vi "AO_master_DM_WFS_v1.vi"() -> ()   [LabVIEW 2018]
uses:
  <userlib>/WaveKit.lib/Controls/Image information.ctl
  <userlib>/WaveKit.lib/Controls/Image general information.ctl
  <userlib>/WaveKit.lib/Controls/Image acquisition information.ctl
  <userlib>/WaveKit.lib/Controls/Point2D.ctl
  <userlib>/WaveKit.lib/Controls/Data alignment enum.ctl
  <userlib>/WaveKit.lib/Controls/StatisticsData.ctl
  <userlib>/WaveKit.lib/Controls/Wavefront Corrector states - ONE.ctl
  <userlib>/WaveKit.lib/Classes/Camera/Camera.lvclass
  <userlib>/WaveKit.lib/Classes/CameraSet/CameraSet.lvclass
  <userlib>/WaveKit.lib/Classes/Image/Image.lvclass
  <userlib>/WaveKit.lib/Classes/Phase/Phase.lvclass
  <userlib>/WaveKit.lib/Controls/HasoSlopes.lvclass
  <userlib>/WaveKit.lib/Controls/Pupil.lvclass
  <userlib>/WaveKit.lib/Classes/WavefrontCorrector/WavefrontCorrector.lvclass
  <userlib>/WaveKit.lib/Classes/WavefrontCorrectorSet/WavefrontCorrectorSet.lvclass
  <userlib>/WaveKit.lib/Classes/HasoEngine/HasoEngine.lvclass
  <userlib>/WaveKit.lib/Controls/SlopesEngineSetup.ctl
  <userlib>/WaveKit.lib/Controls/WavefrontReconstructionMode.ctl
  <vilib>/Utility/file.llb/Read From Spreadsheet File (DBL).vi
  <vilib>/Analysis/1siggen.llb/Ramp Pattern by Delta.vi
  <userlib>/WaveKit.lib/Classes/ModalCoef/ModalCoef.lvclass
  <vilib>/Analysis/NI_AALBase.lvlib
panel:
  in  "Device Status":enum32{"DM", "WFS", "Others"}(tab)=enum."Others"
  out "DM Actuator Values":sgl[](graph)
  out "Initial State":T1[](array[typedef])
  out "ActuatorsNumber":i32
  out "Initial Positions":sgl[](array[numeric])
  out "Final Positions":sgl[](array[numeric])
  in  "Coef Min":dbl=-0.5 min=1.0
  in  "Coef Max":dbl=0.5 min=1.0
  out "Zernike Measured":dbl[](graph)
  out "Phase statistics":T2
  out "Phase values":sgl[][](graph)=[[nan, nan, nan, nan, nan, nan, nan, nan, nan, nan, nan, nan, nan, nan, nan, nan, nan, nan, nan, nan, nan, nan, nan, nan, nan, nan, nan, nan, nan, nan, nan, nan, nan, nan, nan, nan, nan, nan, nan, nan], [nan, nan, nan, nan, nan, nan, nan, nan, nan, nan, nan, nan, nan, nan, nan, nan, nan, nan, nan, nan, nan, nan, nan, nan, nan, nan, nan, nan, nan, nan, nan, nan, nan, nan, nan, nan, nan, nan, nan, nan], [nan, nan, nan, nan, nan, nan, nan, nan, nan, nan, nan, nan, nan, nan, nan, nan, nan, nan, nan, nan, nan, nan, nan, nan, nan, nan, nan, nan, nan, nan, nan, nan, nan, nan, nan, nan, nan, nan, nan, nan], [nan, nan, nan, nan, nan, nan, nan, nan, nan, nan, nan, nan, nan, nan, nan, nan, nan, nan, nan, nan, nan, nan, nan, nan, nan, nan, nan, nan, nan, nan, nan, nan, nan, nan, nan, nan, nan, nan, nan, nan], [nan, nan, nan, nan, nan, nan, nan, nan, nan, nan, nan, nan, nan, nan, -0.14441992, nan, 0.1501734, 0.22490476, 0.2674259, 0.28415325, 0.2792031, 0.2552752, 0.21375881, 0.15405469, nan, nan, nan, nan, nan, nan, nan, nan, nan, nan, nan, nan, nan, nan, nan, nan], [nan, nan, nan, nan, nan, nan, nan, nan, nan, nan, nan, nan, nan, nan, 0.19143742, 0.2795512, 0.33646506, 0.37099743, 0.3877919, 0.3894302, 0.37774685, 0.35447162, 0.3212538, 0.27904776, 0.22675864, 0.15897867, nan, nan, nan, nan, nan, nan, nan, nan, nan, nan, nan, nan, nan, nan], [nan, nan, nan, nan, nan, nan, nan, nan, nan, nan, nan, nan, nan, 0.22618562, 0.290776, 0.33285964, 0.36044422, 0.3767934, 0.38285175, 0.37884915, 0.3652757, 0.3433441, 0.3149789, 0.28229773, 0.2464756, 0.20580466, 0.15268901, 0.06923797, nan, nan, nan, nan, nan, nan, nan, nan, nan, nan, nan, nan], [nan, nan, nan, nan, nan, nan, nan, nan, nan, nan, nan, nan, 0.19992779, 0.24616541, 0.27565512, 0.29675642, 0.31222007, 0.32191983, 0.32467726, 0.31943765, 0.30597392, 0.2852214, 0.25927368, 0.2309889, 0.20308714, 0.17653626, 0.14795627, 0.10568966, 0.024115691, nan, nan, nan, nan, nan, nan, nan, nan, nan, nan, nan], [nan, nan, nan, nan, nan, nan, nan, nan, nan, nan, nan, 0.14862825, 0.18219855, 0.20114602, 0.21551609, 0.22862102, 0.24014233, 0.24817906, 0.2505626, 0.24567793, 0.23295718, 0.21313797, 0.18829979, 0.16161954, 0.1367108, 0.11633411, 0.10019377, 0.081457645, 0.04156301, -0.057204023, nan, nan, nan, nan, nan, nan, nan, nan, nan, nan], [nan, nan, nan, nan, nan, nan, nan, nan, nan, nan, 0.08899155, 0.117771566, 0.12948777, 0.13732892, 0.14631097, 0.15688494, 0.16728252, 0.17497937, 0.17758016, 0.17335457, 0.16157834, 0.14275661, 0.11873307, 0.09261118, 0.06834036, 0.04974218, 0.038678437, 0.031985473, 0.016725859, -0.03676957, nan, nan, nan, nan, nan, nan, nan, nan, nan, nan], [nan, nan, nan, nan, nan, nan, nan, nan, nan, nan, 0.058377307, 0.069048055, 0.0725615, 0.07683456, 0.0840318, 0.09335055, 0.10271386, 0.1097376, 0.11226265, 0.10867052, 0.09812171, 0.08078306, 0.058033932, 0.032565817, 0.008214329, -0.010712444, -0.020921554, -0.022825297, -0.02489755, -0.05023362, -0.14592764, nan, nan, nan, nan, nan, nan, nan, nan, nan], [nan, nan, nan, nan, nan, nan, nan, nan, nan, -0.0018393314, 0.018310271, 0.023098737, 0.024714457, 0.027986258, 0.033823933, 0.041292578, 0.048749834, 0.054400377, 0.056548227, 0.05374936, 0.04499338, 0.029967438, 0.009379062, -0.014759185, -0.03905803, -0.059140373, -0.070816256, -0.0724436, -0.06894927, -0.07806298, -0.1393881, nan, nan, nan, nan, nan, nan, nan, nan, nan], [nan, nan, nan, nan, nan, nan, nan, nan, nan, -0.03322208, -0.017045017, -0.0123043535, -0.010394985, -0.007970343, -0.0042642877, 0.0003761826, 0.005164365, 0.009095938, 0.010986101, 0.009512841, 0.0033822758, -0.008344227, -0.02579559, -0.047820807, -0.071688615, -0.09321856, -0.107681155, -0.11187886, -0.10789668, -0.10908524, -0.14891545, -0.29341945, nan, nan, nan, nan, nan, nan, nan, nan], [nan, nan, nan, nan, nan, nan, nan, nan, nan, nan, -0.043187555, -0.03622458, -0.033755217, -0.03278728, -0.03198469, -0.030707732, -0.028716512, -0.026208155, -0.023933899, -0.023217455, -0.025771504, -0.03328519, -0.04682974, -0.06620631, -0.08943447, -0.1126552, -0.13079928, -0.13944486, -0.13836564, -0.13734597, -0.16491348, -0.2807172, nan, nan, nan, nan, nan, nan, nan, nan], [nan, nan, nan, nan, nan, nan, nan, nan, -0.13038255, -0.08328184, -0.060542934, -0.050779276, -0.048053104, -0.048984695, -0.05126809, -0.053124577, -0.05330209, -0.051303368, -0.04760214, -0.04368073, -0.041799206, -0.04448101, -0.05377527, -0.07043236, -0.09320336, -0.118551016, -0.14113419, -0.15550357, -0.15952203, -0.16009864, -0.18189941, -0.27977645, nan, nan, nan, nan, nan, nan, nan, nan], [nan, nan, nan, nan, nan, nan, nan, nan, -0.15416794, -0.09987456, -0.07151361, -0.05893044, -0.056102008, -0.058817875, -0.063637674, -0.067669004, -0.06878706, -0.06599128, -0.059670344, -0.051622536, -0.044753395, -0.042448726, -0.04769562, -0.062100213, -0.08502676, -0.11315687, -0.14084403, -0.16171429, -0.1720384, -0.17647736, -0.19687745, -0.284868, -0.53908885, -1.12795, nan, nan, nan, nan, nan, nan], [nan, nan, nan, nan, nan, nan, nan, nan, -0.17633308, -0.1131372, -0.07876157, -0.06330658, -0.060116876, -0.063924976, -0.07015394, -0.07493687, -0.07548633, -0.07052183, -0.060539607, -0.047784284, -0.035856243, -0.028966732, -0.030924596, -0.044017438, -0.06802279, -0.099662215, -0.13288532, -0.16044727, -0.17731819, -0.18653797, -0.20820689, -0.29237592, -0.5366785, nan, nan, nan, nan, nan, nan, nan], [nan, nan, nan, nan, nan, nan, nan, nan, -0.19826387, -0.12505035, -0.08430402, -0.06564974, -0.061443567, -0.06527472, -0.07152294, -0.07554153, -0.07411167, -0.0658889, -0.05163869, -0.034133032, -0.017655006, -0.0071354215, -0.007018423, -0.020031396, -0.046107426, -0.08178567, -0.12048963, -0.15415914, -0.17678727, -0.19048853, -0.21480094, -0.2999987, -0.54526997, nan, nan, nan, nan, nan, nan, nan], [nan, nan, nan, nan, nan, nan, nan, nan, -0.2214154, -0.13693352, -0.08914254, -0.06661926, -0.06048554, -0.06317037, -0.0681367, -0.07015528, -0.065784656, -0.053790003, -0.035310905, -0.013662348, 0.0062713036, 0.01901285, 0.01972933, 0.005542416, -0.023349542, -0.06307545, -0.10643376, -0.14466219, -0.17119798, -0.18806857, -0.21562657, -0.30642, -0.5640642, nan, nan, nan, nan, nan, nan, nan], [nan, nan, nan, nan, nan, nan, nan, nan, -0.24718054, -0.14940841, -0.093277775, -0.0658183, -0.056708053, -0.05720259, -0.059951056, -0.05929426, -0.051715773, -0.036192447, -0.014265999, 0.010266874, 0.032073133, 0.04536258, 0.04520398, 0.028878966, -0.0030008797, -0.045963787, -0.092160165, -0.13235793, -0.16002774, -0.17817038, -0.20961209, -0.31157303, -0.5953845, nan, nan, nan, nan, nan, nan, nan], [nan, nan, nan, nan, nan, nan, nan, nan, -0.27748746, -0.16290864, -0.09610232, -0.062047683, -0.048735943, -0.04617936, -0.046241976, -0.042900223, -0.03261665, -0.014586102, 0.009311387, 0.03494107, 0.05674191, 0.068891875, 0.0666744, 0.04783368, 0.0136316735, -0.030755527, -0.0769404, -0.115639456, -0.14119013, -0.15893419, -0.19620675, -0.31774768, nan, nan, nan, nan, nan, nan, nan, nan], [nan, nan, nan, nan, nan, nan, nan, nan, -0.31623095, -0.17884897, -0.09729818, -0.0539262, -0.03469713, -0.028198741, -0.025418447, -0.019910373, -0.008048305, 0.010862423, 0.034768496, 0.05942371, 0.07931873, 0.0889112, 0.08400761, 0.06307276, 0.028166434, -0.014867521, -0.057410896, -0.09080534, -0.111413695, -0.12868427, -0.17697167, -0.3319423, nan, nan, nan, nan, nan, nan, nan, nan], [nan, nan, nan, nan, nan, nan, nan, nan, nan, -0.20170604, -0.09850275, -0.0411539, -0.0131010795, -0.0011654077, 0.0047943285, 0.01185911, 0.023955166, 0.041901454, 0.06374147, 0.08542206, 0.1018104, 0.10796184, 0.10047772, 0.0787158, 0.04554086, 0.007227666, -0.027947046, -0.052963093, -0.06777905, -0.08820889, -0.15871821, nan, nan, nan, nan, nan, nan, nan, nan, nan], [nan, nan, nan, nan, nan, nan, nan, nan, nan, -0.24239759, -0.10614249, -0.026831074, 0.015322472, 0.03581071, 0.046350636, 0.05505173, 0.06651187, 0.08204405, 0.10016226, 0.11737824, 0.12928592, 0.13183476, 0.12261822, 0.10192663, 0.073240966, 0.042765103, 0.017522467, 0.0014635092, -0.0110412, -0.045025453, -0.15884721, nan, nan, nan, nan, nan, nan, nan, nan, nan], [nan, nan, nan, nan, nan, nan, nan, nan, nan, nan, -0.13597216, -0.021381527, 0.04426403, 0.07956008, 0.09847209, 0.110732496, 0.122154154, 0.13505057, 0.14887714, 0.16113368, 0.16849175, 0.16803522, 0.1584293, 0.14075197, 0.118653886, 0.09743117, 0.0815231, 0.06987105, 0.048498146, -0.020404778, nan, nan, nan, nan, nan, nan, nan, nan, nan, nan], [nan, nan, nan, nan, nan, nan, nan, nan, nan, nan, nan, -0.04876471, 0.05625415, 0.117832564, 0.15310521, 0.17423762, 0.18897903, 0.20128381, 0.21210447, 0.22038196, 0.22418612, 0.221881, 0.21311647, 0.19937092, 0.1836943, 0.16922635, 0.15598845, 0.13537171, 0.081669986, nan, nan, nan, nan, nan, nan, nan, nan, nan, nan, nan], [nan, nan, nan, nan, nan, nan, nan, nan, nan, nan, nan, nan, 0.014031529, 0.121263236, 0.18738765, 0.22803904, 0.25380248, 0.2710389, 0.28282017, 0.2899857, 0.29225817, 0.2892868, 0.28139976, 0.26978248, 0.25571787, 0.23844866, 0.21115, 0.15442081, nan, nan, nan, nan, nan, nan, nan, nan, nan, nan, nan, nan], [nan, nan, nan, nan, nan, nan, nan, nan, nan, nan, nan, nan, nan, nan, 0.15212902, 0.2306162, 0.28129596, 0.31381333, 0.33402625, 0.3450995, 0.34855807, 0.34515002, 0.33529556, 0.31882071, 0.29360068, 0.25266168, nan, nan, nan, nan, nan, nan, nan, nan, nan, nan, nan, nan, nan, nan], [nan, nan, nan, nan, nan, nan, nan, nan, nan, nan, nan, nan, nan, nan, nan, nan, 0.1979487, 0.2623494, 0.30271748, 0.32490522, 0.33223343, 0.3261181, 0.30614072, 0.26925305, nan, nan, nan, nan, nan, nan, nan, nan, nan, nan, nan, nan, nan, nan, nan, nan], [nan, nan, nan, nan, nan, nan, nan, nan, nan, nan, nan, nan, nan, nan, nan, nan, nan, nan, nan, nan, nan, nan, nan, nan, nan, nan, nan, nan, nan, nan, nan, nan, nan, nan, nan, nan, nan, nan, nan, nan], [nan, nan, nan, nan, nan, nan, nan, nan, nan, nan, nan, nan, nan, nan, nan, nan, nan, nan, nan, nan, nan, nan, nan, nan, nan, nan, nan, nan, nan, nan, nan, nan, nan, nan, nan, nan, nan, nan, nan, nan], [nan, nan, nan, nan, nan, nan, nan, nan, nan, nan, nan, nan, nan, nan, nan, nan, nan, nan, nan, nan, nan, nan, nan, nan, nan, nan, nan, nan, nan, nan, nan, nan, nan, nan, nan, nan, nan, nan, nan, nan]] caption="Wavefront"
  out "HASO intensity":u32[][](graph)
  in  "error in (no error)":errorcluster
  out "Current error":errorcluster
  out "Output path":path=path "D:/Data"
  out "nb_images (get)":u32=10
  out "exposure_duration_us (get)":u32
  in  "Current status":string="Test1"
  out "HASO ready":bool
  in  "Live Wavefront":bool
  in  "Update DM":bool
  in  "Tab Control":T3(tab)
  in  "Initial haso file":path=path "D:/SystemAlignment/system_aberration_residual_20220406.has"
  in  "interaction matrix file":path=path "D:/SystemAlignment/IM_20220407_1p5sx2_0p5um.aomi"
  in  "DM configuration file":path=path "C:/Program Files (x86)/Imagine Optic/Configuration Files/WaveFrontCorrector_mirao52-e_0326.dat"
  in  "Haso configuration file":path=path "C:/Program Files (x86)/Imagine Optic/Configuration Files/HASO3_first_7364.dat"
  in  "Record Batch Actuator":bool
  in  "Coef value":dbl=0.5 min=1.0
  in  "Idx end":u32=20 min=1
  in  "Idx start":u32=1 min=1
  in  "Subfolder":string="Test1"
  in  "Folder Name":string="Test"
  in  "Net Rp":bool
  in  "Input type":T4(ring)=enum."Zernike Coef"
  in  "Additional Command":bool=TRUE
  in  "Offset command file":path=path "D:/SystemAlignment/system_aberration_20220414.dat"
  in  "Initial offset":bool=TRUE
  in  "Additional file":path=path "D:/SystemAlignment/system_aberration_20191029.dat"
  out "Coef out":sgl[](array[numeric])
  out "Index out":i32[](array[numeric])
  in  "Zern/DM index in":i32[](array[numeric])
  in  "Zern/DM coef in":sgl[](array[numeric])
  in  "idxType":enum16{"Wyant", "ANSI"}(ring)=enum."ANSI"
  in  "Filter":u8[](array[numeric])
  in  "exposure_duration_s (set)":dbl=1.0 min=1.0
  in  "nb_images (set)":u32=1 min=1
  in  "Save File":bool
  in  "File Base Name":string="Test"
  in  "Main Path":path=path "D:/Data"
  in  "Record Response":bool
  in  "Record Batch Zern":bool
  out "Acquisition information":T5={"Image general information"={"Camera serial number"="", "Smearing removed"=FALSE, "Background image removed"=FALSE, "Time Stamp"=timestamp(0 s since 1904-01-01), "Comment"="", "Camera_MAX_Level"=0}, "Acquisition information"={"Exposure duration (us)"=0, "Exposure duration specified (us)"=0, "Gain"=0.0, "Number of summed images"=0, "Trigger type"=""}, "Number of pixels"={"X"=0, "Y"=0}, "Number of bits"=enum."16"}
  in  "Init":bool
  in  "Reset error":bool
  in  "Exit":bool
  in  "Stop HASO":bool
  in  "Start HASO":bool
  # "AO_master_DM_WFS_v1.vi: (last update: 20220405)\nControl deformable mirror and wavefront sensor, check DM response \n1, re-orgnize panel/interface: tap for settings, tab for display and indicators\n2, change camera asynchronous mode to synchronous mode:  see xxxx_v1_SynModeFailure_discarded.vi \n      tried but it does not work when exp time < 0.1s (?), switched back to asyn mode.\n3, add control to flip mirror ( and laser shutter and stage ???): to do\n4, make it more efficient and robust to errors (now: error --> shut down devices)\na) DM ocuppied due to last unnormal exit; b) wavefront measure error: no laser, wrong slopes;\n5, enable DM input by actuators, add DM  actuator index picture, check response of actuators in batch"
  # "Stop HASO: error after Record Batch"
  # "um"
  # "HASO Parameters"
  # "Need to turn OFF live wavefront"
  # "Check DM Response"
  # "Batch Range"
  # "Show in Wyant convention"
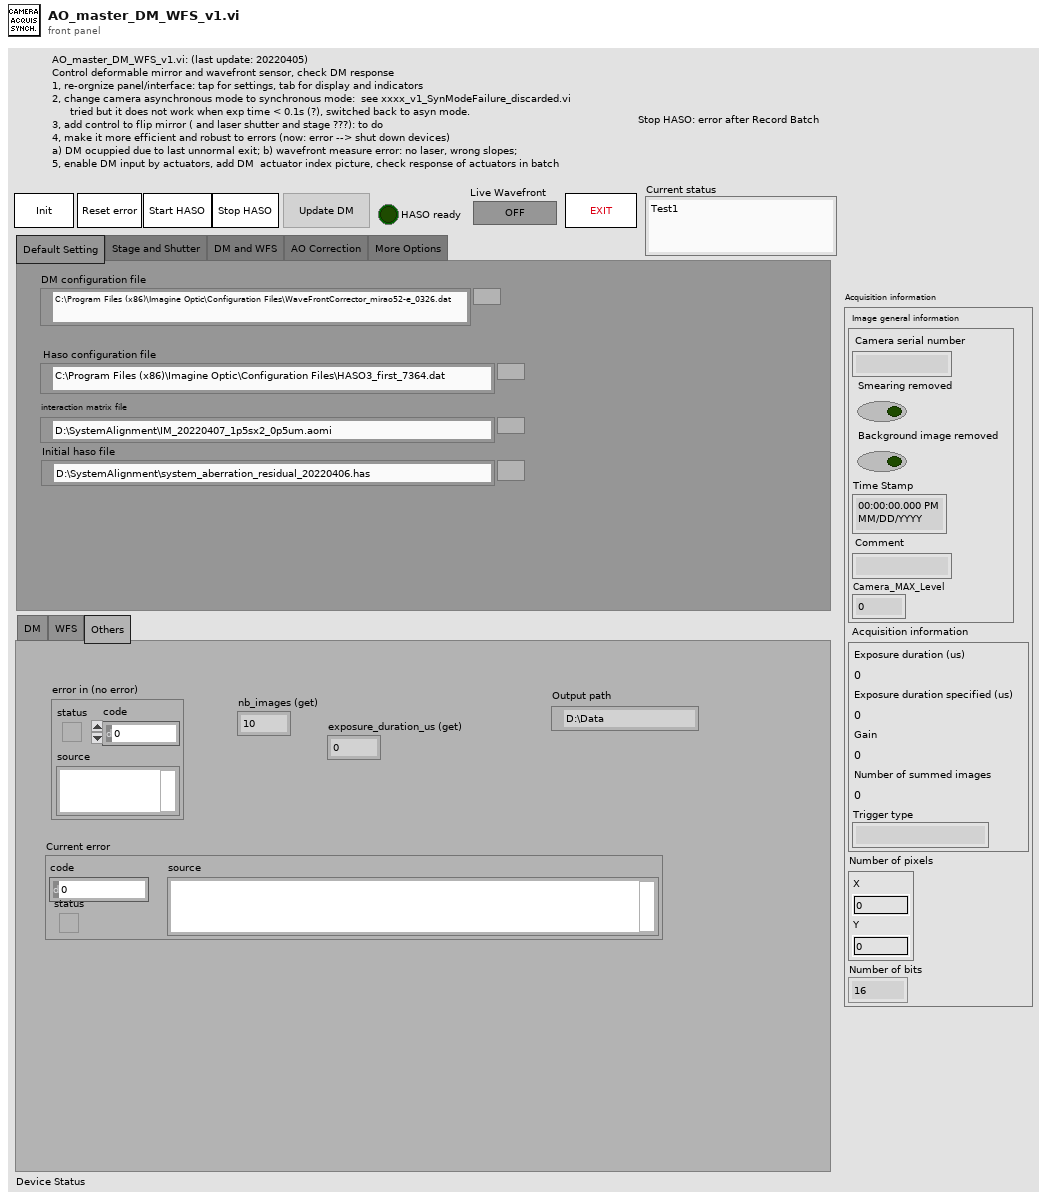
[diagram p1: front panel]
types:
  T1 = typedef "Wavefront Corrector states - ONE.ctl" = cluster{"Max":sgl, "Min":sgl, "Validity":enum16{"valid", "fixed", "invalid"}, "Fixed_Position":sgl}
  T2 = typedef "StatisticsData.ctl" = cluster{"PV":sgl, "RMS":dbl, "Max":sgl, "Min":sgl}
  T3 = enum32{"Default Setting", "Stage and Shutter", "DM and WFS", "AO Correction", "More Options"}
  T4 = enum16{"Zero Input", "Command File", "Zernike Coef", "Zernike File", "DM actuators"}
  T5 = typedef "Image information.ctl" = cluster{"Image general information":T6, "Acquisition information":T7, "Number of pixels":T8, "Number of bits":T9}
  T6 = typedef "Image general information.ctl" = cluster{"Camera serial number":string, "Smearing removed":bool, "Background image removed":bool, "Time Stamp":timestamp, "Comment":string, "Camera_MAX_Level":i32}
  T7 = typedef "Image acquisition information.ctl" = cluster{"Exposure duration (us)":i32, "Exposure duration specified (us)":i32, "Gain":sgl, "Number of summed images":i32, "Trigger type":string}
  T8 = typedef "Point2D.ctl" = cluster{"X":u32, "Y":u32}
  T9 = typedef "Data alignment enum.ctl" = enum16{"8", "16", "32"}
  T10 = typedef "SlopesEngineSetup.ctl" = cluster{"Start sub-aperture":T8, "Pupil average":dbl}
  T11 = typedef "CameraSpecifications.ctl" = cluster{"Grabber name":string, "Camera name":string, "Camera sn":string, "Pixels_um":T12, "Maximum level":u32, "Data alignment":T9, "Is signed":bool, "Acquisition start":T8, "Acquisition length":T8, "MaxFrameRate_Hz":sgl, "Chip type":enum16{"Progressive scan", "Frame transfert"}}
  T12 = typedef "General dimensions definition.ctl" = cluster{"Size":T8, "Step":T13}
  T13 = typedef "Point2Df.ctl" = cluster{"X":sgl, "Y":sgl}
  T14 = typedef "Wavefront Corrector Position.ctl" = sgl[]
  T15 = typedef "WavefrontReconstructionMode.ctl" = enum16{"None", "Modal_Legendre", "Modal_Zernike", "Zonal", "Modal_Zonal_Zernike", "Modal_Zonal_Legendre"}
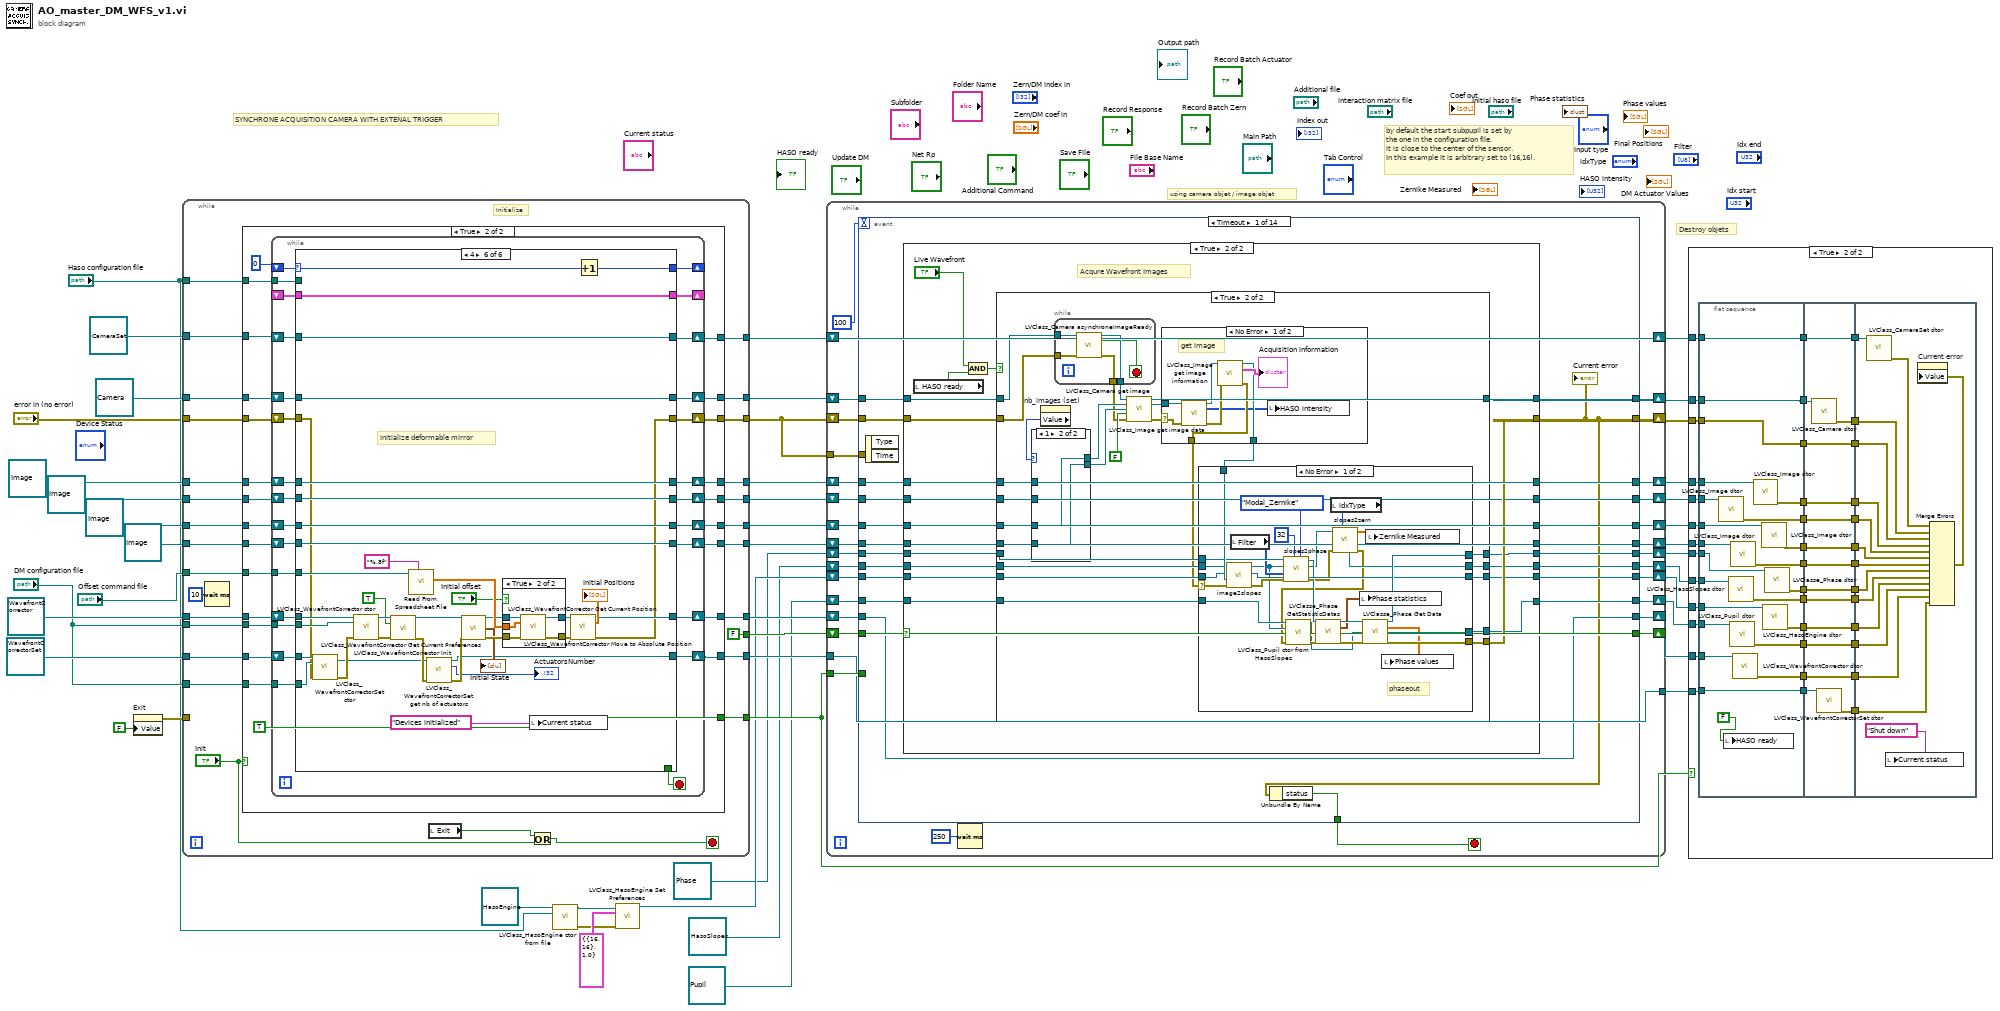
[diagram p0: block diagram]
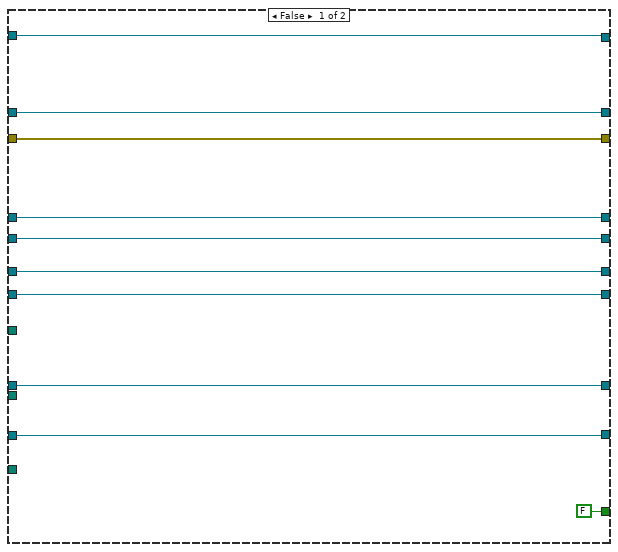
[diagram p3: hidden frame]
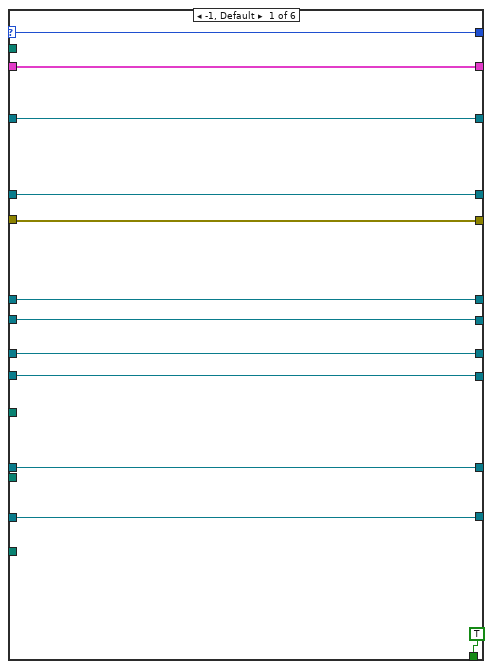
[diagram p4: hidden frame]
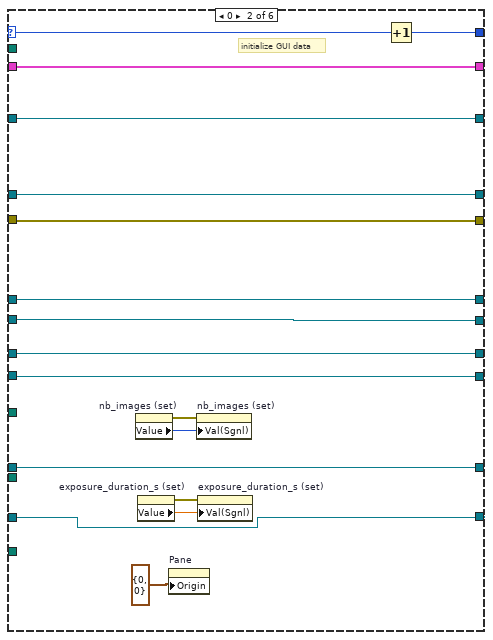
[diagram p5: hidden frame]
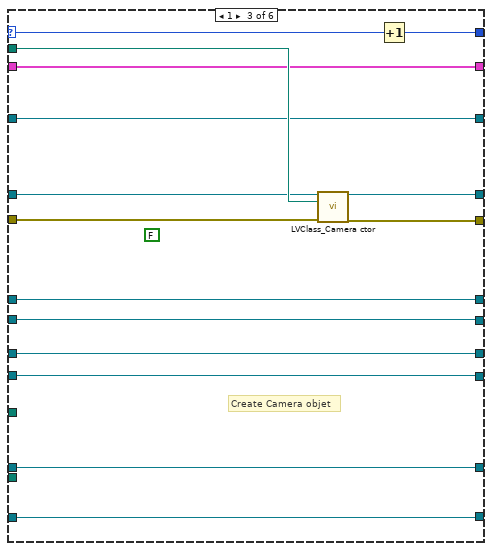
[diagram p6: hidden frame]
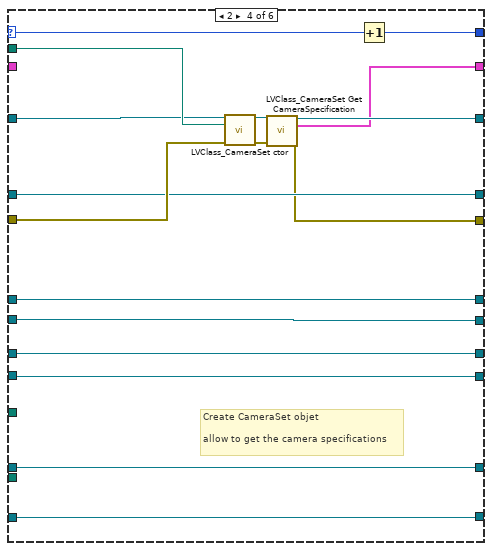
[diagram p7: hidden frame]
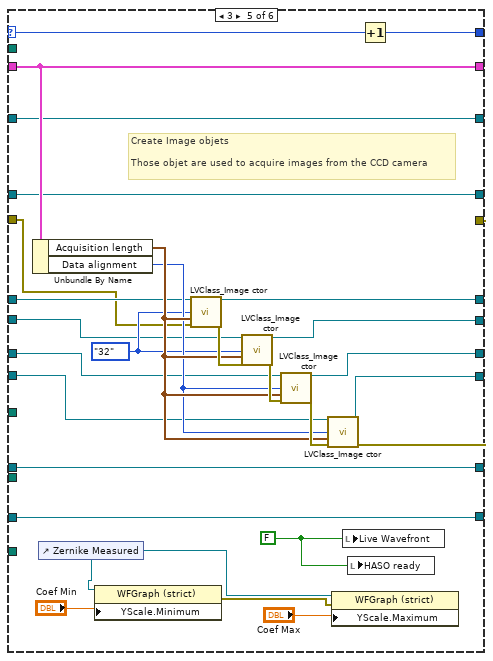
[diagram p8: hidden frame]
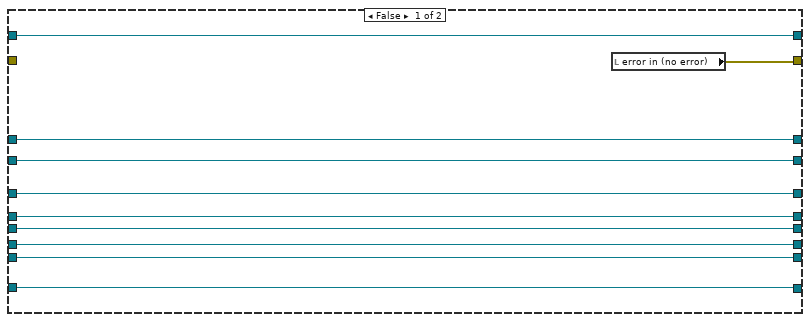
[diagram p10: hidden frame]
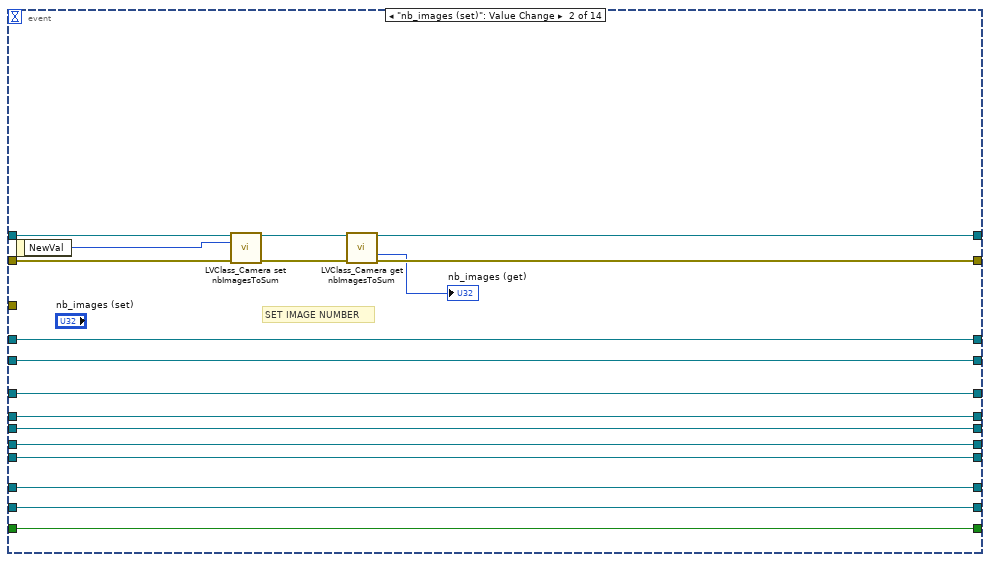
[diagram p15: hidden frame]
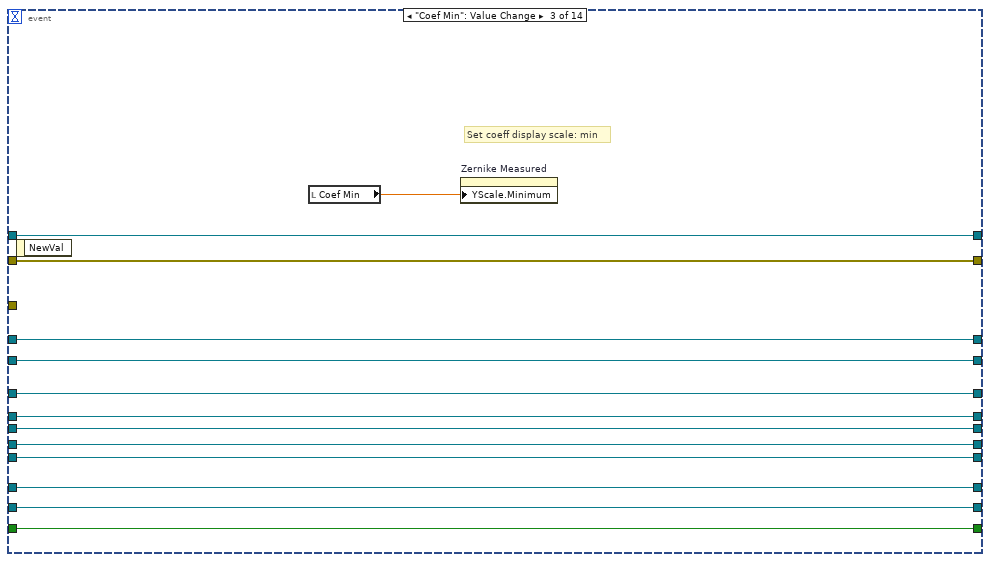
[diagram p16: hidden frame]
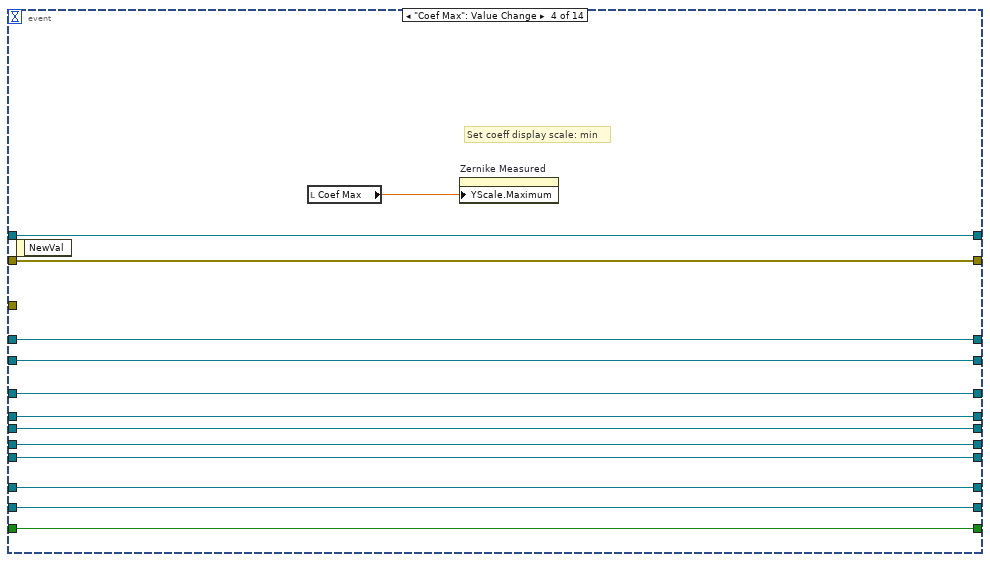
[diagram p17: hidden frame]
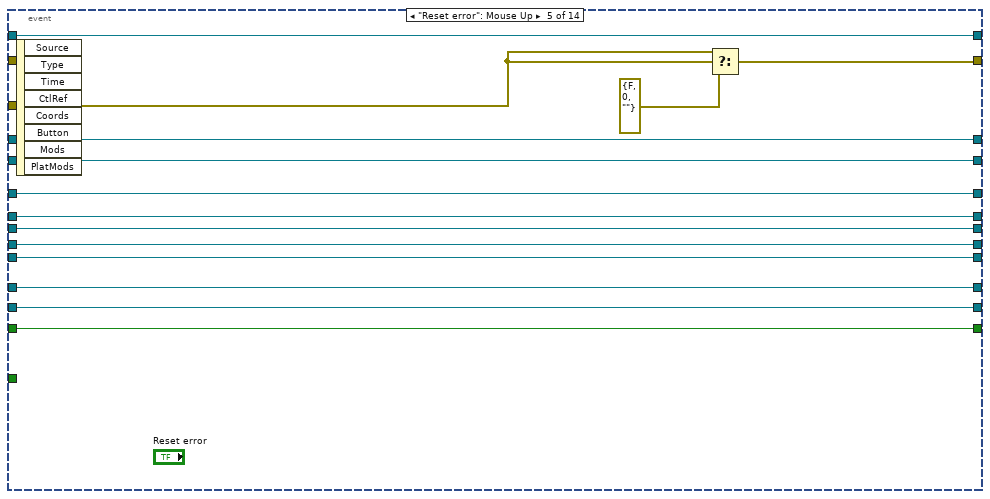
[diagram p18: hidden frame]
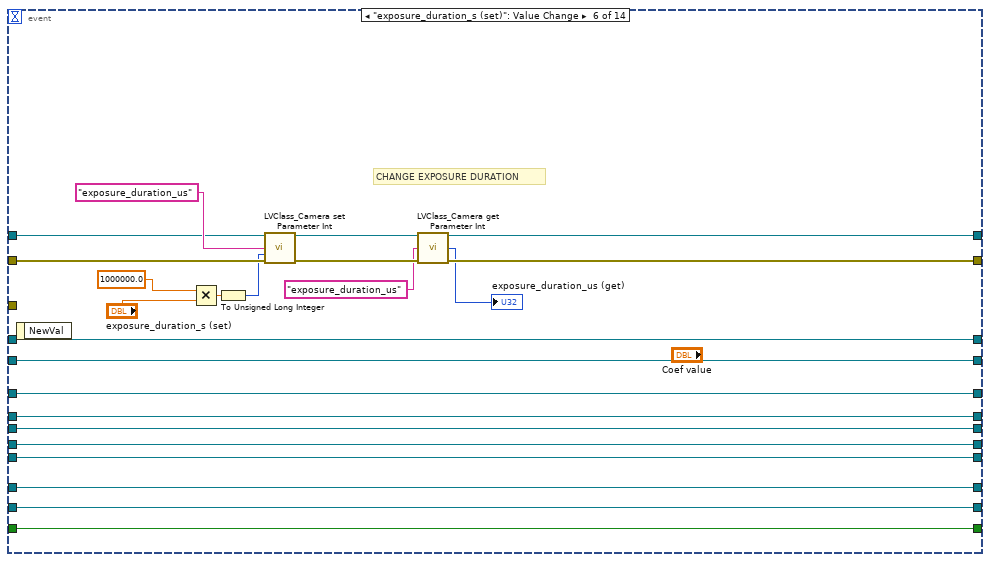
[diagram p19: hidden frame]
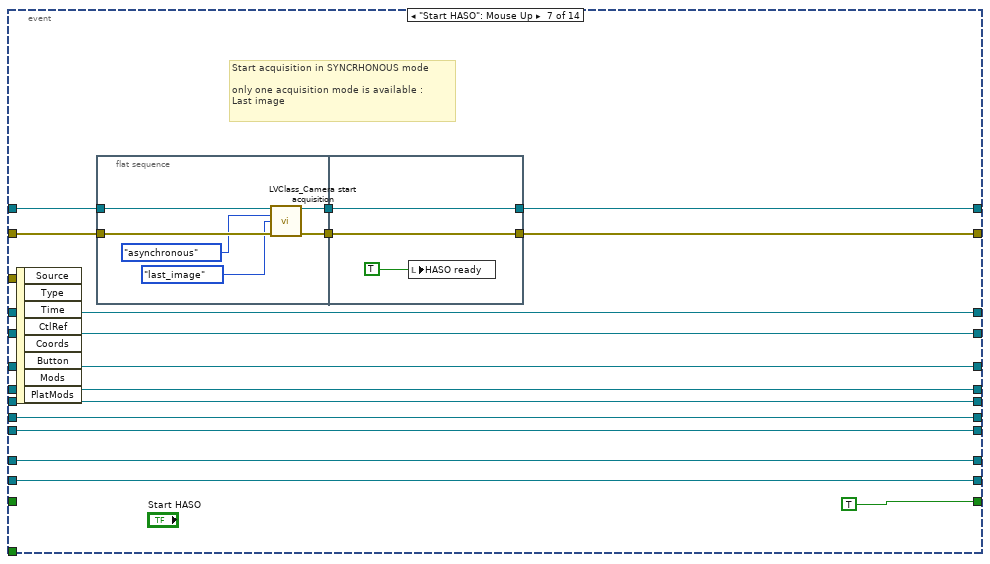
[diagram p20: hidden frame]
diagram:
  # "by default the start subpupil is set by \nthe one in the configuration file. \nit is close to the center of the sensor.\nIn this example it is arbitrary set to (16,16)."
  # "Destroy objets"
  # "using camera objet / image objet"
  # "SYNCHRONE ACQUISITION CAMERA WITH EXTENAL TRIGGER"
  n1 = property on="Exit" class="Bool (strict)"("Value"=FALSE ("Exit")) -> (error out=w23:errorcluster)  [unwired: 2 in, 1 out]
  n2 = while {
    tunnel: [FALSE] -> w39
    tunnel: [w73] -> w38
    tunnel: [w72] -> w37
    tunnel: [w71] -> w36
    tunnel: [w70] -> w35
    tunnel: [w69] -> w34
    tunnel: [w68] -> w33
    tunnel: refnum<class "Camera.lvclass"> refnum ("Camera.lvclass") -> [w67]
    tunnel: refnum<class "CameraSet.lvclass"> refnum ("CameraSet.lvclass") -> [w66]
    tunnel: refnum<class "Image.lvclass"> refnum ("Image in") -> [w65]
    tunnel: refnum<class "Image.lvclass"> refnum ("Image in") -> [w64]
    tunnel: refnum<class "Image.lvclass"> refnum ("Image in") -> [w63]
    tunnel: refnum<class "Image.lvclass"> refnum ("Image in") -> [w62]
    tunnel: "error in (no error)" -> [w61]
    tunnel: [w60] -> w26
    tunnel: [w58] -> w25
    tunnel: w23 -> [_]
    tunnel: "Haso configuration file" -> [w54]
    tunnel: "Offset command file" -> [w53]
    tunnel: refnum<class "WavefrontCorrectorSet.lvclass"> refnum ("WavefrontCorrectorSet in") -> [w52]
    tunnel: "DM configuration file" -> [w51]
    tunnel: refnum<class "WavefrontCorrector.lvclass"> refnum ("WavefrontCorrector in") -> [w50]
    tunnel: "DM configuration file" -> [w49]
    tunnel: [w48] -> w18
    tunnel: [w47] -> w17
    stop <- w55 stop-if-true
    # "Initialize"
    n3 = Wait (ms)(milliseconds to wait=u32 10) -> ()  [unwired: 1 out]
    n4 = case shown="True" "Init" {
      tunnel: [w84 w108] -> w73
      tunnel: [w83 w107] -> w72
      tunnel: [w81 w106] -> w71
      tunnel: [w80 w105] -> w70
      tunnel: [w79 w104] -> w69
      tunnel: [w78 w103] -> w68
      tunnel: w67 -> [w84 w102]
      tunnel: w66 -> [w83 w100]
      tunnel: w65 -> [w81 w99]
      tunnel: w64 -> [w80 w98]
      tunnel: w63 -> [w79 w97]
      tunnel: w62 -> [w78 w96]
      tunnel: w61 -> [w82 w95]
      tunnel: [w82 w94] -> w60
      tunnel: [FALSE TRUE] -> w58
      tunnel: w54 -> [_ w92]
      tunnel: w53 -> [_ w91]
      tunnel: w52 -> [w75 w85]
      tunnel: w51 -> [_ w90]
      tunnel: w50 -> [w76 w86]
      tunnel: w49 -> [_ w89]
      tunnel: [w76 w88] -> w48
      tunnel: [w75 w87] -> w47
      frame False {
      }
      frame True {
        n5 = while {
          tunnel: w92 -> [w133]
          shift-right: [w135] -> w108
          shift-left: w102 -> [w127]
          shift-right: [w117] -> _
          shift-left: 0 -> [w116]
          shift-right: [w134] -> w107
          shift-left: w100 -> [w126]
          shift-right: [w125] -> _
          shift-left: _ -> [w123]
          shift-right: [w132] -> w106
          shift-left: w99 -> [w124]
          shift-right: [w131] -> w105
          shift-left: w98 -> [w122]
          shift-right: [w130] -> w104
          shift-left: w97 -> [w120]
          shift-right: [w129] -> w103
          shift-left: w96 -> [w121]
          shift-right: [w128] -> w94
          shift-left: w95 -> [w118]
          tunnel: w91 -> [w115]
          tunnel: w90 -> [w114]
          tunnel: w89 -> [w113]
          shift-right: [w112] -> w88
          shift-left: w86 -> [w110]
          shift-right: [w111] -> w87
          shift-left: w85 -> [w109]
          stop <- w119 stop-if-true
          n6 = case shown="4" w116 {
            tunnel: [w147 w151 w179 w189 w211 w261] -> w135
            tunnel: w133 -> [_ _ w178 w193 _ _]
            tunnel: [w146 w155 w176 w194 w212 w260] -> w134
            tunnel: [w139 w156 w170 w184 w218 w255] -> w132
            tunnel: [w140 w157 w171 w185 w217 w256] -> w131
            tunnel: [w141 w158 w172 w186 w216 w257] -> w130
            tunnel: [w142 w159 w173 w187 w215 w258] -> w129
            tunnel: [w143 w150 w175 w188 w214 w229] -> w128
            selector: w116 -> [w138 w153 w168 w183 w206 w227]
            tunnel: w127 -> [w147 w151 w177 w189 w211 w261]
            tunnel: w126 -> [w146 w155 w176 w192 w212 w260]
            tunnel: [w144 w152 w174 w191 w213 w259] -> w125
            tunnel: w124 -> [w139 w156 w170 w184 w210 w255]
            tunnel: w123 -> [w144 w152 w174 _ w213 w259]
            tunnel: w122 -> [w140 w157 w171 w185 w209 w256]
            tunnel: w121 -> [w142 w159 w173 w187 w208 w258]
            tunnel: w120 -> [w141 w158 w172 w186 w207 w257]
            tunnel: [TRUE _ _ _ _ _] -> w119
            tunnel: w118 -> [w143 w150 w167 w190 w204 w230]
            tunnel: [w138 w154 w169 w182 w205 w226] -> w117
            tunnel: w115 -> [_ _ _ _ _ w237]
            tunnel: w109 -> [w136 w148 w165 w180 w202 w235]
            tunnel: w114 -> [_ _ _ _ _ w234]
            tunnel: w110 -> [w137 w149 w166 w181 w203 w233]
            tunnel: w113 -> [_ _ _ _ _ w232]
            tunnel: [w137 w149 w166 w181 w203 w231] -> w112
            tunnel: [w136 w148 w165 w180 w202 w228] -> w111
            frame -1, Default {
            }
            frame 0 {
              # "initialize GUI data"
              n7 = property on="nb_images (set)" class="DigNum (strict)"() -> (error out=w164:errorcluster, "Value"=w163:u32)  [unwired: 2 in, 1 out]
              n8 = property on="exposure_duration_s (set)" class="DigNum (strict)"() -> (error out=w160:errorcluster, "Value"=w162:dbl)  [unwired: 2 in, 1 out]
              n9 = property on="Pane" class="Pane"("Origin"=cluster{"Horizontal":i16, "Vertical":i16} {"Horizontal"=0, "Vertical"=0} ("Front Panel Window:Origin")) -> ()  [unwired: 2 in, 2 out]
              n10 = property on="nb_images (set)" class="DigNum (strict)"(error in=w164, "Val(Sgnl)"=w163) -> ()  [unwired: 1 in, 2 out]
              n11 = property on="exposure_duration_s (set)" class="DigNum (strict)"(error in=w160, "Val(Sgnl)"=w162) -> ()  [unwired: 1 in, 2 out]
              n12 = Increment(x=w153) -> (x+1=w154:i32)
            }
            frame 1 {
              (unwired) FALSE ("Acq required")
              # "Create Camera objet"
              n13 = call <userlib>:"LVClass_Camera ctor.vi"("Camera"=w177, "Configuration file path"=w178, "error in (no error)"=w167) -> ("Camera (new)"=w179:refnum<class "Camera.lvclass">, "error out"=w175:errorcluster)  [unwired: 11 in]
              n14 = Increment(x=w168) -> (x+1=w169:i32)
            }
            frame 2 {
              # "Create CameraSet objet\n\nallow to get the camera specifications"
              n15 = call <userlib>:"LVClass_CameraSet ctor.vi"("CameraSet.lvclass"=w192, "Configuration file path"=w193, "error in (no error)"=w190) -> ("CameraSet.lvclass"=w196:refnum<class "CameraSet.lvclass">, "error out"=w195:errorcluster)  [unwired: 11 in]
              n16 = call <userlib>:"LVClass_CameraSet Get CameraSpecification.vi"("CameraSet.lvclass"=w196, "error in (no error)"=w195) -> ("CameraSet.lvclass"=w194:refnum<class "CameraSet.lvclass">, "Camera Config"=w191:T11, "error out"=w188:errorcluster)  [unwired: 11 in]
              n17 = Increment(x=w183) -> (x+1=w182:i32)
            }
            frame 3 {
              w201 = FALSE
              w219 = Data_alignment_enum."32" ("Data alignment")
              # "Create Image objets\n\nThose objet are used to acquire images from the CCD camera"
              n18 = Unbundle By Name(w213) -> ("Acquisition length"=w221:T8, "Data alignment"=w220:T9)
              n19 = control-ref of="Zernike Measured"() -> (w198:refnum<vi>)
              n20 = property on="Property Node" class="WFGraph (strict)"(reference=w198, "YScale.Minimum"="Coef Min") -> (error out=w197:errorcluster)  [unwired: 1 in, 1 out]
              n21 = call <userlib>:"LVClass_Image ctor.vi"("Image in"=w210, "Data alignment"=w219, "Size"=w221, "error in (no error)"=w204) -> ("Image out"=w218:refnum<class "Image.lvclass">, "error out"=w222:errorcluster)  [unwired: 10 in]
              n22 = call <userlib>:"LVClass_Image ctor.vi"("Image in"=w209, "Data alignment"=w219, "Size"=w221, "error in (no error)"=w222) -> ("Image out"=w217:refnum<class "Image.lvclass">, "error out"=w223:errorcluster)  [unwired: 10 in]
              n23 = call <userlib>:"LVClass_Image ctor.vi"("Image in"=w207, "Data alignment"=w220, "Size"=w221, "error in (no error)"=w223) -> ("Image out"=w216:refnum<class "Image.lvclass">, "error out"=w224:errorcluster)  [unwired: 10 in]
              n24 = call <userlib>:"LVClass_Image ctor.vi"("Image in"=w208, "Data alignment"=w220, "Size"=w221, "error in (no error)"=w224) -> ("Image out"=w215:refnum<class "Image.lvclass">, "error out"=w214:errorcluster)  [unwired: 10 in]
              n25 = property on="Property Node" class="WFGraph (strict)"(reference=w198, error in=w197, "YScale.Maximum"="Coef Max") -> ()  [unwired: 2 out]
              n26 = local write "Live Wavefront"(w201) -> ()
              n27 = local write "HASO ready"(w201) -> ()
              n28 = Increment(x=w206) -> (x+1=w205:i32)
            }
            frame 4 {
              (unwired) "DM "
              (unwired) "DM "
              # "Initialize deformable mirror"
              n29 = call <userlib>:"LVClass_WavefrontCorrectorSet ctor.vi"("WavefrontCorrectorSet in"=w235, "PathToWavefrontCorrectorSetupFile"=w234, "error in (no error)"=w230) -> ("WavefrontCorrectorSet out"=w242:refnum<class "WavefrontCorrectorSet.lvclass">, "error out"=w251:errorcluster)  [unwired: 11 in]
              n30 = call <userlib>:"LVClass_WavefrontCorrector ctor.vi"("WavefrontCorrector in"=w233, "PathToWavefrontCorrectorSetupFile"=w232, "error in (no error)"=w251) -> ("WavefrontCorrector out"=w239:refnum<class "WavefrontCorrector.lvclass">, "error out"=w240:errorcluster)  [unwired: 11 in]
              n31 = call <userlib>:"LVClass_WavefrontCorrector Init.vi"("WavefrontCorrector in"=w239, "set_init_state_from_config_file"=TRUE, "error in (no error)"=w240) -> ("WavefrontCorrector out"=w243:refnum<class "WavefrontCorrector.lvclass">, "error out"=w252:errorcluster)  [unwired: 11 in]
              n32 = call-poly <vilib>:"Read From Spreadsheet File.vi"("format (%.3f)"="%.8f", "file path (dialog if empty)"=w237) -> ("first row"=w254:dbl[])  [unwired: 5 in, 4 out]
              n33 = call <userlib>:"LVClass_WavefrontCorrectorSet get nb of actuators.vi"("WavefrontCorrectorSet in"=w242, "error in (no error)"=w252) -> ("WavefrontCorrectorSet out"=w228:refnum<class "WavefrontCorrectorSet.lvclass">, "ActuatorsNumber"=→"ActuatorsNumber":i32, "error out"=w253:errorcluster)  [unwired: 11 in]
              n34 = call <userlib>:"LVClass_WavefrontCorrector Get Current Preferences.vi"("WavefrontCorrector in"=w243, "error in (no error)"=w253) -> ("WavefrontCorrector out"=w248:refnum<class "WavefrontCorrector.lvclass">, "Mirror preferences.Wavefront Corrector State"=→"Initial State":T1[], "error out"=w249:errorcluster)  [unwired: 10 in, 1 out]
              n35 = case shown="True" "Initial offset" {
                tunnel: w254 -> [_ w268]
                tunnel: [w263 w267] -> w246
                tunnel: [w262 w266] -> w247
                tunnel: w248 -> [w263 w265]
                tunnel: w249 -> [w262 w264]
                frame False {
                }
                frame True {
                  n36 = call <userlib>:"LVClass_WavefrontCorrector Move to Absolute Position.vi"("WavefrontCorrector in"=w265, "Absolute Positions"=w268, "error in (no error)"=w264) -> ("WavefrontCorrector out"=w267:refnum<class "WavefrontCorrector.lvclass">, "error out"=w266:errorcluster)  [unwired: 11 in]
                }
              }
              n37 = local write "Current status"("Devices initialized") -> ()
              n38 = call <userlib>:"LVClass_WavefrontCorrector Get Current Position.vi"("WavefrontCorrector in"=w246, "error in (no error)"=w247) -> ("WavefrontCorrector out"=w231:refnum<class "WavefrontCorrector.lvclass">, "Wavefront Corrector Position"=→"Initial Positions":T14, "error out"=w229:errorcluster)  [unwired: 11 in]
              n39 = Increment(x=w227) -> (x+1=w226:i32)
            }
          }
        }
      }
    }
    n40 = local read "Exit"() -> (w57:bool)
    n41 = Or(x=w57, y="Init") -> (x .or. y?=w55:bool)
  }
  n42 = call <userlib>:"LVClass_HasoEngine ctor from file.vi"("HasoEngine in"=refnum<class "HasoEngine.lvclass"> refnum, "Configuration file path"="Haso configuration file") -> ("HasoEngine out"=w14:refnum<class "HasoEngine.lvclass">, "error out"=w15:errorcluster)  [unwired: 12 in]
  n43 = call <userlib>:"LVClass_HasoEngine Set Preferences.vi"("HasoEngine in"=w14, "Slopes_HasoEngine_Setup"=T10 {"Start sub-aperture"={"X"=16, "Y"=16}, "Pupil average"=1.0}, "error in (no error)"=w15) -> ("HasoEngine out"=w11:refnum<class "HasoEngine.lvclass">)  [unwired: 11 in, 1 out]
  n44 = while {
    shift-right: [w296] -> w46
    shift-left: w26 -> [w298]
    shift-right: [w294] -> w45
    shift-left: w38 -> [w295]
    shift-right: [w288] -> w44
    shift-left: w36 -> [w293]
    shift-right: [w287] -> w43
    shift-left: w35 -> [w292]
    shift-right: [w286] -> w42
    shift-left: w34 -> [w291]
    shift-right: [w285] -> w41
    shift-left: w33 -> [w290]
    shift-right: [w284] -> _
    shift-left: w39 -> [w289]
    shift-right: [w283] -> w40
    shift-left: w37 -> [w283]
    tunnel: w26 -> [w282]
    tunnel: w25 -> [w281]
    tunnel: w17 -> [w270]
    shift-right: [w278] -> w10
    shift-left: refnum<class "HasoSlopes.lvclass"> refnum ("HasoSlopes in") -> [w277]
    shift-right: [w276] -> w5
    shift-left: w11 -> [w279]
    shift-right: [w273] -> w6
    shift-left: refnum<class "Phase.lvclass"> refnum ("Phase in") -> [w275]
    shift-right: [w272] -> w4
    shift-left: refnum<class "Pupil.lvclass"> refnum ("Pupil in") -> [w274]
    tunnel: [w270] -> w3
    shift-right: [w269] -> w2
    shift-left: w18 -> [w271]
    stop <- w297 stop-if-true
    n45 = event shown="[0] Timeout" {
      selector: _ -> [_ _ _ _ _ _ _ _ _ _ _ _ _ _]
      dyn-events: _ -> [_ _ _ _ _ _ _ _ _ _ _ _ _ _]
      timeout: 100 -> [_ _ _ _ _ _ _ _ _ _ _ _ _ _]
      tunnel: w298 -> [w314 w452 w455 w468 _ w515 w531 w549 w577 w711 w1282 w1825 _ w2593]
      tunnel: [w300 _ _ _ _ _ _ _ w578 w712 w1283 w1826 "Exit" TRUE ("Exit")] -> w297
      tunnel: [w301 w450 w455 w468 w486 w510 w529 w555 w576 w710 w1281 w1824 w2577 w2598] -> w296
      tunnel: w295 -> [w319 w451 w456 w469 w488 w514 w532 w556 w572 w699 w1270 w1813 w2578 w2600]
      tunnel: [w318 w449 w456 w469 w488 w511 w530 w557 w572 w699 w1270 w1813 w2576 w2599] -> w294
      tunnel: w293 -> [w322 w442 w463 w476 w490 w504 w527 w551 w588 w706 w1277 w1820 w2572 w2594]
      tunnel: w292 -> [w321 w443 w464 w477 w491 w505 w526 w552 w587 w705 w1276 w1819 w2573 w2595]
      tunnel: w291 -> [w320 w444 w465 w478 w492 w506 w525 w553 w586 w704 w1275 w1818 w2574 w2596]
      tunnel: w290 -> [w315 w445 w466 w479 w493 w507 w524 w554 w585 w703 w1274 w1817 w2575 w2597]
      tunnel: w289 -> [w311 w441 w462 w475 w489 w503 _ _ w573 w708 w1279 w1822 _ _]
      tunnel: [w317 w442 w463 w476 w490 w504 w527 w551 w588 w706 w1277 w1820 w2572 w2594] -> w288
      tunnel: [w316 w443 w464 w477 w491 w505 w526 w552 w587 w705 w1276 w1819 w2573 w2595] -> w287
      tunnel: [w313 w444 w465 w478 w492 w506 w525 w553 w586 w704 w1275 w1818 w2574 w2596] -> w286
      tunnel: [w312 w445 w466 w479 w493 w507 w524 w554 w585 w703 w1274 w1817 w2575 w2597] -> w285
      tunnel: [w311 w441 w462 w475 w489 w503 TRUE FALSE w573 w708 w1279 w1822 FALSE FALSE] -> w284
      tunnel: w282 -> [_ _ _ _ w485 _ _ _ _ _ _ _ _ _]
      tunnel: w281 -> [_ _ _ _ _ _ _ _ _ _ _ _ w2570 _]
      tunnel: w277 -> [w310 w439 w460 w473 w483 w497 w522 w547 w569 w701 w1272 w1815 w2568 w2590]
      tunnel: w279 -> [w309 w438 w459 w472 w482 w496 w521 w546 w568 w700 w1271 w1814 w2567 w2589]
      tunnel: [w308 w439 w460 w473 w483 w497 w522 w547 w569 w698 w1269 w1812 w2568 w2590] -> w278
      tunnel: [w307 w438 w459 w472 w482 w496 w521 w546 w568 w700 w1271 w1814 w2567 w2589] -> w276
      tunnel: w275 -> [w306 w440 w461 w474 w484 w498 w523 w548 w570 w702 w1273 w1816 w2569 w2591]
      tunnel: w274 -> [w305 w437 w458 w471 w481 w495 w520 w545 w567 w696 w1267 w1810 w2566 w2588]
      tunnel: [w304 w440 w461 w474 w484 w498 w523 w548 w570 w697 w1268 w1811 w2569 w2591] -> w273
      tunnel: [w303 w437 w458 w471 w481 w495 w520 w545 w567 w695 w1266 w1809 w2566 w2588] -> w272
      tunnel: w271 -> [w302 w436 w457 w470 w480 w494 w519 w544 w575 w709 w1280 w1823 w2565 w2587]
      tunnel: [w302 w436 w457 w470 w480 w494 w519 w544 w571 w707 w1278 w1821 w2565 w2587] -> w269
      event Timeout {
        n46 = event-data() -> ()  [unwired: 1 in, 2 out]
        n47 = case shown="True" w311 {
          tunnel: [w323 w348] -> w301
          tunnel: w322 -> [w332 w351]
          tunnel: [w332 w351] -> w317
          tunnel: [w328 w347] -> w316
          tunnel: w320 -> [w331 w350]
          tunnel: w315 -> [w330 w349]
          tunnel: [w331 w350] -> w313
          tunnel: [w330 w349] -> w312
          tunnel: w321 -> [w328 w347]
          tunnel: w319 -> [w329 w345]
          tunnel: [w329 w346] -> w318
          tunnel: w314 -> [_ w344]
          tunnel: w310 -> [w326 w343]
          tunnel: w309 -> [w325 w342]
          tunnel: [w326 w341] -> w308
          tunnel: [w325 w340] -> w307
          tunnel: w306 -> [w327 w339]
          tunnel: w305 -> [w324 w338]
          tunnel: [w327 w337] -> w304
          tunnel: [w324 w336] -> w303
          frame False {
            n48 = local read "error in (no error)"() -> (w323:errorcluster)
          }
          frame True {
            # "Acqure Wavefront Images"
            n49 = local read "HASO ready"() -> (w333:bool)
            n50 = And(x="Live Wavefront", y=w333) -> (x .and. y?=w335:bool)
            n51 = case shown="True" w335 {
              tunnel: w351 -> [_ w381]
              tunnel: w350 -> [_ w380]
              tunnel: w349 -> [_ w379]
              tunnel: [w352 w376] -> w348
              tunnel: w347 -> [_ w373]
              tunnel: [w357 w372] -> w346
              tunnel: w345 -> [w357 w358]
              tunnel: w344 -> [w352 w359]
              tunnel: w343 -> [w355 w371]
              tunnel: w342 -> [w354 w370]
              tunnel: [w355 w369] -> w341
              tunnel: [w354 w368] -> w340
              tunnel: w339 -> [w356 w367]
              tunnel: w338 -> [w353 w366]
              tunnel: [w356 w365] -> w337
              tunnel: [w353 w364] -> w336
              frame False {
              }
              frame True {
                n52 = property on="nb_images (set)" class="DigNum (strict)"() -> ("Value"=w382:u32)  [unwired: 2 in, 2 out]
                n53 = case shown="1" w382 {
                  tunnel: [w433 w435] -> w383
                  tunnel: w373 -> [w432 _]
                  tunnel: w381 -> [w433 _]
                  tunnel: [w432 w434] -> w378
                  tunnel: w380 -> [_ w435]
                  tunnel: w379 -> [_ w434]
                  frame 2, Default {
                  }
                  frame 1 {
                  }
                }
                n54 = while {
                  tunnel: w358 -> [w388]
                  tunnel: [w387] -> w360
                  tunnel: w359 -> [w385]
                  tunnel: [w384] -> w361
                  stop <- w386 stop-if-true
                  n55 = call <userlib>:"LVClass_Camera asynchroneImageReady.vi"("Camera in"=w388, "error in (no error)"=w385) -> ("Camera out"=w387:refnum<class "Camera.lvclass">, "ready"=w386:bool, "error out"=w384:errorcluster)  [unwired: 11 in]
                }
                n56 = call <userlib>:"LVClass_Camera get image.vi"("Camera in"=w360, "Image"=w383, "Image RAW"=w378, "remove_background"=FALSE, "error in (no error)"=w361) -> ("Camera out"=w372:refnum<class "Camera.lvclass">, "Image (dup)"=w377:refnum<class "Image.lvclass">, "error out"=w374:errorcluster)  [unwired: 7 in, 1 out]
                n57 = case shown="No Error" w374 {
                  selector: w374 -> [w429 w430]
                  tunnel: w377 -> [w426 w431]
                  tunnel: [w424 w431] -> w363
                  tunnel: [w423 w430] -> w362
                  frame No Error {
                    # "get image"
                    n58 = call <userlib>:"LVClass_Image get image data.vi"("Image in"=w426, "error in (no error)"=w429) -> ("Image out"=w428:refnum<class "Image.lvclass">, "Image data out"=w422:u32[][], "error out"=w427:errorcluster)  [unwired: 11 in]
                    n59 = call <userlib>:"LVClass_Image get image information.vi"("Image in"=w428, "error in (no error)"=w427) -> ("Image out"=w424:refnum<class "Image.lvclass">, "Acquisition information"=→"Acquisition information":T5, "error out"=w423:errorcluster)  [unwired: 11 in]
                    n60 = local write "HASO intensity"(w422) -> ()
                  }
                  frame Error {
                  }
                }
                n61 = case shown="No Error" w362 {
                  selector: w362 -> [w409 w421]
                  tunnel: [w415 w421] -> w376
                  tunnel: w363 -> [w408 _]
                  tunnel: [w413 w417] -> w364
                  tunnel: [w412 w420] -> w365
                  tunnel: w371 -> [w405 w419]
                  tunnel: w370 -> [w404 w418]
                  tunnel: [w393 w419] -> w369
                  tunnel: [w403 w418] -> w368
                  tunnel: w367 -> [w401 w420]
                  tunnel: w366 -> [w399 w417]
                  frame No Error {
                    # "phaseout"
                    n62 = call "image2slopes.vi"("error in (no error)"=w409, "Image in"=w408, "HasoEngine in"=w404, "HasoSlopes in"=w405) -> ("error out"=w402:errorcluster, "HasoEngine out"=w403:refnum<class "HasoEngine.lvclass">, "HasoSlopes out"=w395:refnum<class "HasoSlopes.lvclass">)  [unwired: 4 in, 1 out]
                    n63 = local read "Filter"() -> (w398:u8[])
                    n64 = call "slopes2phase.vi"("TypePhase"=WavefrontReconstructionMode."Modal_Zernike", "Number of coefficients"=u8 32, "error in (no error)"=w402, "Filter"=w398, "HasoSlopes in"=w395, "Phase in"=w401) -> ("error out"=w392:errorcluster, "HasoSlopes out"=w394:refnum<class "HasoSlopes.lvclass">, "Phase out"=w400:refnum<class "Phase.lvclass">)  [unwired: 3 in]
                    n65 = local read "idxType"() -> (w389:enum16{"Wyant", "ANSI"})
                    n66 = call "slopes2zern.vi"("HasoSlopes in"=w394, "error in (no error)"=w392, "idxType"=w389) -> ("HasoSlopes out"=w393:refnum<class "HasoSlopes.lvclass">, "Zernike Coefficients"=w390:dbl[], "error out"=w391:errorcluster)  [unwired: 3 in, 2 out]
                    n67 = call <userlib>:"LVClass_Pupil ctor from HasoSlopes.vi"("Pupil in"=w399, "HasoSlopes.lvclass"=w395, "error in (no error)"=w391) -> ("Pupil out"=w410:refnum<class "Pupil.lvclass">, "error out"=w411:errorcluster)  [unwired: 11 in]
                    n68 = call <userlib>:"LVClasse_Phase GetStatisticDatas.vi"("Phase in"=w400, "error in (no error)"=w411) -> ("Phase out"=w416:refnum<class "Phase.lvclass">, "StatisticsData"=w396:T2, "error out"=w414:errorcluster)  [unwired: 11 in]
                    n69 = local write "Phase statistics"(w396) -> ()
                    n70 = call <userlib>:"LVClasse_Phase Get Data.vi"("Phase in"=w416, "Pupil"=w410, "error in (no error)"=w414) -> ("Phase out"=w412:refnum<class "Phase.lvclass">, "data"=w397:sgl[][], "Pupil (dup)"=w413:refnum<class "Pupil.lvclass">, "error out"=w415:errorcluster)  [unwired: 9 in]
                    n71 = local write "Zernike Measured"(w390) -> ()
                    n72 = local write "Phase values"(w397) -> ()
                  }
                  frame Error {
                  }
                }
              }
            }
          }
        }
        "Current error" <- w301
        n73 = Unbundle By Name(w301) -> ("status"=w300:bool)
      }
      event "nb_images (set)": Value Change {
        # "SET IMAGE NUMBER"
        n74 = event-data() -> ("NewVal"=w453:u32)  [unwired: 1 in]
        n75 = call <userlib>:"LVClass_Camera set nbImagesToSum.vi"("Camera in"=w451, "nb_image"=w453, "error in (no error)"=w452) -> ("Camera out"=w448:refnum<class "Camera.lvclass">, "error out"=w447:errorcluster)  [unwired: 11 in]
        n76 = call <userlib>:"LVClass_Camera get nbImagesToSum.vi"("Camera in"=w448, "error in (no error)"=w447) -> ("Camera out"=w449:refnum<class "Camera.lvclass">, "nb_image"=→"nb_images (get)":u32, "error out"=w450:errorcluster)  [unwired: 11 in]
      }
      event "Coef Min": Value Change {
        # "Set coeff display scale: min"
        n77 = event-data() -> ()  [unwired: 1 in, 1 out]
        n78 = local read "Coef Min"() -> (w454:dbl)
        n79 = property on="Zernike Measured" class="WFGraph (strict)"("YScale.Minimum"=w454) -> ()  [unwired: 2 in, 2 out]
      }
      event "Coef Max": Value Change {
        # "Set coeff display scale: min"
        n80 = event-data() -> ()  [unwired: 1 in, 1 out]
        n81 = local read "Coef Max"() -> (w467:dbl)
        n82 = property on="Zernike Measured" class="WFGraph (strict)"("YScale.Maximum"=w467) -> ()  [unwired: 2 in, 2 out]
      }
      event "Reset error": Mouse Up {
        n83 = event-data() -> ()  [unwired: 1 in, 8 out]
        n84 = Select(t=w485, s=w485, f=errorcluster {"status"=FALSE, "code"=0, "source"=""} ("error out")) -> (s? t:f=w486:errorcluster)
      }
      event "exposure_duration_s (set)": Value Change {
        # "CHANGE EXPOSURE DURATION"
        n85 = event-data() -> ()  [unwired: 1 in, 1 out]
        n86 = Multiply(x=1000000.0, y="exposure_duration_s (set)") -> (x*y=w501:dbl)
        n87 = To Unsigned Long Integer(number=w501) -> (unsigned 32bit integer=w500:u32)
        n88 = call <userlib>:"LVClass_Camera set Parameter Int.vi"("Camera in"=w514, "parameter_name"="exposure_duration_us", "value"=w500, "error in (no error)"=w515) -> ("Camera out"=w513:refnum<class "Camera.lvclass">, "error out"=w512:errorcluster)  [unwired: 10 in]
        n89 = call <userlib>:"LVClass_Camera get Parameter Int.vi"("Camera in"=w513, "parameter_name"="exposure_duration_us", "error in (no error)"=w512) -> ("Camera out"=w511:refnum<class "Camera.lvclass">, "value"=→"exposure_duration_us (get)":i32, "error out"=w510:errorcluster)  [unwired: 10 in]
      }
      event "Start HASO": Mouse Up {
        # "Start acquisition in SYNCRHONOUS mode\n\nonly one acquisition mode is available :\nLast image"
        n90 = event-data() -> ()  [unwired: 1 in, 8 out]
        n91 = flat-sequence {
          tunnel: w532 -> [w538]
          tunnel: w531 -> [w537]
          tunnel: [w536] -> w518
          tunnel: [w535] -> w517
          tunnel: [w540] -> w529
          tunnel: [w541] -> w530
          tunnel: w518 -> [w541]
          tunnel: w517 -> [w540]
          frame #0 {
            n92 = call <userlib>:"LVClass_Camera start acquisition.vi"("Camera in"=w538, "synchronisation_mode"=enum16{"synchronous", "asynchronous"}."asynchronous", "acquisition_mode"=enum16{"last_image", "new_image"}."last_image", "error in (no error)"=w537) -> ("Camera out"=w536:refnum<class "Camera.lvclass">, "error out"=w535:errorcluster)  [unwired: 10 in]
          }
          frame #1 {
            n93 = local write "HASO ready"(TRUE) -> ()
          }
        }
      }
      event "Stop HASO": Mouse Up {
        n94 = event-data() -> ()  [unwired: 1 in, 8 out]
        n95 = flat-sequence {
          tunnel: w556 -> [w560]
          tunnel: w549 -> [w558]
          tunnel: [w561] -> w543
          tunnel: [w559] -> w542
          tunnel: [w563] -> w555
          tunnel: [w564] -> w557
          tunnel: w543 -> [w564]
          tunnel: w542 -> [w563]
          frame #0 {
            n96 = call <userlib>:"LVClass_Camera stop acquisition.vi"("Camera in"=w560, "error in (no error)"=w558) -> ("Camera out"=w561:refnum<class "Camera.lvclass">, "error out"=w559:errorcluster)  [unwired: 12 in]
          }
          frame #1 {
            n97 = local write "HASO ready"(FALSE) -> ()
          }
        }
      }
      event "Update DM": Mouse Up {
        n98 = event-data() -> ()  [unwired: 1 in, 8 out]
        n99 = local read "Initial offset"() -> (w574:bool)
        n100 = case shown="True" w574 {
          tunnel: [w589 w594] -> w579
          frame False {
            n101 = Initialize Array(0.0, 52) -> (w589:dbl[])
          }
          frame True {
            n102 = local read "Offset command file"() -> (w593:path)
            n103 = call-poly <vilib>:"Read From Spreadsheet File.vi"("format (%.3f)"="%.8f", "file path (dialog if empty)"=w593) -> ("first row"=w594:dbl[])  [unwired: 5 in, 4 out]
          }
        }
        n104 = local read "Additional Command"() -> (w584:bool)
        n105 = case shown="True" w584 {
          tunnel: [w596 w602] -> w580
          tunnel: [w595 w601] -> w581
          tunnel: w577 -> [w595 w600]
          frame False {
            n106 = Initialize Array(0.0, 52) -> (w596:dbl[])
          }
          frame True {
            n107 = local read "Input type"() -> (w599:T4)
            n108 = case shown="\"DM actuators\"" w599 {
              tunnel: w600 -> [w603 w608 w651 w665 w674]
              tunnel: [w604 w610 w652 w663 w676] -> w602
              tunnel: [w603 w607 w651 w662 w673] -> w601
              frame "Zero Input" {
                n109 = Initialize Array(0.0, 52) -> (w604:dbl[])
              }
              frame "DM actuators" {
                w614 = 1
                w615 = 52
                n110 = local read "Zern/DM index in"() -> (w611:i32[])
                n111 = local read "Zern/DM coef in"() -> (w609:sgl[])
                n112 = Array Size(array=w611) -> (size(s)=w619:i32)
                n113 = Initialize Array(0.0, w615) -> (w617:dbl[])
                n114 = call-poly <vilib>:"Ramp Pattern.vi"("start"=w614, "end"=w615, "delta"=w614) -> ("Ramp Pattern"=w616:dbl[])  [unwired: 6 in, 2 out]
                n115 = Less Or Equal?(x=w619, y=w615) -> (x <= y?=w618:bool)
                n116 = case shown="True" w618 {
                  tunnel: w619 -> [_ w630]
                  tunnel: w617 -> [w623 w629]
                  tunnel: [w623 w628] -> w610
                  tunnel: w611 -> [_ w627]
                  tunnel: w609 -> [_ w626]
                  tunnel: [w620 w624] -> w607
                  tunnel: w615 -> [_ w625]
                  tunnel: w608 -> [w622 w624]
                  frame False {
                    n117 = Merge Errors(w622, errorcluster {"status"=FALSE, "code"=0, "source"="Wrong Zern index size"} ("error out")) -> (w620:errorcluster)
                  }
                  frame True {
                    n118 = for {
                      N: w630 -> [_]
                      shift-right: [w643] -> w628
                      shift-left: w629 -> [w644]
                      tunnel: w627 -> [w640] mode=indexing
                      tunnel: w626 -> [w634] mode=indexing
                      tunnel: w625 -> [w641]
                      n119 = Greater Than 0?(x=w640) -> (x > 0?=w639:bool)
                      n120 = Less Or Equal?(x=w640, y=w641) -> (x <= y?=w631:bool)
                      n121 = And(x=w639, y=w631) -> (x .and. y?=w638:bool)
                      n122 = In Range and Coerce(upper limit=0.8, x=w634, lower limit=-0.8) -> (coerced(x)=w635:dbl, In Range?=w637:bool)
                      n123 = And(x=w638, y=w637) -> (x .and. y?=w636:bool)
                      n124 = Decrement(x=w640) -> (x-1=w642:i32)
                      n125 = case shown="True" w636 {
                        tunnel: w642 -> [_ w649]
                        tunnel: w644 -> [w645 w648]
                        tunnel: [w645 w647] -> w643
                        tunnel: w635 -> [_ w646]
                        frame False {
                        }
                        frame True {
                          n126 = Replace Array Subset(array=w648, new element=w646, index=w649) -> (w647:dbl[])
                        }
                      }
                    }
                  }
                }
                n127 = local write "Coef out"(w610) -> ()
                n128 = To Long Integer(number=w616) -> (32bit integer=w612:i32[])
                n129 = local write "Index out"(w612) -> ()
              }
              frame "Command File" {
                n130 = local read "Additional file"() -> (w650:path)
                n131 = call-poly <vilib>:"Read From Spreadsheet File.vi"("format (%.3f)"="%.8f", "file path (dialog if empty)"=w650) -> ("first row"=w652:dbl[])  [unwired: 5 in, 4 out]
              }
              frame "Zernike Coef", Default {
                n132 = local read "Zern/DM index in"() -> (w654:i32[])
                n133 = local read "Zern/DM coef in"() -> (w655:sgl[])
                n134 = local read "idxType"() -> (w661:enum16{"Wyant", "ANSI"})
                n135 = local read "Initial haso file"() -> (w659:path)
                n136 = local read "Haso configuration file"() -> (w660:path)
                n137 = local read "interaction matrix file"() -> (w658:path)
                n138 = call "zern2command.vi"("Haso configuration file"=w660, "idxType"=w661, "interaction matrix file"=w658, "error in (no error)"=w665, "Zern coef in"=w655, "Zern index in"=w654, "Initial haso file"=w659) -> ("error out"=w664:errorcluster, "Offset Positions"=w663:sgl[], "Zern pupil out"=w666:refnum<class "Pupil.lvclass">, "ModalCoef out"=w667:refnum<class "ModalCoef.lvclass">)  [unwired: 1 in]
                n139 = call <userlib>:"LVClass_ModalCoef GetData.vi"("ModalCoef in"=w667, "Pupil.lvclass"=w666, "error in (no error)"=w664) -> ("ModalCoef out"=w671:refnum<class "ModalCoef.lvclass">, "coef"=w657:sgl[], "index"=w656:u32[], "Pupil.lvclass (dup)"=w670:refnum<class "Pupil.lvclass">, "error out"=w669:errorcluster)  [unwired: 8 in]
                n140 = local write "Index out"(w656) -> ()
                n141 = call <userlib>:"LVClass_Pupil dtor.vi"("Pupil in"=w670, "error in (no error)"=w669) -> ("error out"=w668:errorcluster)  [unwired: 12 in, 1 out]
                n142 = local write "Coef out"(w657) -> ()
                n143 = call <userlib>:"LVClass_ModalCoef dtor.vi"("ModalCoef in"=w671, "error in (no error)"=w668) -> ("error out"=w662:errorcluster)  [unwired: 12 in, 1 out]
              }
              frame "Zernike File" {
                w679 = 1
                n144 = local read "interaction matrix file"() -> (w683:path)
                n145 = local read "Initial haso file"() -> (w681:path)
                n146 = local read "Haso configuration file"() -> (w682:path)
                n147 = local read "Additional file"() -> (w692:path)
                n148 = call-poly <vilib>:"Ramp Pattern.vi"("start"=w679, "end"=32, "delta"=w679) -> ("Ramp Pattern"=w680:dbl[])  [unwired: 6 in, 2 out]
                n149 = To Long Integer(number=w680) -> (32bit integer=w677:i32[])
                n150 = local read "idxType"() -> (w672:enum16{"Wyant", "ANSI"})
                n151 = call-poly <vilib>:"Read From Spreadsheet File.vi"("format (%.3f)"="%.8f", "file path (dialog if empty)"=w692) -> ("first row"=w684:dbl[])  [unwired: 5 in, 4 out]
                n152 = call "zern2command.vi"("Haso configuration file"=w682, "idxType"=w672, "interaction matrix file"=w683, "Zern coef in"=w684, "Zern index in"=w677, "Initial haso file"=w681) -> ("error out"=w685:errorcluster, "Offset Positions"=w676:sgl[], "Zern pupil out"=w686:refnum<class "Pupil.lvclass">, "ModalCoef out"=w687:refnum<class "ModalCoef.lvclass">)  [unwired: 2 in]
                n153 = call <userlib>:"LVClass_ModalCoef GetData.vi"("ModalCoef in"=w687, "Pupil.lvclass"=w686, "error in (no error)"=w685) -> ("ModalCoef out"=w691:refnum<class "ModalCoef.lvclass">, "Pupil.lvclass (dup)"=w690:refnum<class "Pupil.lvclass">, "error out"=w689:errorcluster)  [unwired: 8 in, 2 out]
                n154 = call <userlib>:"LVClass_Pupil dtor.vi"("Pupil in"=w690, "error in (no error)"=w689) -> ("error out"=w688:errorcluster)  [unwired: 12 in, 1 out]
                n155 = call <userlib>:"LVClass_ModalCoef dtor.vi"("ModalCoef in"=w691, "error in (no error)"=w688) -> ("error out"=w675:errorcluster)  [unwired: 12 in, 1 out]
                n156 = Merge Errors(w675, w674) -> (w673:errorcluster)
              }
            }
          }
        }
        n157 = local write "Initial Positions"(w579) -> ()
        n158 = Add(x=w580, y=w579) -> (x+y=w565:dbl[])
        n159 = call <userlib>:"LVClass_WavefrontCorrector Move to Absolute Position.vi"("WavefrontCorrector in"=w575, "Absolute Positions"=w565, "error in (no error)"=w581) -> ("WavefrontCorrector out"=w582:refnum<class "WavefrontCorrector.lvclass">, "error out"=w583:errorcluster)  [unwired: 11 in]
        n160 = call <userlib>:"LVClass_WavefrontCorrector Get Current Position.vi"("WavefrontCorrector in"=w582, "error in (no error)"=w583) -> ("WavefrontCorrector out"=w571:refnum<class "WavefrontCorrector.lvclass">, "Wavefront Corrector Position"=w566:T14, "error out"=w576:errorcluster)  [unwired: 11 in]
        n161 = local write "Final Positions"(w565) -> ()
        n162 = local write "DM Actuator Values"(w566) -> ()
        n163 = Unbundle By Name(w576) -> ("status"=w578:bool)
      }
      event "Record Response": Mouse Up {
        n164 = event-data() -> ()  [unwired: 1 in, 8 out]
        n165 = local read "Net Rp"() -> (w694:bool)
        n166 = stacked-sequence {
          seq-local: [_ _ _ w1080 _] -> [_ _ _ _ w1105]
          seq-local: [_ _ w947 _ _] -> [_ _ _ w1079 _]
          seq-local: [_ w742 _ _ _] -> [_ _ w948 _ _]
          seq-local: [_ _ w946 _ _] -> [_ _ _ _ w1101]
          tunnel: [_ _ _ _ w1104] -> w712
          tunnel: w711 -> [_ w755 _ _ _]
          tunnel: [_ _ _ _ w1103] -> w710
          tunnel: w709 -> [_ w754 _ w1081 _]
          tunnel: [_ w752 _ _ _] -> w707
          tunnel: w706 -> [_ _ w960 _ w1113]
          tunnel: w705 -> [_ _ w959 _ w1112]
          tunnel: w704 -> [_ _ w958 _ w1111]
          tunnel: w703 -> [_ _ w957 _ w1110]
          tunnel: w702 -> [_ _ w956 _ w1109]
          tunnel: w701 -> [_ _ w955 _ _]
          tunnel: w700 -> [_ _ w954 _ w1108]
          tunnel: w696 -> [_ _ w953 _ w1107]
          tunnel: w699 -> [_ _ w952 _ w1106]
          tunnel: [_ _ _ _ w1100] -> w698
          tunnel: [_ _ w950 _ _] -> w697
          tunnel: [_ _ w949 _ _] -> w695
          tunnel: w694 -> [_ _ _ w1078 w1102]
          frame #0 {
            # "Create output folder path"
            n167 = Get Date/Time In Seconds() -> (seconds since 1Jan1904=w726:timestamp)
            n168 = local read "Folder Name"() -> (w718:string)
            n169 = Format Date/Time String(time format string (%c)="%Y%m%d", seconds (now)=w726) -> (date/time string=w725:string)  [unwired: 1 in]
            n170 = local read "Main Path"() -> (w719:path)
            n171 = local read "Subfolder"() -> (w717:string)
            n172 = Concatenate Strings(w725, "_", w718) -> (w724:string)
            n173 = Build Path(base path=w719, name or relative path=w724) -> (appended path=w722:path)
            n174 = call <vilib>:"Check if File or Folder Exists.vi"("path"=w722) -> ("error out"=w714:errorcluster, "file or folder exists?"=w728:bool)  [unwired: 8 in, 1 out]
            n175 = local write "Current status"("Check single response") -> ()
            n176 = Build Path(base path=w722, name or relative path=w717) -> (appended path=w716:path)
            n177 = case shown="False" w728 {
              tunnel: w722 -> [w740 _]
              tunnel: w714 -> [w739 w741]
              tunnel: [w738 w741] -> w713
              frame False {
                n178 = Create Folder(path (use dialog)=w740, error in=w739) -> (error out=w738:errorcluster)  [unwired: 1 in, 2 out]
              }
              frame True {
              }
            }
            n179 = call <vilib>:"Check if File or Folder Exists.vi"("error in (no error)"=w713, "path"=w716) -> ("error out"=w723:errorcluster, "file or folder exists?"=w727:bool)  [unwired: 7 in, 1 out]
            n180 = case shown="True" w727 {
              tunnel: w716 -> [w731 w736]
              tunnel: w723 -> [w730 w737]
              tunnel: [w729 w732] -> _
              frame False {
                n181 = Create Folder(path (use dialog)=w731, error in=w730) -> (error out=w729:errorcluster)  [unwired: 1 in, 2 out]
              }
              frame True {
                n182 = Delete(path (use dialog)=w736, entire hierarchy (F)=TRUE, error in=w737) -> (deleted path=w734:path, error out=w733:errorcluster)  [unwired: 2 in, 1 out]
                n183 = Create Folder(path (use dialog)=w734, error in=w733) -> (error out=w732:errorcluster)  [unwired: 1 in, 2 out]
              }
            }
            n184 = local write "Output path"(w716) -> ()
          }
          frame #1 {
            # "Delay for DM response"
            # "Apply command to DM"
            n185 = local read "Initial offset"() -> (w753:bool)
            n186 = case shown="True" w753 {
              tunnel: [w841 w846] -> w744
              frame False {
                n187 = Initialize Array(0.0, 52) -> (w841:dbl[])
              }
              frame True {
                n188 = local read "Offset command file"() -> (w845:path)
                n189 = call-poly <vilib>:"Read From Spreadsheet File.vi"("format (%.3f)"="%.8f", "file path (dialog if empty)"=w845) -> ("first row"=w846:dbl[])  [unwired: 5 in, 4 out]
              }
            }
            n190 = local read "Additional Command"() -> (w759:bool)
            n191 = case shown="True" w759 {
              tunnel: [w848 w854] -> w745
              tunnel: [w847 w853] -> w756
              tunnel: w755 -> [w847 w852]
              frame False {
                n192 = Initialize Array(0.0, 52) -> (w848:dbl[])
              }
              frame True {
                n193 = local read "Input type"() -> (w851:T4)
                n194 = case shown="\"DM actuators\"" w851 {
                  tunnel: w852 -> [w855 w861 w903 w917 w926]
                  tunnel: [w856 w859 w904 w915 w928] -> w854
                  tunnel: [w855 w860 w903 w914 w925] -> w853
                  frame "Zero Input" {
                    n195 = Initialize Array(0.0, 52) -> (w856:dbl[])
                  }
                  frame "DM actuators" {
                    w863 = 1
                    w864 = 52
                    n196 = local read "Zern/DM index in"() -> (w870:i32[])
                    n197 = local read "Zern/DM coef in"() -> (w871:sgl[])
                    n198 = Array Size(array=w870) -> (size(s)=w865:i32)
                    n199 = Initialize Array(0.0, w864) -> (w867:dbl[])
                    n200 = call-poly <vilib>:"Ramp Pattern.vi"("start"=w863, "end"=w864, "delta"=w863) -> ("Ramp Pattern"=w868:dbl[])  [unwired: 6 in, 2 out]
                    n201 = Less Or Equal?(x=w865, y=w864) -> (x <= y?=w866:bool)
                    n202 = case shown="True" w866 {
                      tunnel: w865 -> [_ w882]
                      tunnel: w867 -> [w875 w881]
                      tunnel: [w875 w880] -> w859
                      tunnel: w870 -> [_ w879]
                      tunnel: w871 -> [_ w878]
                      tunnel: [w872 w876] -> w860
                      tunnel: w864 -> [_ w877]
                      tunnel: w861 -> [w874 w876]
                      frame False {
                        n203 = Merge Errors(w874, errorcluster {"status"=FALSE, "code"=0, "source"="Wrong Zern index size"} ("error out")) -> (w872:errorcluster)
                      }
                      frame True {
                        n204 = for {
                          N: w882 -> [_]
                          shift-right: [w895] -> w880
                          shift-left: w881 -> [w896]
                          tunnel: w879 -> [w892] mode=indexing
                          tunnel: w878 -> [w886] mode=indexing
                          tunnel: w877 -> [w893]
                          n205 = Greater Than 0?(x=w892) -> (x > 0?=w891:bool)
                          n206 = Less Or Equal?(x=w892, y=w893) -> (x <= y?=w883:bool)
                          n207 = And(x=w891, y=w883) -> (x .and. y?=w890:bool)
                          n208 = In Range and Coerce(upper limit=0.8, x=w886, lower limit=-0.8) -> (coerced(x)=w887:dbl, In Range?=w889:bool)
                          n209 = And(x=w890, y=w889) -> (x .and. y?=w888:bool)
                          n210 = Decrement(x=w892) -> (x-1=w894:i32)
                          n211 = case shown="True" w888 {
                            tunnel: w894 -> [_ w901]
                            tunnel: w896 -> [w897 w900]
                            tunnel: [w897 w899] -> w895
                            tunnel: w887 -> [_ w898]
                            frame False {
                            }
                            frame True {
                              n212 = Replace Array Subset(array=w900, new element=w898, index=w901) -> (w899:dbl[])
                            }
                          }
                        }
                      }
                    }
                    n213 = local write "Coef out"(w859) -> ()
                    n214 = To Long Integer(number=w868) -> (32bit integer=w869:i32[])
                    n215 = local write "Index out"(w869) -> ()
                  }
                  frame "Command File" {
                    n216 = local read "Additional file"() -> (w902:path)
                    n217 = call-poly <vilib>:"Read From Spreadsheet File.vi"("format (%.3f)"="%.8f", "file path (dialog if empty)"=w902) -> ("first row"=w904:dbl[])  [unwired: 5 in, 4 out]
                  }
                  frame "Zernike Coef", Default {
                    n218 = local read "Zern/DM index in"() -> (w906:i32[])
                    n219 = local read "Zern/DM coef in"() -> (w907:sgl[])
                    n220 = local read "idxType"() -> (w913:enum16{"Wyant", "ANSI"})
                    n221 = local read "Initial haso file"() -> (w911:path)
                    n222 = local read "Haso configuration file"() -> (w912:path)
                    n223 = local read "interaction matrix file"() -> (w910:path)
                    n224 = call "zern2command.vi"("Haso configuration file"=w912, "idxType"=w913, "interaction matrix file"=w910, "error in (no error)"=w917, "Zern coef in"=w907, "Zern index in"=w906, "Initial haso file"=w911) -> ("error out"=w916:errorcluster, "Offset Positions"=w915:sgl[], "Zern pupil out"=w918:refnum<class "Pupil.lvclass">, "ModalCoef out"=w919:refnum<class "ModalCoef.lvclass">)  [unwired: 1 in]
                    n225 = call <userlib>:"LVClass_ModalCoef GetData.vi"("ModalCoef in"=w919, "Pupil.lvclass"=w918, "error in (no error)"=w916) -> ("ModalCoef out"=w923:refnum<class "ModalCoef.lvclass">, "coef"=w909:sgl[], "index"=w908:u32[], "Pupil.lvclass (dup)"=w922:refnum<class "Pupil.lvclass">, "error out"=w921:errorcluster)  [unwired: 8 in]
                    n226 = local write "Index out"(w908) -> ()
                    n227 = call <userlib>:"LVClass_Pupil dtor.vi"("Pupil in"=w922, "error in (no error)"=w921) -> ("error out"=w920:errorcluster)  [unwired: 12 in, 1 out]
                    n228 = local write "Coef out"(w909) -> ()
                    n229 = call <userlib>:"LVClass_ModalCoef dtor.vi"("ModalCoef in"=w923, "error in (no error)"=w920) -> ("error out"=w914:errorcluster)  [unwired: 12 in, 1 out]
                  }
                  frame "Zernike File" {
                    w931 = 1
                    n230 = local read "interaction matrix file"() -> (w935:path)
                    n231 = local read "Initial haso file"() -> (w933:path)
                    n232 = local read "Haso configuration file"() -> (w934:path)
                    n233 = local read "Additional file"() -> (w944:path)
                    n234 = call-poly <vilib>:"Ramp Pattern.vi"("start"=w931, "end"=32, "delta"=w931) -> ("Ramp Pattern"=w932:dbl[])  [unwired: 6 in, 2 out]
                    n235 = To Long Integer(number=w932) -> (32bit integer=w929:i32[])
                    n236 = local read "idxType"() -> (w924:enum16{"Wyant", "ANSI"})
                    n237 = call-poly <vilib>:"Read From Spreadsheet File.vi"("format (%.3f)"="%.8f", "file path (dialog if empty)"=w944) -> ("first row"=w936:dbl[])  [unwired: 5 in, 4 out]
                    n238 = call "zern2command.vi"("Haso configuration file"=w934, "idxType"=w924, "interaction matrix file"=w935, "Zern coef in"=w936, "Zern index in"=w929, "Initial haso file"=w933) -> ("error out"=w937:errorcluster, "Offset Positions"=w928:sgl[], "Zern pupil out"=w938:refnum<class "Pupil.lvclass">, "ModalCoef out"=w939:refnum<class "ModalCoef.lvclass">)  [unwired: 2 in]
                    n239 = call <userlib>:"LVClass_ModalCoef GetData.vi"("ModalCoef in"=w939, "Pupil.lvclass"=w938, "error in (no error)"=w937) -> ("ModalCoef out"=w943:refnum<class "ModalCoef.lvclass">, "Pupil.lvclass (dup)"=w942:refnum<class "Pupil.lvclass">, "error out"=w941:errorcluster)  [unwired: 8 in, 2 out]
                    n240 = call <userlib>:"LVClass_Pupil dtor.vi"("Pupil in"=w942, "error in (no error)"=w941) -> ("error out"=w940:errorcluster)  [unwired: 12 in, 1 out]
                    n241 = call <userlib>:"LVClass_ModalCoef dtor.vi"("ModalCoef in"=w943, "error in (no error)"=w940) -> ("error out"=w927:errorcluster)  [unwired: 12 in, 1 out]
                    n242 = Merge Errors(w927, w926) -> (w925:errorcluster)
                  }
                }
              }
            }
            n243 = local read "File Base Name"() -> (w746:string)
            n244 = local read "Output path"() -> (w750:path)
            n245 = local read "Input type"() -> (w747:T4)
            n246 = local read "Save File"() -> (w751:bool)
            n247 = local write "Initial Positions"(w744) -> ()
            n248 = Add(x=w745, y=w744) -> (x+y=w748:dbl[])
            n249 = call <userlib>:"LVClass_WavefrontCorrector Move to Absolute Position.vi"("WavefrontCorrector in"=w754, "Absolute Positions"=w748, "error in (no error)"=w756) -> ("WavefrontCorrector out"=w757:refnum<class "WavefrontCorrector.lvclass">, "error out"=w758:errorcluster)  [unwired: 11 in]
            n250 = call <userlib>:"LVClass_WavefrontCorrector Get Current Position.vi"("WavefrontCorrector in"=w757, "error in (no error)"=w758) -> ("WavefrontCorrector out"=w752:refnum<class "WavefrontCorrector.lvclass">, "Wavefront Corrector Position"=w749:T14, "error out"=w743:errorcluster)  [unwired: 11 in]
            n251 = case shown="True" w751 {
              tunnel: w750 -> [_ w768]
              tunnel: w746 -> [_ w767]
              tunnel: w744 -> [_ w766]
              tunnel: w745 -> [_ w765]
              tunnel: w748 -> [_ w764]
              tunnel: w747 -> [_ w763]
              tunnel: w749 -> [_ w762]
              frame False {
              }
              frame True {
                n252 = stacked-sequence {
                  tunnel: w768 -> [w773 w782 w791 w800 w807 w819 w831]
                  tunnel: w767 -> [w771 w780 w789 w798 w806 w818 w830]
                  tunnel: w766 -> [w769 _ _ _ _ _ _]
                  tunnel: w765 -> [_ w778 _ _ _ _ _]
                  tunnel: w764 -> [_ _ w787 _ _ _ _]
                  tunnel: w763 -> [_ _ _ _ w805 w817 w829]
                  tunnel: w762 -> [_ _ _ w796 _ _ _]
                  frame #0 {
                    n253 = Concatenate Strings(w771, "_cmdOffset", ".dat") -> (w774:string)
                    n254 = Build Path(base path=w773, name or relative path=w774) -> (appended path=w775:path)
                    n255 = Array To Spreadsheet String(array=w769, 3:"%f") -> (spreadsheet string=w776:string)  [unwired: 1 in]
                    n256 = Write to Text File(file (use dialog)=w775, text=w776) -> ()  [unwired: 2 in, 3 out]
                  }
                  frame #1 {
                    n257 = Concatenate Strings(w780, "_cmdAdd", ".dat") -> (w783:string)
                    n258 = Build Path(base path=w782, name or relative path=w783) -> (appended path=w784:path)
                    n259 = Array To Spreadsheet String(array=w778, 3:"%f") -> (spreadsheet string=w785:string)  [unwired: 1 in]
                    n260 = Write to Text File(file (use dialog)=w784, text=w785) -> ()  [unwired: 2 in, 3 out]
                  }
                  frame #2 {
                    n261 = Concatenate Strings(w789, "_cmdFinal", ".dat") -> (w792:string)
                    n262 = Build Path(base path=w791, name or relative path=w792) -> (appended path=w793:path)
                    n263 = Array To Spreadsheet String(array=w787, 3:"%f") -> (spreadsheet string=w794:string)  [unwired: 1 in]
                    n264 = Write to Text File(file (use dialog)=w793, text=w794) -> ()  [unwired: 2 in, 3 out]
                  }
                  frame #3 {
                    n265 = Concatenate Strings(w798, "_cmdFinalMirror", ".dat") -> (w801:string)
                    n266 = Build Path(base path=w800, name or relative path=w801) -> (appended path=w802:path)
                    n267 = Array To Spreadsheet String(array=w796, 3:"%f") -> (spreadsheet string=w803:string)  [unwired: 1 in]
                    n268 = Write to Text File(file (use dialog)=w802, text=w803) -> ()  [unwired: 2 in, 3 out]
                  }
                  frame #4 {
                    n269 = case shown="\"Zero Input\"" w805 {
                      tunnel: w807 -> [_ w812]
                      tunnel: w806 -> [_ w810]
                      frame "Zero Input" {
                      }
                      frame "Zernike Coef", Default {
                        n270 = local read "Zern/DM coef in"() -> (w808:sgl[])
                        n271 = Concatenate Strings(w810, "_zernCoef", ".txt") -> (w813:string)
                        n272 = Build Path(base path=w812, name or relative path=w813) -> (appended path=w814:path)
                        n273 = Array To Spreadsheet String(array=w808, 3:"%f") -> (spreadsheet string=w815:string)  [unwired: 1 in]
                        n274 = Write to Text File(file (use dialog)=w814, text=w815) -> ()  [unwired: 2 in, 3 out]
                      }
                    }
                  }
                  frame #5 {
                    n275 = case shown="\"Zernike Coef\", Default" w817 {
                      tunnel: w819 -> [_ w824]
                      tunnel: w818 -> [_ w822]
                      frame "Zero Input" {
                      }
                      frame "Zernike Coef", Default {
                        n276 = local read "Zern/DM index in"() -> (w820:i32[])
                        n277 = Concatenate Strings(w822, "_zernIdx", ".txt") -> (w825:string)
                        n278 = Build Path(base path=w824, name or relative path=w825) -> (appended path=w826:path)
                        n279 = Array To Spreadsheet String(array=w820, 3:"%d") -> (spreadsheet string=w827:string)  [unwired: 1 in]
                        n280 = Write to Text File(file (use dialog)=w826, text=w827) -> ()  [unwired: 2 in, 3 out]
                      }
                    }
                  }
                  frame #6 {
                    n281 = case shown="\"Zernike Coef\", Default" w829 {
                      tunnel: w831 -> [_ w836]
                      tunnel: w830 -> [_ w834]
                      frame "Zero Input" {
                      }
                      frame "Zernike Coef", Default {
                        n282 = Concatenate Strings(w834, "_zernCoefWyant", ".txt") -> (w837:string)
                        n283 = local read "Coef out"() -> (w832:sgl[])
                        n284 = Build Path(base path=w836, name or relative path=w837) -> (appended path=w838:path)
                        n285 = Array To Spreadsheet String(array=w832, 3:"%f") -> (spreadsheet string=w839:string)  [unwired: 1 in]
                        n286 = Write to Text File(file (use dialog)=w838, text=w839) -> ()  [unwired: 2 in, 3 out]
                      }
                    }
                  }
                }
              }
            }
            n287 = local write "Final Positions"(w748) -> ()
            n288 = local write "DM Actuator Values"(w749) -> ()
            n289 = flat-sequence {
              tunnel: [w760] -> w742
              tunnel: w743 -> [w760]
              frame #0 {
                n290 = Wait (ms)(milliseconds to wait=u32 50) -> ()  [unwired: 1 out]
              }
            }
          }
          frame #2 {
            n291 = local read "HASO ready"() -> (w951:bool)
            n292 = case shown="True" w951 {
              tunnel: w960 -> [_ w986]
              tunnel: w958 -> [_ w985]
              tunnel: w957 -> [_ w984]
              tunnel: [w961 w983] -> w947
              tunnel: w959 -> [_ w982]
              tunnel: w952 -> [_ w968]
              tunnel: w948 -> [w961 w969]
              tunnel: w955 -> [w964 w981]
              tunnel: w954 -> [w963 w980]
              tunnel: [w964 w979] -> w946
              tunnel: [w963 w978] -> _
              tunnel: w956 -> [w965 w977]
              tunnel: w953 -> [w962 w976]
              tunnel: [w965 w975] -> w950
              tunnel: [w962 w974] -> w949
              frame False {
              }
              frame True {
                n293 = property on="nb_images (set)" class="DigNum (strict)"() -> ("Value"=w987:u32)  [unwired: 2 in, 2 out]
                n294 = case shown="2, Default" w987 {
                  tunnel: [w1075 w1077] -> w970
                  tunnel: w982 -> [w1074 _]
                  tunnel: w986 -> [w1075 _]
                  tunnel: [w1074 w1076] -> w971
                  tunnel: w985 -> [_ w1077]
                  tunnel: w984 -> [_ w1076]
                  frame 2, Default {
                  }
                  frame 1 {
                  }
                }
                n295 = stacked-sequence {
                  tunnel: w970 -> [_ w1005]
                  tunnel: w971 -> [_ w1004]
                  tunnel: [_ w1003] -> w967
                  tunnel: [_ w1001] -> w966
                  tunnel: [_ w1000] -> _
                  tunnel: w968 -> [_ w997]
                  tunnel: w969 -> [_ w996]
                  frame #0 {
                    # "Delay until MD gets stable"
                    n296 = local read "exposure_duration_s (set)"() -> (w988:dbl)
                    n297 = local read "nb_images (set)"() -> (w989:u32)
                    n298 = Multiply(x=w988, y=w989) -> (x*y=w990:dbl)
                    n299 = Add(x=w990, y=1.0) -> (x+y=w991:dbl)
                    n300 = Multiply(x=w991, y=1000.0) -> (x*y=w995:dbl)
                    n301 = To Unsigned Long Integer(number=w995) -> (unsigned 32bit integer=w994:u32)
                    n302 = Wait (ms)(milliseconds to wait=w994) -> ()  [unwired: 1 out]
                  }
                  frame #1 {
                    n303 = while {
                      tunnel: w997 -> [w1010]
                      tunnel: [w1009] -> w999
                      tunnel: w996 -> [w1007]
                      tunnel: [w1006] -> w998
                      stop <- w1008 stop-if-true
                      n304 = call <userlib>:"LVClass_Camera asynchroneImageReady.vi"("Camera in"=w1010, "error in (no error)"=w1007) -> ("Camera out"=w1009:refnum<class "Camera.lvclass">, "ready"=w1008:bool, "error out"=w1006:errorcluster)  [unwired: 11 in]
                    }
                    n305 = call <userlib>:"LVClass_Camera get image.vi"("Camera in"=w999, "Image"=w1005, "Image RAW"=w1004, "remove_background"=FALSE, "error in (no error)"=w998) -> ("Camera out"=w1000:refnum<class "Camera.lvclass">, "Image (dup)"=w1003:refnum<class "Image.lvclass">, "error out"=w1001:errorcluster)  [unwired: 7 in, 1 out]
                  }
                }
                n306 = case shown="No Error" w966 {
                  selector: w966 -> [w1071 w1072]
                  tunnel: w967 -> [w1070 w1073]
                  tunnel: [w1067 w1073] -> w973
                  tunnel: [w1068 w1072] -> w972
                  frame No Error {
                    # "get image"
                    n307 = call <userlib>:"LVClass_Image get image data.vi"("Image in"=w1070, "error in (no error)"=w1071) -> ("Image out"=w1067:refnum<class "Image.lvclass">, "Image data out"=w1069:u32[][], "error out"=w1068:errorcluster)  [unwired: 11 in]
                    n308 = local write "HASO intensity"(w1069) -> ()
                  }
                  frame Error {
                  }
                }
                n309 = case shown="No Error" w972 {
                  selector: w972 -> [w1034 w1066]
                  tunnel: [w1040 w1066] -> w983
                  tunnel: w973 -> [w1033 _]
                  tunnel: [w1038 w1062] -> w974
                  tunnel: [w1037 w1065] -> w975
                  tunnel: w981 -> [w1030 w1064]
                  tunnel: w980 -> [w1029 w1063]
                  tunnel: [w1017 w1064] -> w979
                  tunnel: [w1028 w1063] -> w978
                  tunnel: w977 -> [w1026 w1065]
                  tunnel: w976 -> [w1024 w1062]
                  frame No Error {
                    # "phaseout"
                    n310 = local read "File Base Name"() -> (w1015:string)
                    n311 = local read "Save File"() -> (w1016:bool)
                    n312 = local read "Output path"() -> (w1014:path)
                    n313 = call "image2slopes.vi"("error in (no error)"=w1034, "Image in"=w1033, "HasoEngine in"=w1029, "HasoSlopes in"=w1030) -> ("error out"=w1027:errorcluster, "HasoEngine out"=w1028:refnum<class "HasoEngine.lvclass">, "HasoSlopes out"=w1011:refnum<class "HasoSlopes.lvclass">)  [unwired: 4 in, 1 out]
                    n314 = local read "Filter"() -> (w1023:u8[])
                    n315 = call "slopes2phase.vi"("TypePhase"=WavefrontReconstructionMode."Modal_Zernike", "Number of coefficients"=u8 32, "error in (no error)"=w1027, "Filter"=w1023, "HasoSlopes in"=w1011, "Phase in"=w1026) -> ("error out"=w1019:errorcluster, "HasoSlopes out"=w1020:refnum<class "HasoSlopes.lvclass">, "Phase out"=w1025:refnum<class "Phase.lvclass">)  [unwired: 3 in]
                    n316 = local read "idxType"() -> (w1013:enum16{"Wyant", "ANSI"})
                    n317 = call "slopes2zern.vi"("HasoSlopes in"=w1020, "error in (no error)"=w1019, "idxType"=w1013) -> ("HasoSlopes out"=w1017:refnum<class "HasoSlopes.lvclass">, "Zernike Coefficients"=w1012:dbl[], "error out"=w1018:errorcluster)  [unwired: 3 in, 2 out]
                    n318 = call <userlib>:"LVClass_Pupil ctor from HasoSlopes.vi"("Pupil in"=w1024, "HasoSlopes.lvclass"=w1011, "error in (no error)"=w1018) -> ("Pupil out"=w1035:refnum<class "Pupil.lvclass">, "error out"=w1036:errorcluster)  [unwired: 11 in]
                    n319 = case shown="True" w1016 {
                      tunnel: w1015 -> [_ w1045]
                      tunnel: w1014 -> [_ w1044]
                      tunnel: w1012 -> [_ w1043]
                      tunnel: w1011 -> [_ w1042]
                      frame False {
                      }
                      frame True {
                        n320 = stacked-sequence {
                          tunnel: w1045 -> [w1049 w1055]
                          tunnel: w1044 -> [w1048 w1054]
                          tunnel: w1043 -> [_ w1053]
                          tunnel: w1042 -> [w1046 _]
                          frame #0 {
                            n321 = Concatenate Strings(w1049, "_slopesMeas", ".has") -> (w1052:string)
                            n322 = Build Path(base path=w1048, name or relative path=w1052) -> (appended path=w1047:path)
                            n323 = call <userlib>:"LVClass_HasoSlopes Save.vi"("HasoSlopes in"=w1046, "path"=w1047) -> ()  [unwired: 12 in, 2 out]
                          }
                          frame #1 {
                            n324 = Concatenate Strings(w1055, "_zernCoefMeas", ".txt") -> (w1058:string)
                            n325 = Build Path(base path=w1054, name or relative path=w1058) -> (appended path=w1059:path)
                            n326 = Array To Spreadsheet String(array=w1053, 3:"%f") -> (spreadsheet string=w1060:string)  [unwired: 1 in]
                            n327 = Write to Text File(file (use dialog)=w1059, text=w1060) -> ()  [unwired: 2 in, 3 out]
                          }
                        }
                      }
                    }
                    n328 = call <userlib>:"LVClasse_Phase GetStatisticDatas.vi"("Phase in"=w1025, "error in (no error)"=w1036) -> ("Phase out"=w1041:refnum<class "Phase.lvclass">, "StatisticsData"=w1021:T2, "error out"=w1039:errorcluster)  [unwired: 11 in]
                    n329 = local write "Phase statistics"(w1021) -> ()
                    n330 = call <userlib>:"LVClasse_Phase Get Data.vi"("Phase in"=w1041, "Pupil"=w1035, "error in (no error)"=w1039) -> ("Phase out"=w1037:refnum<class "Phase.lvclass">, "data"=w1022:sgl[][], "Pupil (dup)"=w1038:refnum<class "Pupil.lvclass">, "error out"=w1040:errorcluster)  [unwired: 9 in]
                    n331 = local write "Zernike Measured"(w1012) -> ()
                    n332 = local write "Phase values"(w1022) -> ()
                  }
                  frame Error {
                  }
                }
              }
            }
          }
          frame #3 {
            # "Apply offset to DM"
            n333 = case shown="True" w1078 {
              tunnel: w1081 -> [_ w1089]
              tunnel: [w1082 w1083] -> w1080
              tunnel: w1079 -> [w1082 w1085]
              frame False {
              }
              frame True {
                # "Delay for DM response"
                n334 = local read "Initial offset"() -> (w1088:bool)
                n335 = case shown="True" w1088 {
                  tunnel: [w1094 w1099] -> w1086
                  frame False {
                    n336 = Initialize Array(0.0, 52) -> (w1094:dbl[])
                  }
                  frame True {
                    n337 = local read "Offset command file"() -> (w1098:path)
                    n338 = call-poly <vilib>:"Read From Spreadsheet File.vi"("format (%.3f)"="%.8f", "file path (dialog if empty)"=w1098) -> ("first row"=w1099:dbl[])  [unwired: 5 in, 4 out]
                  }
                }
                n339 = local write "Initial Positions"(w1086) -> ()
                n340 = call <userlib>:"LVClass_WavefrontCorrector Move to Absolute Position.vi"("WavefrontCorrector in"=w1089, "Absolute Positions"=w1086, "error in (no error)"=w1085) -> ("WavefrontCorrector out"=w1090:refnum<class "WavefrontCorrector.lvclass">, "error out"=w1091:errorcluster)  [unwired: 11 in]
                n341 = call <userlib>:"LVClass_WavefrontCorrector Get Current Position.vi"("WavefrontCorrector in"=w1090, "error in (no error)"=w1091) -> ("Wavefront Corrector Position"=w1087:T14, "error out"=w1084:errorcluster)  [unwired: 11 in, 1 out]
                n342 = local write "Initial Positions"(w1087) -> ()
                n343 = flat-sequence {
                  tunnel: [w1092] -> w1083
                  tunnel: w1084 -> [w1092]
                  frame #0 {
                    n344 = Wait (ms)(milliseconds to wait=u32 50) -> ()  [unwired: 1 out]
                  }
                }
              }
            }
          }
          frame #4 {
            n345 = case shown="True" w1102 {
              tunnel: w1113 -> [_ w1128]
              tunnel: w1112 -> [_ w1127]
              tunnel: w1111 -> [_ w1126]
              tunnel: w1110 -> [_ w1125]
              tunnel: w1109 -> [_ w1124]
              tunnel: w1101 -> [w1114 w1123]
              tunnel: w1108 -> [_ w1122]
              tunnel: w1107 -> [_ w1121]
              tunnel: w1106 -> [_ w1120]
              tunnel: w1105 -> [w1115 w1118]
              tunnel: [w1115 w1117] -> w1103
              tunnel: [w1114 w1116] -> w1100
              frame False {
              }
              frame True {
                n346 = local read "HASO ready"() -> (w1119:bool)
                n347 = case shown="True" w1119 {
                  tunnel: w1128 -> [_ w1156]
                  tunnel: w1126 -> [_ w1155]
                  tunnel: w1125 -> [_ w1154]
                  tunnel: [w1129 w1153] -> w1117
                  tunnel: w1127 -> [_ w1152]
                  tunnel: w1120 -> [_ w1136]
                  tunnel: w1118 -> [w1129 w1135]
                  tunnel: w1123 -> [w1132 w1140]
                  tunnel: w1122 -> [w1131 w1151]
                  tunnel: [w1132 w1142] -> w1116
                  tunnel: [w1131 w1150] -> _
                  tunnel: w1124 -> [w1133 w1149]
                  tunnel: w1121 -> [w1130 w1148]
                  tunnel: [w1133 w1147] -> _
                  tunnel: [w1130 w1146] -> _
                  frame False {
                  }
                  frame True {
                    n348 = property on="nb_images (set)" class="DigNum (strict)"() -> ("Value"=w1157:u32)  [unwired: 2 in, 2 out]
                    n349 = case shown="2, Default" w1157 {
                      tunnel: [w1259 w1261] -> w1138
                      tunnel: w1152 -> [w1258 _]
                      tunnel: w1156 -> [w1259 _]
                      tunnel: [w1258 w1260] -> w1137
                      tunnel: w1155 -> [_ w1261]
                      tunnel: w1154 -> [_ w1260]
                      frame 2, Default {
                      }
                      frame 1 {
                      }
                    }
                    n350 = stacked-sequence {
                      tunnel: w1138 -> [_ w1175]
                      tunnel: w1137 -> [_ w1174]
                      tunnel: [_ w1173] -> w1139
                      tunnel: [_ w1171] -> w1134
                      tunnel: [_ w1170] -> _
                      tunnel: w1136 -> [_ w1167]
                      tunnel: w1135 -> [_ w1166]
                      frame #0 {
                        # "Delay until MD gets stable"
                        n351 = local read "exposure_duration_s (set)"() -> (w1158:dbl)
                        n352 = local read "nb_images (set)"() -> (w1159:u32)
                        n353 = Multiply(x=w1158, y=w1159) -> (x*y=w1160:dbl)
                        n354 = Add(x=w1160, y=1.0) -> (x+y=w1161:dbl)
                        n355 = Multiply(x=w1161, y=1000.0) -> (x*y=w1165:dbl)
                        n356 = To Unsigned Long Integer(number=w1165) -> (unsigned 32bit integer=w1164:u32)
                        n357 = Wait (ms)(milliseconds to wait=w1164) -> ()  [unwired: 1 out]
                      }
                      frame #1 {
                        n358 = while {
                          tunnel: w1167 -> [w1180]
                          tunnel: [w1179] -> w1169
                          tunnel: w1166 -> [w1177]
                          tunnel: [w1176] -> w1168
                          stop <- w1178 stop-if-true
                          n359 = call <userlib>:"LVClass_Camera asynchroneImageReady.vi"("Camera in"=w1180, "error in (no error)"=w1177) -> ("Camera out"=w1179:refnum<class "Camera.lvclass">, "ready"=w1178:bool, "error out"=w1176:errorcluster)  [unwired: 11 in]
                        }
                        n360 = call <userlib>:"LVClass_Camera get image.vi"("Camera in"=w1169, "Image"=w1175, "Image RAW"=w1174, "remove_background"=FALSE, "error in (no error)"=w1168) -> ("Camera out"=w1170:refnum<class "Camera.lvclass">, "Image (dup)"=w1173:refnum<class "Image.lvclass">, "error out"=w1171:errorcluster)  [unwired: 7 in, 1 out]
                      }
                    }
                    n361 = case shown="No Error" w1134 {
                      selector: w1134 -> [w1255 w1256]
                      tunnel: w1139 -> [w1252 w1257]
                      tunnel: [w1251 w1257] -> w1145
                      tunnel: [w1250 w1256] -> w1144
                      frame No Error {
                        # "get image"
                        n362 = call <userlib>:"LVClass_Image get image data.vi"("Image in"=w1252, "error in (no error)"=w1255) -> ("Image out"=w1254:refnum<class "Image.lvclass">, "Image data out"=w1249:u32[][], "error out"=w1253:errorcluster)  [unwired: 11 in]
                        n363 = call <userlib>:"LVClass_Image get image information.vi"("Image in"=w1254, "error in (no error)"=w1253) -> ("Image out"=w1251:refnum<class "Image.lvclass">, "error out"=w1250:errorcluster)  [unwired: 11 in, 1 out]
                        n364 = local write "HASO intensity"(w1249) -> ()
                      }
                      frame Error {
                      }
                    }
                    n365 = case shown="No Error" w1144 {
                      selector: w1144 -> [w1207 w1248]
                      tunnel: [w1213 w1248] -> w1153
                      tunnel: w1145 -> [w1206 _]
                      tunnel: [w1211 w1245] -> w1146
                      tunnel: [w1210 w1247] -> w1147
                      tunnel: refnum<class "HasoSlopes.lvclass"> refnum ("HasoSlopes in") -> [w1203 w1244]
                      tunnel: w1151 -> [w1202 w1246]
                      tunnel: [w1201 w1246] -> w1150
                      tunnel: w1149 -> [w1200 w1247]
                      tunnel: w1148 -> [w1198 w1245]
                      tunnel: [w1183 w1243] -> w1142
                      tunnel: [w1181 w1244] -> w1141
                      tunnel: w1140 -> [w1182 w1243]
                      frame No Error {
                        # "phaseout"
                        n366 = local read "File Base Name"() -> (w1190:string)
                        n367 = local read "Save File"() -> (w1191:bool)
                        n368 = local read "Output path"() -> (w1189:path)
                        n369 = call "image2slopes.vi"("error in (no error)"=w1207, "Image in"=w1206, "HasoEngine in"=w1202, "HasoSlopes in"=w1203) -> ("error out"=w1185:errorcluster, "HasoEngine out"=w1201:refnum<class "HasoEngine.lvclass">, "HasoSlopes out"=w1181:refnum<class "HasoSlopes.lvclass">)  [unwired: 4 in, 1 out]
                        n370 = local read "Filter"() -> (w1197:u8[])
                        n371 = call <userlib>:"LVClass_HasoSlopes Apply Substractor.vi"("HasoSlopes in"=w1182, "HasoSlopes to substract"=w1181, "error in (no error)"=w1185) -> ("HasoSlopes out"=w1186:refnum<class "HasoSlopes.lvclass">, "error out"=w1184:errorcluster)  [unwired: 11 in]
                        n372 = call "slopes2phase.vi"("TypePhase"=WavefrontReconstructionMode."Modal_Zernike", "Number of coefficients"=u8 32, "error in (no error)"=w1184, "Filter"=w1197, "HasoSlopes in"=w1186, "Phase in"=w1200) -> ("error out"=w1193:errorcluster, "HasoSlopes out"=w1194:refnum<class "HasoSlopes.lvclass">, "Phase out"=w1199:refnum<class "Phase.lvclass">)  [unwired: 3 in]
                        n373 = local read "idxType"() -> (w1188:enum16{"Wyant", "ANSI"})
                        n374 = call "slopes2zern.vi"("HasoSlopes in"=w1194, "error in (no error)"=w1193, "idxType"=w1188) -> ("HasoSlopes out"=w1183:refnum<class "HasoSlopes.lvclass">, "Zernike Coefficients"=w1187:dbl[], "error out"=w1192:errorcluster)  [unwired: 3 in, 2 out]
                        n375 = call <userlib>:"LVClass_Pupil ctor from HasoSlopes.vi"("Pupil in"=w1198, "HasoSlopes.lvclass"=w1186, "error in (no error)"=w1192) -> ("Pupil out"=w1208:refnum<class "Pupil.lvclass">, "error out"=w1209:errorcluster)  [unwired: 11 in]
                        n376 = case shown="True" w1191 {
                          tunnel: w1190 -> [_ w1219]
                          tunnel: w1189 -> [_ w1218]
                          tunnel: w1187 -> [_ w1217]
                          tunnel: w1186 -> [_ w1215]
                          tunnel: w1181 -> [_ w1216]
                          frame False {
                          }
                          frame True {
                            n377 = stacked-sequence {
                              tunnel: w1219 -> [w1223 w1230 w1236]
                              tunnel: w1218 -> [w1222 w1229 w1235]
                              tunnel: w1217 -> [_ _ w1234]
                              tunnel: w1216 -> [w1220 _ _]
                              tunnel: w1215 -> [_ w1227 _]
                              frame #0 {
                                n378 = Concatenate Strings(w1223, "_slopesOffset", ".has") -> (w1226:string)
                                n379 = Build Path(base path=w1222, name or relative path=w1226) -> (appended path=w1221:path)
                                n380 = call <userlib>:"LVClass_HasoSlopes Save.vi"("HasoSlopes in"=w1220, "path"=w1221) -> ()  [unwired: 12 in, 2 out]
                              }
                              frame #1 {
                                n381 = Concatenate Strings(w1230, "_slopesNet", ".has") -> (w1233:string)
                                n382 = Build Path(base path=w1229, name or relative path=w1233) -> (appended path=w1228:path)
                                n383 = call <userlib>:"LVClass_HasoSlopes Save.vi"("HasoSlopes in"=w1227, "path"=w1228) -> ()  [unwired: 12 in, 2 out]
                              }
                              frame #2 {
                                n384 = Concatenate Strings(w1236, "_zernCoefNet", ".txt") -> (w1239:string)
                                n385 = Build Path(base path=w1235, name or relative path=w1239) -> (appended path=w1240:path)
                                n386 = Array To Spreadsheet String(array=w1234, 3:"%f") -> (spreadsheet string=w1241:string)  [unwired: 1 in]
                                n387 = Write to Text File(file (use dialog)=w1240, text=w1241) -> ()  [unwired: 2 in, 3 out]
                              }
                            }
                          }
                        }
                        n388 = call <userlib>:"LVClasse_Phase GetStatisticDatas.vi"("Phase in"=w1199, "error in (no error)"=w1209) -> ("Phase out"=w1214:refnum<class "Phase.lvclass">, "StatisticsData"=w1195:T2, "error out"=w1212:errorcluster)  [unwired: 11 in]
                        n389 = local write "Phase statistics"(w1195) -> ()
                        n390 = call <userlib>:"LVClasse_Phase Get Data.vi"("Phase in"=w1214, "Pupil"=w1208, "error in (no error)"=w1212) -> ("Phase out"=w1210:refnum<class "Phase.lvclass">, "data"=w1196:sgl[][], "Pupil (dup)"=w1211:refnum<class "Pupil.lvclass">, "error out"=w1213:errorcluster)  [unwired: 9 in]
                        n391 = local write "Zernike Measured"(w1187) -> ()
                        n392 = local write "Phase values"(w1196) -> ()
                      }
                      frame Error {
                      }
                    }
                    n393 = call <userlib>:"LVClass_HasoSlopes dtor.vi"("HasoSlopes in"=w1141) -> ()  [unwired: 13 in, 2 out]
                  }
                }
              }
            }
            n394 = Unbundle By Name(w1103) -> ("status"=w1104:bool)
          }
        }
      }
      event "Record Batch Zern": Mouse Up {
        n395 = event-data() -> ()  [unwired: 1 in, 8 out]
        n396 = local read "Idx start"() -> (w1262:u32)
        n397 = local read "Idx end"() -> (w1263:u32)
        n398 = Subtract(x=w1263, y=w1262) -> (x-y=w1264:u32)
        n399 = Increment(x=w1264) -> (x+1=w1265:u32)
        n400 = for {
          N: w1265 -> [_]
          tunnel: [w1304] -> w1283
          tunnel: w1277 -> [w1299]
          tunnel: w1276 -> [w1298]
          tunnel: w1275 -> [w1297]
          tunnel: w1274 -> [w1296]
          tunnel: w1271 -> [w1293]
          tunnel: w1270 -> [w1292]
          shift-right: [w1302] -> w1281
          shift-left: w1282 -> [w1303]
          shift-right: [w1300] -> w1278
          shift-left: w1280 -> [w1301]
          shift-right: [w1290] -> w1268
          shift-left: w1273 -> [w1295]
          shift-right: [w1291] -> w1269
          shift-left: w1272 -> [w1294]
          shift-right: [w1288] -> w1266
          shift-left: w1267 -> [w1289]
          tunnel: w1262 -> [w1285]
          i -> [w1286]
          n401 = Add(x=w1285, y=w1286) -> (x+y=w1284:u32)
          n402 = local read "Net Rp"() -> (w1287:bool)
          n403 = stacked-sequence {
            seq-local: [_ _ _ w1614 _] -> [_ _ _ _ w1639]
            seq-local: [_ _ w1479 _ _] -> [_ _ _ w1613 _]
            seq-local: [_ w1348 _ _ _] -> [_ _ w1480 _ _]
            seq-local: [_ _ w1478 _ _] -> [_ _ _ _ w1635]
            tunnel: [_ _ _ _ w1638] -> w1304
            tunnel: w1303 -> [_ w1361 _ _ _]
            tunnel: [_ _ _ _ w1637] -> w1302
            tunnel: w1301 -> [_ w1360 _ w1615 _]
            tunnel: [_ w1358 _ _ _] -> w1300
            tunnel: w1299 -> [_ _ w1492 _ w1647]
            tunnel: w1298 -> [_ _ w1491 _ w1646]
            tunnel: w1297 -> [_ _ w1490 _ w1645]
            tunnel: w1296 -> [_ _ w1489 _ w1644]
            tunnel: w1295 -> [_ _ w1488 _ w1643]
            tunnel: w1294 -> [_ _ w1487 _ _]
            tunnel: w1293 -> [_ _ w1486 _ w1642]
            tunnel: w1289 -> [_ _ w1485 _ w1641]
            tunnel: w1292 -> [_ _ w1484 _ w1640]
            tunnel: [_ _ _ _ w1634] -> w1291
            tunnel: [_ _ w1482 _ _] -> w1290
            tunnel: [_ _ w1481 _ _] -> w1288
            tunnel: w1287 -> [_ _ _ w1612 w1636]
            tunnel: w1284 -> [w1306 w1349 _ _ _]
            frame #0 {
              # "Create output folder path"
              n404 = Get Date/Time In Seconds() -> (seconds since 1Jan1904=w1327:timestamp)
              n405 = local read "Folder Name"() -> (w1319:string)
              n406 = local read "idxType"() -> (w1310:enum16{"Wyant", "ANSI"})
              n407 = Number To Decimal String(number=w1306) -> (decimal integer string=w1307:string)  [unwired: 1 in]
              n408 = Format Date/Time String(time format string (%c)="%Y%m%d", seconds (now)=w1327) -> (date/time string=w1326:string)  [unwired: 1 in]
              n409 = local read "Main Path"() -> (w1320:path)
              n410 = case shown="\"ANSI\"" w1310 {
                tunnel: ["Wyant" "ANSI"] -> w1309
                frame "Wyant", Default {
                }
                frame "ANSI" {
                }
              }
              n411 = local read "Subfolder"() -> (w1318:string)
              n412 = Concatenate Strings(w1326, "_", w1319) -> (w1325:string)
              n413 = Build Path(base path=w1320, name or relative path=w1325) -> (appended path=w1323:path)
              n414 = call <vilib>:"Check if File or Folder Exists.vi"("path"=w1323) -> ("error out"=w1316:errorcluster, "file or folder exists?"=w1329:bool)  [unwired: 8 in, 1 out]
              n415 = Concatenate Strings(w1309, "_idx_", w1307) -> (w1305:string)
              n416 = Build Path(base path=w1323, name or relative path=w1318) -> (appended path=w1314:path)
              n417 = Build Path(base path=w1314, name or relative path=w1305) -> (appended path=w1311:path)
              n418 = local write "Current status"(w1305) -> ()
              n419 = case shown="False" w1329 {
                tunnel: w1323 -> [w1345 _]
                tunnel: w1316 -> [w1344 w1346]
                tunnel: [w1343 w1346] -> w1315
                frame False {
                  n420 = Create Folder(path (use dialog)=w1345, error in=w1344) -> (error out=w1343:errorcluster)  [unwired: 1 in, 2 out]
                }
                frame True {
                }
              }
              n421 = call <vilib>:"Check if File or Folder Exists.vi"("error in (no error)"=w1315, "path"=w1314) -> ("error out"=w1313:errorcluster, "file or folder exists?"=w1317:bool)  [unwired: 7 in, 1 out]
              n422 = case shown="True" w1317 {
                tunnel: w1314 -> [w1334 _]
                tunnel: w1313 -> [w1333 w1335]
                tunnel: [w1332 w1335] -> w1312
                frame False {
                  n423 = Create Folder(path (use dialog)=w1334, error in=w1333) -> (error out=w1332:errorcluster)  [unwired: 1 in, 2 out]
                }
                frame True {
                }
              }
              n424 = call <vilib>:"Check if File or Folder Exists.vi"("error in (no error)"=w1312, "path"=w1311) -> ("error out"=w1324:errorcluster, "file or folder exists?"=w1328:bool)  [unwired: 7 in, 1 out]
              n425 = case shown="False" w1328 {
                tunnel: w1311 -> [w1337 w1341]
                tunnel: w1324 -> [w1336 w1342]
                frame False {
                  n426 = Create Folder(path (use dialog)=w1337, error in=w1336) -> ()  [unwired: 1 in, 3 out]
                }
                frame True {
                  n427 = Delete(path (use dialog)=w1341, entire hierarchy (F)=TRUE, error in=w1342) -> (deleted path=w1339:path, error out=w1338:errorcluster)  [unwired: 2 in, 1 out]
                  n428 = Create Folder(path (use dialog)=w1339, error in=w1338) -> ()  [unwired: 1 in, 3 out]
                }
              }
              n429 = local write "Output path"(w1311) -> ()
            }
            frame #1 {
              # "Delay for DM response"
              # "Apply command to DM"
              n430 = local read "Initial offset"() -> (w1359:bool)
              n431 = case shown="True" w1359 {
                tunnel: [w1447 w1452] -> w1350
                frame False {
                  n432 = Initialize Array(0.0, 52) -> (w1447:dbl[])
                }
                frame True {
                  n433 = local read "Offset command file"() -> (w1451:path)
                  n434 = call-poly <vilib>:"Read From Spreadsheet File.vi"("format (%.3f)"="%.8f", "file path (dialog if empty)"=w1451) -> ("first row"=w1452:dbl[])  [unwired: 5 in, 4 out]
                }
              }
              n435 = local read "Additional Command"() -> (w1365:bool)
              n436 = case shown="True" w1365 {
                tunnel: [w1454 w1477] -> w1351
                tunnel: [w1453 w1476] -> w1362
                tunnel: w1361 -> [w1453 w1475]
                tunnel: w1349 -> [_ w1458]
                frame False {
                  n437 = Initialize Array(0.0, 52) -> (w1454:dbl[])
                }
                frame True {
                  w1459 = 1
                  n438 = local read "Coef value"() -> (w1461:dbl)
                  n439 = local read "Initial haso file"() -> (w1465:path)
                  n440 = Initialize Array(w1458, w1459) -> (w1457:u32[])
                  n441 = Initialize Array(w1461, w1459) -> (w1460:dbl[])
                  n442 = local read "Haso configuration file"() -> (w1466:path)
                  n443 = local read "interaction matrix file"() -> (w1464:path)
                  n444 = local read "idxType"() -> (w1467:enum16{"Wyant", "ANSI"})
                  n445 = call "zern2command.vi"("Haso configuration file"=w1466, "idxType"=w1467, "interaction matrix file"=w1464, "error in (no error)"=w1475, "Zern coef in"=w1460, "Zern index in"=w1457, "Initial haso file"=w1465) -> ("error out"=w1468:errorcluster, "Offset Positions"=w1477:sgl[], "Zern pupil out"=w1469:refnum<class "Pupil.lvclass">, "ModalCoef out"=w1470:refnum<class "ModalCoef.lvclass">)  [unwired: 1 in]
                  n446 = call <userlib>:"LVClass_ModalCoef GetData.vi"("ModalCoef in"=w1470, "Pupil.lvclass"=w1469, "error in (no error)"=w1468) -> ("ModalCoef out"=w1474:refnum<class "ModalCoef.lvclass">, "coef"=w1463:sgl[], "index"=w1462:u32[], "Pupil.lvclass (dup)"=w1473:refnum<class "Pupil.lvclass">, "error out"=w1472:errorcluster)  [unwired: 8 in]
                  n447 = local write "Index out"(w1462) -> ()
                  n448 = call <userlib>:"LVClass_Pupil dtor.vi"("Pupil in"=w1473, "error in (no error)"=w1472) -> ("error out"=w1471:errorcluster)  [unwired: 12 in, 1 out]
                  n449 = local write "Coef out"(w1463) -> ()
                  n450 = call <userlib>:"LVClass_ModalCoef dtor.vi"("ModalCoef in"=w1474, "error in (no error)"=w1471) -> ("error out"=w1476:errorcluster)  [unwired: 12 in, 1 out]
                }
              }
              n451 = local read "File Base Name"() -> (w1352:string)
              n452 = local read "Output path"() -> (w1356:path)
              n453 = local read "Input type"() -> (w1353:T4)
              n454 = local read "Save File"() -> (w1357:bool)
              n455 = local write "Initial Positions"(w1350) -> ()
              n456 = Add(x=w1351, y=w1350) -> (x+y=w1354:dbl[])
              n457 = call <userlib>:"LVClass_WavefrontCorrector Move to Absolute Position.vi"("WavefrontCorrector in"=w1360, "Absolute Positions"=w1354, "error in (no error)"=w1362) -> ("WavefrontCorrector out"=w1363:refnum<class "WavefrontCorrector.lvclass">, "error out"=w1364:errorcluster)  [unwired: 11 in]
              n458 = call <userlib>:"LVClass_WavefrontCorrector Get Current Position.vi"("WavefrontCorrector in"=w1363, "error in (no error)"=w1364) -> ("WavefrontCorrector out"=w1358:refnum<class "WavefrontCorrector.lvclass">, "Wavefront Corrector Position"=w1355:T14, "error out"=w1347:errorcluster)  [unwired: 11 in]
              n459 = case shown="True" w1357 {
                tunnel: w1356 -> [_ w1374]
                tunnel: w1352 -> [_ w1373]
                tunnel: w1350 -> [_ w1372]
                tunnel: w1351 -> [_ w1371]
                tunnel: w1354 -> [_ w1370]
                tunnel: w1353 -> [_ w1369]
                tunnel: w1355 -> [_ w1368]
                frame False {
                }
                frame True {
                  n460 = stacked-sequence {
                    tunnel: w1374 -> [w1379 w1388 w1397 w1406 w1413 w1425 w1437]
                    tunnel: w1373 -> [w1377 w1386 w1395 w1404 w1412 w1424 w1436]
                    tunnel: w1372 -> [w1375 _ _ _ _ _ _]
                    tunnel: w1371 -> [_ w1384 _ _ _ _ _]
                    tunnel: w1370 -> [_ _ w1393 _ _ _ _]
                    tunnel: w1369 -> [_ _ _ _ w1411 w1423 w1435]
                    tunnel: w1368 -> [_ _ _ w1402 _ _ _]
                    frame #0 {
                      n461 = Concatenate Strings(w1377, "_cmdOffset", ".dat") -> (w1380:string)
                      n462 = Build Path(base path=w1379, name or relative path=w1380) -> (appended path=w1381:path)
                      n463 = Array To Spreadsheet String(array=w1375, 3:"%f") -> (spreadsheet string=w1382:string)  [unwired: 1 in]
                      n464 = Write to Text File(file (use dialog)=w1381, text=w1382) -> ()  [unwired: 2 in, 3 out]
                    }
                    frame #1 {
                      n465 = Concatenate Strings(w1386, "_cmdAdd", ".dat") -> (w1389:string)
                      n466 = Build Path(base path=w1388, name or relative path=w1389) -> (appended path=w1390:path)
                      n467 = Array To Spreadsheet String(array=w1384, 3:"%f") -> (spreadsheet string=w1391:string)  [unwired: 1 in]
                      n468 = Write to Text File(file (use dialog)=w1390, text=w1391) -> ()  [unwired: 2 in, 3 out]
                    }
                    frame #2 {
                      n469 = Concatenate Strings(w1395, "_cmdFinal", ".dat") -> (w1398:string)
                      n470 = Build Path(base path=w1397, name or relative path=w1398) -> (appended path=w1399:path)
                      n471 = Array To Spreadsheet String(array=w1393, 3:"%f") -> (spreadsheet string=w1400:string)  [unwired: 1 in]
                      n472 = Write to Text File(file (use dialog)=w1399, text=w1400) -> ()  [unwired: 2 in, 3 out]
                    }
                    frame #3 {
                      n473 = Concatenate Strings(w1404, "_cmdFinalMirror", ".dat") -> (w1407:string)
                      n474 = Build Path(base path=w1406, name or relative path=w1407) -> (appended path=w1408:path)
                      n475 = Array To Spreadsheet String(array=w1402, 3:"%f") -> (spreadsheet string=w1409:string)  [unwired: 1 in]
                      n476 = Write to Text File(file (use dialog)=w1408, text=w1409) -> ()  [unwired: 2 in, 3 out]
                    }
                    frame #4 {
                      n477 = case shown="\"Zernike Coef\", Default" w1411 {
                        tunnel: w1413 -> [_ w1418]
                        tunnel: w1412 -> [_ w1416]
                        frame "Zero Input" {
                        }
                        frame "Zernike Coef", Default {
                          n478 = local read "Zern/DM coef in"() -> (w1414:sgl[])
                          n479 = Concatenate Strings(w1416, "_zernCoef", ".txt") -> (w1419:string)
                          n480 = Build Path(base path=w1418, name or relative path=w1419) -> (appended path=w1420:path)
                          n481 = Array To Spreadsheet String(array=w1414, 3:"%f") -> (spreadsheet string=w1421:string)  [unwired: 1 in]
                          n482 = Write to Text File(file (use dialog)=w1420, text=w1421) -> ()  [unwired: 2 in, 3 out]
                        }
                      }
                    }
                    frame #5 {
                      n483 = case shown="\"Zernike Coef\", Default" w1423 {
                        tunnel: w1425 -> [_ w1430]
                        tunnel: w1424 -> [_ w1428]
                        frame "Zero Input" {
                        }
                        frame "Zernike Coef", Default {
                          n484 = local read "Zern/DM index in"() -> (w1426:i32[])
                          n485 = Concatenate Strings(w1428, "_zernIdx", ".txt") -> (w1431:string)
                          n486 = Build Path(base path=w1430, name or relative path=w1431) -> (appended path=w1432:path)
                          n487 = Array To Spreadsheet String(array=w1426, 3:"%d") -> (spreadsheet string=w1433:string)  [unwired: 1 in]
                          n488 = Write to Text File(file (use dialog)=w1432, text=w1433) -> ()  [unwired: 2 in, 3 out]
                        }
                      }
                    }
                    frame #6 {
                      n489 = case shown="\"Zernike Coef\", Default" w1435 {
                        tunnel: w1437 -> [_ w1442]
                        tunnel: w1436 -> [_ w1440]
                        frame "Zero Input" {
                        }
                        frame "Zernike Coef", Default {
                          n490 = Concatenate Strings(w1440, "_zernCoefWyant", ".txt") -> (w1443:string)
                          n491 = local read "Coef out"() -> (w1438:sgl[])
                          n492 = Build Path(base path=w1442, name or relative path=w1443) -> (appended path=w1444:path)
                          n493 = Array To Spreadsheet String(array=w1438, 3:"%f") -> (spreadsheet string=w1445:string)  [unwired: 1 in]
                          n494 = Write to Text File(file (use dialog)=w1444, text=w1445) -> ()  [unwired: 2 in, 3 out]
                        }
                      }
                    }
                  }
                }
              }
              n495 = local write "Final Positions"(w1354) -> ()
              n496 = local write "DM Actuator Values"(w1355) -> ()
              n497 = flat-sequence {
                tunnel: [w1366] -> w1348
                tunnel: w1347 -> [w1366]
                frame #0 {
                  n498 = Wait (ms)(milliseconds to wait=u32 50) -> ()  [unwired: 1 out]
                }
              }
            }
            frame #2 {
              n499 = local read "HASO ready"() -> (w1483:bool)
              n500 = case shown="True" w1483 {
                tunnel: w1492 -> [_ w1518]
                tunnel: w1490 -> [_ w1517]
                tunnel: w1489 -> [_ w1516]
                tunnel: [w1493 w1515] -> w1479
                tunnel: w1491 -> [_ w1514]
                tunnel: w1484 -> [_ w1501]
                tunnel: w1480 -> [w1493 w1500]
                tunnel: w1487 -> [w1496 w1513]
                tunnel: w1486 -> [w1495 w1512]
                tunnel: [w1496 w1511] -> w1478
                tunnel: [w1495 w1510] -> _
                tunnel: w1488 -> [w1497 w1509]
                tunnel: w1485 -> [w1494 w1508]
                tunnel: [w1497 w1507] -> w1482
                tunnel: [w1494 w1506] -> w1481
                frame False {
                }
                frame True {
                  n501 = property on="nb_images (set)" class="DigNum (strict)"() -> ("Value"=w1519:u32)  [unwired: 2 in, 2 out]
                  n502 = case shown="2, Default" w1519 {
                    tunnel: [w1609 w1611] -> w1499
                    tunnel: w1514 -> [w1608 _]
                    tunnel: w1518 -> [w1609 _]
                    tunnel: [w1608 w1610] -> w1498
                    tunnel: w1517 -> [_ w1611]
                    tunnel: w1516 -> [_ w1610]
                    frame 2, Default {
                    }
                    frame 1 {
                    }
                  }
                  n503 = stacked-sequence {
                    tunnel: w1499 -> [_ w1537]
                    tunnel: w1498 -> [_ w1536]
                    tunnel: [_ w1535] -> w1502
                    tunnel: [_ w1533] -> w1503
                    tunnel: [_ w1532] -> _
                    tunnel: w1501 -> [_ w1529]
                    tunnel: w1500 -> [_ w1528]
                    frame #0 {
                      # "Delay until MD gets stable"
                      n504 = local read "exposure_duration_s (set)"() -> (w1520:dbl)
                      n505 = local read "nb_images (set)"() -> (w1521:u32)
                      n506 = Multiply(x=w1520, y=w1521) -> (x*y=w1522:dbl)
                      n507 = Add(x=w1522, y=3.0) -> (x+y=w1523:dbl)
                      n508 = Multiply(x=w1523, y=1000.0) -> (x*y=w1527:dbl)
                      n509 = To Unsigned Long Integer(number=w1527) -> (unsigned 32bit integer=w1526:u32)
                      n510 = Wait (ms)(milliseconds to wait=w1526) -> ()  [unwired: 1 out]
                    }
                    frame #1 {
                      n511 = while {
                        tunnel: w1529 -> [w1542]
                        tunnel: [w1541] -> w1531
                        tunnel: w1528 -> [w1539]
                        tunnel: [w1538] -> w1530
                        stop <- w1540 stop-if-true
                        n512 = call <userlib>:"LVClass_Camera asynchroneImageReady.vi"("Camera in"=w1542, "error in (no error)"=w1539) -> ("Camera out"=w1541:refnum<class "Camera.lvclass">, "ready"=w1540:bool, "error out"=w1538:errorcluster)  [unwired: 11 in]
                      }
                      n513 = call <userlib>:"LVClass_Camera get image.vi"("Camera in"=w1531, "Image"=w1537, "Image RAW"=w1536, "remove_background"=FALSE, "error in (no error)"=w1530) -> ("Camera out"=w1532:refnum<class "Camera.lvclass">, "Image (dup)"=w1535:refnum<class "Image.lvclass">, "error out"=w1533:errorcluster)  [unwired: 7 in, 1 out]
                    }
                  }
                  n514 = case shown="No Error" w1503 {
                    selector: w1503 -> [w1605 w1606]
                    tunnel: w1502 -> [w1599 w1607]
                    tunnel: [w1602 w1607] -> w1505
                    tunnel: [w1601 w1606] -> w1504
                    frame No Error {
                      # "get image"
                      n515 = call <userlib>:"LVClass_Image get image data.vi"("Image in"=w1599, "error in (no error)"=w1605) -> ("Image out"=w1604:refnum<class "Image.lvclass">, "Image data out"=w1600:u32[][], "error out"=w1603:errorcluster)  [unwired: 11 in]
                      n516 = call <userlib>:"LVClass_Image get image information.vi"("Image in"=w1604, "error in (no error)"=w1603) -> ("Image out"=w1602:refnum<class "Image.lvclass">, "error out"=w1601:errorcluster)  [unwired: 11 in, 1 out]
                      n517 = local write "HASO intensity"(w1600) -> ()
                    }
                    frame Error {
                    }
                  }
                  n518 = case shown="No Error" w1504 {
                    selector: w1504 -> [w1566 w1598]
                    tunnel: [w1572 w1598] -> w1515
                    tunnel: w1505 -> [w1565 _]
                    tunnel: [w1570 w1594] -> w1506
                    tunnel: [w1569 w1597] -> w1507
                    tunnel: w1513 -> [w1562 w1596]
                    tunnel: w1512 -> [w1561 w1595]
                    tunnel: [w1549 w1596] -> w1511
                    tunnel: [w1560 w1595] -> w1510
                    tunnel: w1509 -> [w1558 w1597]
                    tunnel: w1508 -> [w1556 w1594]
                    frame No Error {
                      # "phaseout"
                      n519 = local read "File Base Name"() -> (w1547:string)
                      n520 = local read "Save File"() -> (w1548:bool)
                      n521 = local read "Output path"() -> (w1546:path)
                      n522 = call "image2slopes.vi"("error in (no error)"=w1566, "Image in"=w1565, "HasoEngine in"=w1561, "HasoSlopes in"=w1562) -> ("error out"=w1559:errorcluster, "HasoEngine out"=w1560:refnum<class "HasoEngine.lvclass">, "HasoSlopes out"=w1543:refnum<class "HasoSlopes.lvclass">)  [unwired: 4 in, 1 out]
                      n523 = local read "Filter"() -> (w1555:u8[])
                      n524 = call "slopes2phase.vi"("TypePhase"=WavefrontReconstructionMode."Modal_Zernike", "Number of coefficients"=u8 32, "error in (no error)"=w1559, "Filter"=w1555, "HasoSlopes in"=w1543, "Phase in"=w1558) -> ("error out"=w1551:errorcluster, "HasoSlopes out"=w1552:refnum<class "HasoSlopes.lvclass">, "Phase out"=w1557:refnum<class "Phase.lvclass">)  [unwired: 3 in]
                      n525 = local read "idxType"() -> (w1545:enum16{"Wyant", "ANSI"})
                      n526 = call "slopes2zern.vi"("HasoSlopes in"=w1552, "error in (no error)"=w1551, "idxType"=w1545) -> ("HasoSlopes out"=w1549:refnum<class "HasoSlopes.lvclass">, "Zernike Coefficients"=w1544:dbl[], "error out"=w1550:errorcluster)  [unwired: 3 in, 2 out]
                      n527 = call <userlib>:"LVClass_Pupil ctor from HasoSlopes.vi"("Pupil in"=w1556, "HasoSlopes.lvclass"=w1543, "error in (no error)"=w1550) -> ("Pupil out"=w1567:refnum<class "Pupil.lvclass">, "error out"=w1568:errorcluster)  [unwired: 11 in]
                      n528 = case shown="True" w1548 {
                        tunnel: w1547 -> [_ w1577]
                        tunnel: w1546 -> [_ w1576]
                        tunnel: w1544 -> [_ w1575]
                        tunnel: w1543 -> [_ w1574]
                        frame False {
                        }
                        frame True {
                          n529 = stacked-sequence {
                            tunnel: w1577 -> [w1581 w1587]
                            tunnel: w1576 -> [w1580 w1586]
                            tunnel: w1575 -> [_ w1585]
                            tunnel: w1574 -> [w1578 _]
                            frame #0 {
                              n530 = Concatenate Strings(w1581, "_slopesMeas", ".has") -> (w1584:string)
                              n531 = Build Path(base path=w1580, name or relative path=w1584) -> (appended path=w1579:path)
                              n532 = call <userlib>:"LVClass_HasoSlopes Save.vi"("HasoSlopes in"=w1578, "path"=w1579) -> ()  [unwired: 12 in, 2 out]
                            }
                            frame #1 {
                              n533 = Concatenate Strings(w1587, "_zernCoefMeas", ".txt") -> (w1590:string)
                              n534 = Build Path(base path=w1586, name or relative path=w1590) -> (appended path=w1591:path)
                              n535 = Array To Spreadsheet String(array=w1585, 3:"%f") -> (spreadsheet string=w1592:string)  [unwired: 1 in]
                              n536 = Write to Text File(file (use dialog)=w1591, text=w1592) -> ()  [unwired: 2 in, 3 out]
                            }
                          }
                        }
                      }
                      n537 = call <userlib>:"LVClasse_Phase GetStatisticDatas.vi"("Phase in"=w1557, "error in (no error)"=w1568) -> ("Phase out"=w1573:refnum<class "Phase.lvclass">, "StatisticsData"=w1553:T2, "error out"=w1571:errorcluster)  [unwired: 11 in]
                      n538 = local write "Phase statistics"(w1553) -> ()
                      n539 = call <userlib>:"LVClasse_Phase Get Data.vi"("Phase in"=w1573, "Pupil"=w1567, "error in (no error)"=w1571) -> ("Phase out"=w1569:refnum<class "Phase.lvclass">, "data"=w1554:sgl[][], "Pupil (dup)"=w1570:refnum<class "Pupil.lvclass">, "error out"=w1572:errorcluster)  [unwired: 9 in]
                      n540 = local write "Zernike Measured"(w1544) -> ()
                      n541 = local write "Phase values"(w1554) -> ()
                    }
                    frame Error {
                    }
                  }
                }
              }
            }
            frame #3 {
              # "Apply offset to DM"
              n542 = case shown="True" w1612 {
                tunnel: w1615 -> [_ w1623]
                tunnel: [w1616 w1618] -> w1614
                tunnel: w1613 -> [w1616 w1619]
                frame False {
                }
                frame True {
                  # "Delay for DM response"
                  n543 = local read "Initial offset"() -> (w1622:bool)
                  n544 = case shown="True" w1622 {
                    tunnel: [w1628 w1633] -> w1620
                    frame False {
                      n545 = Initialize Array(0.0, 52) -> (w1628:dbl[])
                    }
                    frame True {
                      n546 = local read "Offset command file"() -> (w1632:path)
                      n547 = call-poly <vilib>:"Read From Spreadsheet File.vi"("format (%.3f)"="%.8f", "file path (dialog if empty)"=w1632) -> ("first row"=w1633:dbl[])  [unwired: 5 in, 4 out]
                    }
                  }
                  n548 = local write "Initial Positions"(w1620) -> ()
                  n549 = call <userlib>:"LVClass_WavefrontCorrector Move to Absolute Position.vi"("WavefrontCorrector in"=w1623, "Absolute Positions"=w1620, "error in (no error)"=w1619) -> ("WavefrontCorrector out"=w1624:refnum<class "WavefrontCorrector.lvclass">, "error out"=w1625:errorcluster)  [unwired: 11 in]
                  n550 = call <userlib>:"LVClass_WavefrontCorrector Get Current Position.vi"("WavefrontCorrector in"=w1624, "error in (no error)"=w1625) -> ("Wavefront Corrector Position"=w1621:T14, "error out"=w1617:errorcluster)  [unwired: 11 in, 1 out]
                  n551 = local write "Initial Positions"(w1621) -> ()
                  n552 = flat-sequence {
                    tunnel: [w1626] -> w1618
                    tunnel: w1617 -> [w1626]
                    frame #0 {
                      n553 = Wait (ms)(milliseconds to wait=u32 50) -> ()  [unwired: 1 out]
                    }
                  }
                }
              }
            }
            frame #4 {
              n554 = case shown="True" w1636 {
                tunnel: w1647 -> [_ w1662]
                tunnel: w1646 -> [_ w1661]
                tunnel: w1645 -> [_ w1660]
                tunnel: w1644 -> [_ w1659]
                tunnel: w1643 -> [_ w1658]
                tunnel: w1635 -> [w1648 w1657]
                tunnel: w1642 -> [_ w1656]
                tunnel: w1641 -> [_ w1655]
                tunnel: w1640 -> [_ w1654]
                tunnel: w1639 -> [w1649 w1652]
                tunnel: [w1649 w1651] -> w1637
                tunnel: [w1648 w1650] -> w1634
                frame False {
                }
                frame True {
                  n555 = local read "HASO ready"() -> (w1653:bool)
                  n556 = case shown="True" w1653 {
                    tunnel: w1662 -> [_ w1690]
                    tunnel: w1660 -> [_ w1689]
                    tunnel: w1659 -> [_ w1688]
                    tunnel: [w1663 w1687] -> w1651
                    tunnel: w1661 -> [_ w1686]
                    tunnel: w1654 -> [_ w1671]
                    tunnel: w1652 -> [w1663 w1670]
                    tunnel: w1657 -> [w1666 w1674]
                    tunnel: w1656 -> [w1665 w1685]
                    tunnel: [w1666 w1676] -> w1650
                    tunnel: [w1665 w1684] -> _
                    tunnel: w1658 -> [w1667 w1683]
                    tunnel: w1655 -> [w1664 w1682]
                    tunnel: [w1667 w1681] -> _
                    tunnel: [w1664 w1680] -> _
                    frame False {
                    }
                    frame True {
                      n557 = property on="nb_images (set)" class="DigNum (strict)"() -> ("Value"=w1691:u32)  [unwired: 2 in, 2 out]
                      n558 = case shown="2, Default" w1691 {
                        tunnel: [w1793 w1795] -> w1673
                        tunnel: w1686 -> [w1792 _]
                        tunnel: w1690 -> [w1793 _]
                        tunnel: [w1792 w1794] -> w1672
                        tunnel: w1689 -> [_ w1795]
                        tunnel: w1688 -> [_ w1794]
                        frame 2, Default {
                        }
                        frame 1 {
                        }
                      }
                      n559 = stacked-sequence {
                        tunnel: w1673 -> [_ w1709]
                        tunnel: w1672 -> [_ w1708]
                        tunnel: [_ w1707] -> w1669
                        tunnel: [_ w1705] -> w1668
                        tunnel: [_ w1704] -> _
                        tunnel: w1671 -> [_ w1701]
                        tunnel: w1670 -> [_ w1700]
                        frame #0 {
                          # "Delay until MD gets stable"
                          n560 = local read "exposure_duration_s (set)"() -> (w1692:dbl)
                          n561 = local read "nb_images (set)"() -> (w1693:u32)
                          n562 = Multiply(x=w1692, y=w1693) -> (x*y=w1694:dbl)
                          n563 = Add(x=w1694, y=3.0) -> (x+y=w1695:dbl)
                          n564 = Multiply(x=w1695, y=1000.0) -> (x*y=w1699:dbl)
                          n565 = To Unsigned Long Integer(number=w1699) -> (unsigned 32bit integer=w1698:u32)
                          n566 = Wait (ms)(milliseconds to wait=w1698) -> ()  [unwired: 1 out]
                        }
                        frame #1 {
                          n567 = while {
                            tunnel: w1701 -> [w1714]
                            tunnel: [w1713] -> w1703
                            tunnel: w1700 -> [w1711]
                            tunnel: [w1710] -> w1702
                            stop <- w1712 stop-if-true
                            n568 = call <userlib>:"LVClass_Camera asynchroneImageReady.vi"("Camera in"=w1714, "error in (no error)"=w1711) -> ("Camera out"=w1713:refnum<class "Camera.lvclass">, "ready"=w1712:bool, "error out"=w1710:errorcluster)  [unwired: 11 in]
                          }
                          n569 = call <userlib>:"LVClass_Camera get image.vi"("Camera in"=w1703, "Image"=w1709, "Image RAW"=w1708, "remove_background"=FALSE, "error in (no error)"=w1702) -> ("Camera out"=w1704:refnum<class "Camera.lvclass">, "Image (dup)"=w1707:refnum<class "Image.lvclass">, "error out"=w1705:errorcluster)  [unwired: 7 in, 1 out]
                        }
                      }
                      n570 = case shown="No Error" w1668 {
                        selector: w1668 -> [w1789 w1790]
                        tunnel: w1669 -> [w1786 w1791]
                        tunnel: [w1785 w1791] -> w1679
                        tunnel: [w1784 w1790] -> w1678
                        frame No Error {
                          # "get image"
                          n571 = call <userlib>:"LVClass_Image get image data.vi"("Image in"=w1786, "error in (no error)"=w1789) -> ("Image out"=w1788:refnum<class "Image.lvclass">, "Image data out"=w1783:u32[][], "error out"=w1787:errorcluster)  [unwired: 11 in]
                          n572 = call <userlib>:"LVClass_Image get image information.vi"("Image in"=w1788, "error in (no error)"=w1787) -> ("Image out"=w1785:refnum<class "Image.lvclass">, "error out"=w1784:errorcluster)  [unwired: 11 in, 1 out]
                          n573 = local write "HASO intensity"(w1783) -> ()
                        }
                        frame Error {
                        }
                      }
                      n574 = case shown="No Error" w1678 {
                        selector: w1678 -> [w1741 w1782]
                        tunnel: [w1747 w1782] -> w1687
                        tunnel: w1679 -> [w1740 _]
                        tunnel: [w1745 w1779] -> w1680
                        tunnel: [w1744 w1781] -> w1681
                        tunnel: refnum<class "HasoSlopes.lvclass"> refnum ("HasoSlopes in") -> [w1737 w1778]
                        tunnel: w1685 -> [w1736 w1780]
                        tunnel: [w1735 w1780] -> w1684
                        tunnel: w1683 -> [w1734 w1781]
                        tunnel: w1682 -> [w1732 w1779]
                        tunnel: [w1717 w1777] -> w1676
                        tunnel: [w1715 w1778] -> w1675
                        tunnel: w1674 -> [w1716 w1777]
                        frame No Error {
                          # "phaseout"
                          n575 = local read "File Base Name"() -> (w1724:string)
                          n576 = local read "Save File"() -> (w1725:bool)
                          n577 = local read "Output path"() -> (w1723:path)
                          n578 = call "image2slopes.vi"("error in (no error)"=w1741, "Image in"=w1740, "HasoEngine in"=w1736, "HasoSlopes in"=w1737) -> ("error out"=w1719:errorcluster, "HasoEngine out"=w1735:refnum<class "HasoEngine.lvclass">, "HasoSlopes out"=w1715:refnum<class "HasoSlopes.lvclass">)  [unwired: 4 in, 1 out]
                          n579 = local read "Filter"() -> (w1731:u8[])
                          n580 = call <userlib>:"LVClass_HasoSlopes Apply Substractor.vi"("HasoSlopes in"=w1716, "HasoSlopes to substract"=w1715, "error in (no error)"=w1719) -> ("HasoSlopes out"=w1720:refnum<class "HasoSlopes.lvclass">, "error out"=w1718:errorcluster)  [unwired: 11 in]
                          n581 = call "slopes2phase.vi"("TypePhase"=WavefrontReconstructionMode."Modal_Zernike", "Number of coefficients"=u8 32, "error in (no error)"=w1718, "Filter"=w1731, "HasoSlopes in"=w1720, "Phase in"=w1734) -> ("error out"=w1727:errorcluster, "HasoSlopes out"=w1728:refnum<class "HasoSlopes.lvclass">, "Phase out"=w1733:refnum<class "Phase.lvclass">)  [unwired: 3 in]
                          n582 = local read "idxType"() -> (w1722:enum16{"Wyant", "ANSI"})
                          n583 = call "slopes2zern.vi"("HasoSlopes in"=w1728, "error in (no error)"=w1727, "idxType"=w1722) -> ("HasoSlopes out"=w1717:refnum<class "HasoSlopes.lvclass">, "Zernike Coefficients"=w1721:dbl[], "error out"=w1726:errorcluster)  [unwired: 3 in, 2 out]
                          n584 = call <userlib>:"LVClass_Pupil ctor from HasoSlopes.vi"("Pupil in"=w1732, "HasoSlopes.lvclass"=w1720, "error in (no error)"=w1726) -> ("Pupil out"=w1742:refnum<class "Pupil.lvclass">, "error out"=w1743:errorcluster)  [unwired: 11 in]
                          n585 = case shown="True" w1725 {
                            tunnel: w1724 -> [_ w1753]
                            tunnel: w1723 -> [_ w1752]
                            tunnel: w1721 -> [_ w1751]
                            tunnel: w1720 -> [_ w1749]
                            tunnel: w1715 -> [_ w1750]
                            frame False {
                            }
                            frame True {
                              n586 = stacked-sequence {
                                tunnel: w1753 -> [w1757 w1764 w1770]
                                tunnel: w1752 -> [w1756 w1763 w1769]
                                tunnel: w1751 -> [_ _ w1768]
                                tunnel: w1750 -> [w1754 _ _]
                                tunnel: w1749 -> [_ w1761 _]
                                frame #0 {
                                n587 = Concatenate Strings(w1757, "_slopesOffset", ".has") -> (w1760:string)
                                n588 = Build Path(base path=w1756, name or relative path=w1760) -> (appended path=w1755:path)
                                n589 = call <userlib>:"LVClass_HasoSlopes Save.vi"("HasoSlopes in"=w1754, "path"=w1755) -> ()  [unwired: 12 in, 2 out]
                                }
                                frame #1 {
                                n590 = Concatenate Strings(w1764, "_slopesNet", ".has") -> (w1767:string)
                                n591 = Build Path(base path=w1763, name or relative path=w1767) -> (appended path=w1762:path)
                                n592 = call <userlib>:"LVClass_HasoSlopes Save.vi"("HasoSlopes in"=w1761, "path"=w1762) -> ()  [unwired: 12 in, 2 out]
                                }
                                frame #2 {
                                n593 = Concatenate Strings(w1770, "_zernCoefNet", ".txt") -> (w1773:string)
                                n594 = Build Path(base path=w1769, name or relative path=w1773) -> (appended path=w1774:path)
                                n595 = Array To Spreadsheet String(array=w1768, 3:"%f") -> (spreadsheet string=w1775:string)  [unwired: 1 in]
                                n596 = Write to Text File(file (use dialog)=w1774, text=w1775) -> ()  [unwired: 2 in, 3 out]
                                }
                              }
                            }
                          }
                          n597 = call <userlib>:"LVClasse_Phase GetStatisticDatas.vi"("Phase in"=w1733, "error in (no error)"=w1743) -> ("Phase out"=w1748:refnum<class "Phase.lvclass">, "StatisticsData"=w1729:T2, "error out"=w1746:errorcluster)  [unwired: 11 in]
                          n598 = local write "Phase statistics"(w1729) -> ()
                          n599 = call <userlib>:"LVClasse_Phase Get Data.vi"("Phase in"=w1748, "Pupil"=w1742, "error in (no error)"=w1746) -> ("Phase out"=w1744:refnum<class "Phase.lvclass">, "data"=w1730:sgl[][], "Pupil (dup)"=w1745:refnum<class "Pupil.lvclass">, "error out"=w1747:errorcluster)  [unwired: 9 in]
                          n600 = local write "Zernike Measured"(w1721) -> ()
                          n601 = local write "Phase values"(w1730) -> ()
                        }
                        frame Error {
                        }
                      }
                      n602 = call <userlib>:"LVClass_HasoSlopes dtor.vi"("HasoSlopes in"=w1675) -> ()  [unwired: 13 in, 2 out]
                    }
                  }
                }
              }
              n603 = Unbundle By Name(w1637) -> ("status"=w1638:bool)
            }
          }
        }
      }
      event "Record Batch Actuator": Mouse Up {
        n604 = event-data() -> ()  [unwired: 1 in, 8 out]
        n605 = local read "Coef value"() -> (w1796:dbl)
        n606 = local read "Idx start"() -> (w1804:u32)
        n607 = Greater Than 0?(x=w1804) -> (x > 0?=w1805:bool)
        n608 = local read "Idx end"() -> (w1802:u32)
        n609 = Less Or Equal?(x=w1802, y=52) -> (x <= y?=w1806:bool)
        n610 = Subtract(x=w1802, y=w1804) -> (x-y=w1807:u32)
        n611 = In Range and Coerce(upper limit=0.8, x=w1796, lower limit=-0.8) -> (In Range?=w1799:bool)  [unwired: 1 out]
        n612 = And(x=w1805, y=w1806) -> (x .and. y?=w1798:bool)
        n613 = Increment(x=w1807) -> (x+1=w1808:u32)
        n614 = And(x=w1798, y=w1799) -> (x .and. y?=w1797:bool)
        n615 = case shown="True" w1797 {
          tunnel: [FALSE w1852] -> w1826
          tunnel: w1825 -> [w1828 w1851]
          tunnel: [w1828 w1850] -> w1824
          tunnel: w1823 -> [w1829 w1849]
          tunnel: [w1829 w1848] -> w1821
          tunnel: w1820 -> [_ w1847]
          tunnel: w1819 -> [_ w1846]
          tunnel: w1818 -> [_ w1845]
          tunnel: w1817 -> [_ w1844]
          tunnel: w1816 -> [w1832 w1843]
          tunnel: w1815 -> [w1831 w1842]
          tunnel: w1814 -> [_ w1841]
          tunnel: w1813 -> [_ w1840]
          tunnel: [w1831 w1839] -> w1812
          tunnel: [w1832 w1838] -> w1811
          tunnel: w1810 -> [w1830 w1837]
          tunnel: [w1830 w1836] -> w1809
          tunnel: w1808 -> [_ w1835]
          tunnel: w1804 -> [_ w1834]
          tunnel: w1796 -> [_ w1833]
          frame False {
          }
          frame True {
            n616 = for {
              N: w1835 -> [_]
              tunnel: [w1874] -> w1852
              tunnel: w1847 -> [w1869]
              tunnel: w1846 -> [w1868]
              tunnel: w1845 -> [w1867]
              tunnel: w1844 -> [w1866]
              tunnel: w1841 -> [w1863]
              tunnel: w1840 -> [w1862]
              shift-right: [w1872] -> w1850
              shift-left: w1851 -> [w1873]
              shift-right: [w1870] -> w1848
              shift-left: w1849 -> [w1871]
              shift-right: [w1861] -> w1838
              shift-left: w1843 -> [w1865]
              shift-right: [w1853] -> w1839
              shift-left: w1842 -> [w1864]
              shift-right: [w1859] -> w1836
              shift-left: w1837 -> [w1860]
              tunnel: w1834 -> [w1857]
              tunnel: w1833 -> [w1855]
              i -> [w1858]
              n617 = Add(x=w1857, y=w1858) -> (x+y=w1856:u32)
              n618 = local read "Net Rp"() -> (w1854:bool)
              n619 = stacked-sequence {
                seq-local: [_ _ _ _ _ _ w2404 _] -> [_ _ _ _ _ _ _ w2427]
                seq-local: [_ _ w1985 _ _ _ _ _] -> [_ _ _ w2119 _ _ _ _]
                seq-local: [_ w1922 _ _ _ _ _ _] -> [_ _ w1986 _ _ _ _ _]
                seq-local: [_ _ w1984 _ _ _ _ _] -> [_ _ _ _ _ w2325 _ _]
                seq-local: [_ _ _ w2118 _ _ _ _] -> [_ _ _ _ w2190 _ _ _]
                seq-local: [_ _ _ _ w2191 _ _ _] -> [_ _ _ _ _ w2323 _ _]
                seq-local: [_ _ _ _ w2189 _ _ _] -> [_ _ _ _ _ w2324 _ _]
                seq-local: [_ _ _ _ _ w2322 _ _] -> [_ _ _ _ _ _ w2402 _]
                tunnel: [_ _ _ _ _ _ _ w2426] -> w1874
                tunnel: w1873 -> [_ w1918 _ _ _ _ _ _]
                tunnel: [_ _ _ _ _ _ _ w2425] -> w1872
                tunnel: w1871 -> [_ w1931 _ w2136 _ _ w2405 _]
                tunnel: [_ w1929 _ _ _ _ _ _] -> w1870
                tunnel: w1869 -> [_ _ w1998 _ w2201 w2333 _ w2435]
                tunnel: w1868 -> [_ _ w1997 _ w2200 w2332 _ w2434]
                tunnel: w1867 -> [_ _ w1996 _ w2199 w2331 _ w2433]
                tunnel: w1866 -> [_ _ w1995 _ w2198 w2330 _ w2432]
                tunnel: w1865 -> [_ _ w1994 _ w2197 w2329 _ w2431]
                tunnel: w1864 -> [_ _ w1993 _ w2196 _ _ _]
                tunnel: w1863 -> [_ _ w1992 _ w2195 _ _ w2430]
                tunnel: w1860 -> [_ _ w1991 _ w2194 w2328 _ w2429]
                tunnel: w1862 -> [_ _ w1990 _ w2193 w2327 _ w2428]
                tunnel: [_ _ w1988 _ _ _ _ _] -> w1861
                tunnel: [_ _ w1987 _ _ _ _ _] -> w1859
                tunnel: w1856 -> [w1876 w1915 _ w2123 _ _ _ _]
                tunnel: w1855 -> [_ w1914 _ w2120 _ _ _ _]
                tunnel: w1854 -> [_ _ _ _ _ _ w2403 w2424]
                tunnel: [_ _ _ _ _ w2321 _ _] -> w1853
                frame #0 {
                  # "Create output folder path"
                  n620 = Get Date/Time In Seconds() -> (seconds since 1Jan1904=w1895:timestamp)
                  n621 = local read "Folder Name"() -> (w1887:string)
                  n622 = Number To Decimal String(number=w1876) -> (decimal integer string=w1877:string)  [unwired: 1 in]
                  n623 = Format Date/Time String(time format string (%c)="%Y%m%d", seconds (now)=w1895) -> (date/time string=w1894:string)  [unwired: 1 in]
                  n624 = local read "Main Path"() -> (w1888:path)
                  n625 = local read "Subfolder"() -> (w1886:string)
                  n626 = Concatenate Strings(w1894, "_", w1887) -> (w1893:string)
                  n627 = Build Path(base path=w1888, name or relative path=w1893) -> (appended path=w1891:path)
                  n628 = call <vilib>:"Check if File or Folder Exists.vi"("path"=w1891) -> ("error out"=w1884:errorcluster, "file or folder exists?"=w1897:bool)  [unwired: 8 in, 1 out]
                  n629 = Concatenate Strings("A_", w1877) -> (w1875:string)
                  n630 = Build Path(base path=w1891, name or relative path=w1886) -> (appended path=w1882:path)
                  n631 = Build Path(base path=w1882, name or relative path=w1875) -> (appended path=w1879:path)
                  n632 = local write "Current status"(w1875) -> ()
                  n633 = case shown="False" w1897 {
                    tunnel: w1891 -> [w1911 _]
                    tunnel: w1884 -> [w1910 w1912]
                    tunnel: [w1909 w1912] -> w1883
                    frame False {
                      n634 = Create Folder(path (use dialog)=w1911, error in=w1910) -> (error out=w1909:errorcluster)  [unwired: 1 in, 2 out]
                    }
                    frame True {
                    }
                  }
                  n635 = call <vilib>:"Check if File or Folder Exists.vi"("error in (no error)"=w1883, "path"=w1882) -> ("error out"=w1881:errorcluster, "file or folder exists?"=w1885:bool)  [unwired: 7 in, 1 out]
                  n636 = case shown="True" w1885 {
                    tunnel: w1882 -> [w1900 _]
                    tunnel: w1881 -> [w1899 w1901]
                    tunnel: [w1898 w1901] -> w1880
                    frame False {
                      n637 = Create Folder(path (use dialog)=w1900, error in=w1899) -> (error out=w1898:errorcluster)  [unwired: 1 in, 2 out]
                    }
                    frame True {
                    }
                  }
                  n638 = call <vilib>:"Check if File or Folder Exists.vi"("error in (no error)"=w1880, "path"=w1879) -> ("error out"=w1892:errorcluster, "file or folder exists?"=w1896:bool)  [unwired: 7 in, 1 out]
                  n639 = case shown="False" w1896 {
                    tunnel: w1879 -> [w1903 w1907]
                    tunnel: w1892 -> [w1902 w1908]
                    frame False {
                      n640 = Create Folder(path (use dialog)=w1903, error in=w1902) -> ()  [unwired: 1 in, 3 out]
                    }
                    frame True {
                      n641 = Delete(path (use dialog)=w1907, entire hierarchy (F)=TRUE, error in=w1908) -> (deleted path=w1905:path, error out=w1904:errorcluster)  [unwired: 2 in, 1 out]
                      n642 = Create Folder(path (use dialog)=w1905, error in=w1904) -> ()  [unwired: 1 in, 3 out]
                    }
                  }
                  n643 = local write "Output path"(w1879) -> ()
                }
                frame #1 {
                  # "Delay for DM response"
                  # "Apply positive command to DM"
                  n644 = local read "Initial offset"() -> (w1930:bool)
                  n645 = case shown="True" w1930 {
                    tunnel: [w1978 w1983] -> w1923
                    frame False {
                      n646 = Initialize Array(0.0, 52) -> (w1978:dbl[])
                    }
                    frame True {
                      n647 = local read "Offset command file"() -> (w1982:path)
                      n648 = call-poly <vilib>:"Read From Spreadsheet File.vi"("format (%.3f)"="%.8f", "file path (dialog if empty)"=w1982) -> ("first row"=w1983:dbl[])  [unwired: 5 in, 4 out]
                    }
                  }
                  n649 = local read "File Base Name"() -> (w1924:string)
                  n650 = local read "Output path"() -> (w1927:path)
                  n651 = Initialize Array(0.0, 52) -> (w1916:dbl[])
                  n652 = local read "Save File"() -> (w1928:bool)
                  n653 = local write "Initial Positions"(w1923) -> ()
                  n654 = Decrement(x=w1915) -> (x-1=w1917:u32)
                  n655 = Replace Array Subset(array=w1916, new element=w1914, index=w1917) -> (w1913:dbl[])
                  n656 = Add(x=w1913, y=w1923) -> (x+y=w1925:dbl[])
                  n657 = call <userlib>:"LVClass_WavefrontCorrector Move to Absolute Position.vi"("WavefrontCorrector in"=w1931, "Absolute Positions"=w1925, "error in (no error)"=w1918) -> ("WavefrontCorrector out"=w1932:refnum<class "WavefrontCorrector.lvclass">, "error out"=w1933:errorcluster)  [unwired: 11 in]
                  n658 = call <userlib>:"LVClass_WavefrontCorrector Get Current Position.vi"("WavefrontCorrector in"=w1932, "error in (no error)"=w1933) -> ("WavefrontCorrector out"=w1929:refnum<class "WavefrontCorrector.lvclass">, "Wavefront Corrector Position"=w1926:T14, "error out"=w1921:errorcluster)  [unwired: 11 in]
                  n659 = case shown="True" w1928 {
                    tunnel: w1927 -> [_ w1941]
                    tunnel: w1924 -> [_ w1940]
                    tunnel: w1923 -> [_ w1939]
                    tunnel: w1913 -> [_ w1938]
                    tunnel: w1925 -> [_ w1937]
                    tunnel: w1926 -> [_ w1936]
                    frame False {
                    }
                    frame True {
                      n660 = stacked-sequence {
                        tunnel: w1941 -> [w1946 w1955 w1964 w1973]
                        tunnel: w1940 -> [w1944 w1953 w1962 w1971]
                        tunnel: w1939 -> [w1942 _ _ _]
                        tunnel: w1938 -> [_ w1951 _ _]
                        tunnel: w1937 -> [_ _ w1960 _]
                        tunnel: w1936 -> [_ _ _ w1969]
                        frame #0 {
                          n661 = Concatenate Strings(w1944, "_cmdOffset_1", ".dat") -> (w1947:string)
                          n662 = Build Path(base path=w1946, name or relative path=w1947) -> (appended path=w1948:path)
                          n663 = Array To Spreadsheet String(array=w1942, 3:"%f") -> (spreadsheet string=w1949:string)  [unwired: 1 in]
                          n664 = Write to Text File(file (use dialog)=w1948, text=w1949) -> ()  [unwired: 2 in, 3 out]
                        }
                        frame #1 {
                          n665 = Concatenate Strings(w1953, "_cmdAdd_1", ".dat") -> (w1956:string)
                          n666 = Build Path(base path=w1955, name or relative path=w1956) -> (appended path=w1957:path)
                          n667 = Array To Spreadsheet String(array=w1951, 3:"%f") -> (spreadsheet string=w1958:string)  [unwired: 1 in]
                          n668 = Write to Text File(file (use dialog)=w1957, text=w1958) -> ()  [unwired: 2 in, 3 out]
                        }
                        frame #2 {
                          n669 = Concatenate Strings(w1962, "_cmdFinal_1", ".dat") -> (w1965:string)
                          n670 = Build Path(base path=w1964, name or relative path=w1965) -> (appended path=w1966:path)
                          n671 = Array To Spreadsheet String(array=w1960, 3:"%f") -> (spreadsheet string=w1967:string)  [unwired: 1 in]
                          n672 = Write to Text File(file (use dialog)=w1966, text=w1967) -> ()  [unwired: 2 in, 3 out]
                        }
                        frame #3 {
                          n673 = Concatenate Strings(w1971, "_cmdFinalMirror_1", ".dat") -> (w1974:string)
                          n674 = Build Path(base path=w1973, name or relative path=w1974) -> (appended path=w1975:path)
                          n675 = Array To Spreadsheet String(array=w1969, 3:"%f") -> (spreadsheet string=w1976:string)  [unwired: 1 in]
                          n676 = Write to Text File(file (use dialog)=w1975, text=w1976) -> ()  [unwired: 2 in, 3 out]
                        }
                      }
                    }
                  }
                  n677 = local write "Final Positions"(w1925) -> ()
                  n678 = local write "DM Actuator Values"(w1926) -> ()
                  n679 = flat-sequence {
                    tunnel: [w1934] -> w1922
                    tunnel: w1921 -> [w1934]
                    frame #0 {
                      n680 = Wait (ms)(milliseconds to wait=u32 50) -> ()  [unwired: 1 out]
                    }
                  }
                }
                frame #2 {
                  n681 = local read "HASO ready"() -> (w1989:bool)
                  n682 = case shown="True" w1989 {
                    tunnel: w1998 -> [_ w2024]
                    tunnel: w1996 -> [_ w2023]
                    tunnel: w1995 -> [_ w2022]
                    tunnel: [w1999 w2021] -> w1985
                    tunnel: w1997 -> [_ w2020]
                    tunnel: w1990 -> [_ w2007]
                    tunnel: w1986 -> [w1999 w2006]
                    tunnel: w1993 -> [w2002 w2019]
                    tunnel: w1992 -> [w2001 w2018]
                    tunnel: [w2002 w2017] -> w1984
                    tunnel: [w2001 w2016] -> _
                    tunnel: w1994 -> [w2003 w2015]
                    tunnel: w1991 -> [w2000 w2014]
                    tunnel: [w2003 w2013] -> w1988
                    tunnel: [w2000 w2012] -> w1987
                    frame False {
                    }
                    frame True {
                      n683 = property on="nb_images (set)" class="DigNum (strict)"() -> ("Value"=w2025:u32)  [unwired: 2 in, 2 out]
                      n684 = case shown="2, Default" w2025 {
                        tunnel: [w2115 w2117] -> w2005
                        tunnel: w2020 -> [w2114 _]
                        tunnel: w2024 -> [w2115 _]
                        tunnel: [w2114 w2116] -> w2004
                        tunnel: w2023 -> [_ w2117]
                        tunnel: w2022 -> [_ w2116]
                        frame 2, Default {
                        }
                        frame 1 {
                        }
                      }
                      n685 = stacked-sequence {
                        tunnel: w2005 -> [_ w2043]
                        tunnel: w2004 -> [_ w2042]
                        tunnel: [_ w2041] -> w2008
                        tunnel: [_ w2039] -> w2009
                        tunnel: [_ w2038] -> _
                        tunnel: w2007 -> [_ w2035]
                        tunnel: w2006 -> [_ w2034]
                        frame #0 {
                          # "Delay until MD gets stable"
                          n686 = local read "exposure_duration_s (set)"() -> (w2026:dbl)
                          n687 = local read "nb_images (set)"() -> (w2027:u32)
                          n688 = Multiply(x=w2026, y=w2027) -> (x*y=w2028:dbl)
                          n689 = Add(x=w2028, y=3.0) -> (x+y=w2029:dbl)
                          n690 = Multiply(x=w2029, y=1000.0) -> (x*y=w2033:dbl)
                          n691 = To Unsigned Long Integer(number=w2033) -> (unsigned 32bit integer=w2032:u32)
                          n692 = Wait (ms)(milliseconds to wait=w2032) -> ()  [unwired: 1 out]
                        }
                        frame #1 {
                          n693 = while {
                            tunnel: w2035 -> [w2048]
                            tunnel: [w2047] -> w2037
                            tunnel: w2034 -> [w2045]
                            tunnel: [w2044] -> w2036
                            stop <- w2046 stop-if-true
                            n694 = call <userlib>:"LVClass_Camera asynchroneImageReady.vi"("Camera in"=w2048, "error in (no error)"=w2045) -> ("Camera out"=w2047:refnum<class "Camera.lvclass">, "ready"=w2046:bool, "error out"=w2044:errorcluster)  [unwired: 11 in]
                          }
                          n695 = call <userlib>:"LVClass_Camera get image.vi"("Camera in"=w2037, "Image"=w2043, "Image RAW"=w2042, "remove_background"=FALSE, "error in (no error)"=w2036) -> ("Camera out"=w2038:refnum<class "Camera.lvclass">, "Image (dup)"=w2041:refnum<class "Image.lvclass">, "error out"=w2039:errorcluster)  [unwired: 7 in, 1 out]
                        }
                      }
                      n696 = case shown="No Error" w2009 {
                        selector: w2009 -> [w2111 w2112]
                        tunnel: w2008 -> [w2105 w2113]
                        tunnel: [w2108 w2113] -> w2011
                        tunnel: [w2107 w2112] -> w2010
                        frame No Error {
                          # "get image"
                          n697 = call <userlib>:"LVClass_Image get image data.vi"("Image in"=w2105, "error in (no error)"=w2111) -> ("Image out"=w2110:refnum<class "Image.lvclass">, "Image data out"=w2106:u32[][], "error out"=w2109:errorcluster)  [unwired: 11 in]
                          n698 = call <userlib>:"LVClass_Image get image information.vi"("Image in"=w2110, "error in (no error)"=w2109) -> ("Image out"=w2108:refnum<class "Image.lvclass">, "error out"=w2107:errorcluster)  [unwired: 11 in, 1 out]
                          n699 = local write "HASO intensity"(w2106) -> ()
                        }
                        frame Error {
                        }
                      }
                      n700 = case shown="No Error" w2010 {
                        selector: w2010 -> [w2072 w2104]
                        tunnel: [w2078 w2104] -> w2021
                        tunnel: w2011 -> [w2071 _]
                        tunnel: [w2076 w2100] -> w2012
                        tunnel: [w2075 w2103] -> w2013
                        tunnel: w2019 -> [w2068 w2102]
                        tunnel: w2018 -> [w2067 w2101]
                        tunnel: [w2055 w2102] -> w2017
                        tunnel: [w2066 w2101] -> w2016
                        tunnel: w2015 -> [w2064 w2103]
                        tunnel: w2014 -> [w2062 w2100]
                        frame No Error {
                          # "phaseout"
                          n701 = local read "File Base Name"() -> (w2053:string)
                          n702 = local read "Save File"() -> (w2054:bool)
                          n703 = local read "Output path"() -> (w2052:path)
                          n704 = call "image2slopes.vi"("error in (no error)"=w2072, "Image in"=w2071, "HasoEngine in"=w2067, "HasoSlopes in"=w2068) -> ("error out"=w2065:errorcluster, "HasoEngine out"=w2066:refnum<class "HasoEngine.lvclass">, "HasoSlopes out"=w2049:refnum<class "HasoSlopes.lvclass">)  [unwired: 4 in, 1 out]
                          n705 = local read "Filter"() -> (w2061:u8[])
                          n706 = call "slopes2phase.vi"("TypePhase"=WavefrontReconstructionMode."Modal_Zernike", "Number of coefficients"=u8 32, "error in (no error)"=w2065, "Filter"=w2061, "HasoSlopes in"=w2049, "Phase in"=w2064) -> ("error out"=w2057:errorcluster, "HasoSlopes out"=w2058:refnum<class "HasoSlopes.lvclass">, "Phase out"=w2063:refnum<class "Phase.lvclass">)  [unwired: 3 in]
                          n707 = local read "idxType"() -> (w2051:enum16{"Wyant", "ANSI"})
                          n708 = call "slopes2zern.vi"("HasoSlopes in"=w2058, "error in (no error)"=w2057, "idxType"=w2051) -> ("HasoSlopes out"=w2055:refnum<class "HasoSlopes.lvclass">, "Zernike Coefficients"=w2050:dbl[], "error out"=w2056:errorcluster)  [unwired: 3 in, 2 out]
                          n709 = call <userlib>:"LVClass_Pupil ctor from HasoSlopes.vi"("Pupil in"=w2062, "HasoSlopes.lvclass"=w2049, "error in (no error)"=w2056) -> ("Pupil out"=w2073:refnum<class "Pupil.lvclass">, "error out"=w2074:errorcluster)  [unwired: 11 in]
                          n710 = case shown="True" w2054 {
                            tunnel: w2053 -> [_ w2083]
                            tunnel: w2052 -> [_ w2082]
                            tunnel: w2050 -> [_ w2081]
                            tunnel: w2049 -> [_ w2080]
                            frame False {
                            }
                            frame True {
                              n711 = stacked-sequence {
                                tunnel: w2083 -> [w2087 w2093]
                                tunnel: w2082 -> [w2086 w2092]
                                tunnel: w2081 -> [_ w2091]
                                tunnel: w2080 -> [w2084 _]
                                frame #0 {
                                n712 = Concatenate Strings(w2087, "_slopesMeas_1", ".has") -> (w2090:string)
                                n713 = Build Path(base path=w2086, name or relative path=w2090) -> (appended path=w2085:path)
                                n714 = call <userlib>:"LVClass_HasoSlopes Save.vi"("HasoSlopes in"=w2084, "path"=w2085) -> ()  [unwired: 12 in, 2 out]
                                }
                                frame #1 {
                                n715 = Concatenate Strings(w2093, "_zernCoefMeas_1", ".txt") -> (w2096:string)
                                n716 = Build Path(base path=w2092, name or relative path=w2096) -> (appended path=w2097:path)
                                n717 = Array To Spreadsheet String(array=w2091, 3:"%f") -> (spreadsheet string=w2098:string)  [unwired: 1 in]
                                n718 = Write to Text File(file (use dialog)=w2097, text=w2098) -> ()  [unwired: 2 in, 3 out]
                                }
                              }
                            }
                          }
                          n719 = call <userlib>:"LVClasse_Phase GetStatisticDatas.vi"("Phase in"=w2063, "error in (no error)"=w2074) -> ("Phase out"=w2079:refnum<class "Phase.lvclass">, "StatisticsData"=w2059:T2, "error out"=w2077:errorcluster)  [unwired: 11 in]
                          n720 = local write "Phase statistics"(w2059) -> ()
                          n721 = call <userlib>:"LVClasse_Phase Get Data.vi"("Phase in"=w2079, "Pupil"=w2073, "error in (no error)"=w2077) -> ("Phase out"=w2075:refnum<class "Phase.lvclass">, "data"=w2060:sgl[][], "Pupil (dup)"=w2076:refnum<class "Pupil.lvclass">, "error out"=w2078:errorcluster)  [unwired: 9 in]
                          n722 = local write "Zernike Measured"(w2050) -> ()
                          n723 = local write "Phase values"(w2060) -> ()
                        }
                        frame Error {
                        }
                      }
                    }
                  }
                }
                frame #3 {
                  # "Delay for DM response"
                  # "Apply negtive command to DM"
                  n724 = local read "Initial offset"() -> (w2135:bool)
                  n725 = case shown="True" w2135 {
                    tunnel: [w2183 w2188] -> w2129
                    frame False {
                      n726 = Initialize Array(0.0, 52) -> (w2183:dbl[])
                    }
                    frame True {
                      n727 = local read "Offset command file"() -> (w2187:path)
                      n728 = call-poly <vilib>:"Read From Spreadsheet File.vi"("format (%.3f)"="%.8f", "file path (dialog if empty)"=w2187) -> ("first row"=w2188:dbl[])  [unwired: 5 in, 4 out]
                    }
                  }
                  n729 = local read "File Base Name"() -> (w2130:string)
                  n730 = local read "Output path"() -> (w2133:path)
                  n731 = Initialize Array(0.0, 52) -> (w2124:dbl[])
                  n732 = local read "Save File"() -> (w2134:bool)
                  n733 = local write "Initial Positions"(w2129) -> ()
                  n734 = Negate(x=w2120) -> (-x=w2121:dbl)
                  n735 = Decrement(x=w2123) -> (x-1=w2125:u32)
                  n736 = Replace Array Subset(array=w2124, new element=w2121, index=w2125) -> (w2122:dbl[])
                  n737 = Add(x=w2122, y=w2129) -> (x+y=w2131:dbl[])
                  n738 = call <userlib>:"LVClass_WavefrontCorrector Move to Absolute Position.vi"("WavefrontCorrector in"=w2136, "Absolute Positions"=w2131, "error in (no error)"=w2119) -> ("WavefrontCorrector out"=w2137:refnum<class "WavefrontCorrector.lvclass">, "error out"=w2138:errorcluster)  [unwired: 11 in]
                  n739 = call <userlib>:"LVClass_WavefrontCorrector Get Current Position.vi"("WavefrontCorrector in"=w2137, "error in (no error)"=w2138) -> ("Wavefront Corrector Position"=w2132:T14, "error out"=w2128:errorcluster)  [unwired: 11 in, 1 out]
                  n740 = case shown="True" w2134 {
                    tunnel: w2133 -> [_ w2146]
                    tunnel: w2130 -> [_ w2145]
                    tunnel: w2129 -> [_ w2144]
                    tunnel: w2122 -> [_ w2143]
                    tunnel: w2131 -> [_ w2142]
                    tunnel: w2132 -> [_ w2141]
                    frame False {
                    }
                    frame True {
                      n741 = stacked-sequence {
                        tunnel: w2146 -> [w2151 w2160 w2169 w2178]
                        tunnel: w2145 -> [w2149 w2158 w2167 w2176]
                        tunnel: w2144 -> [w2147 _ _ _]
                        tunnel: w2143 -> [_ w2156 _ _]
                        tunnel: w2142 -> [_ _ w2165 _]
                        tunnel: w2141 -> [_ _ _ w2174]
                        frame #0 {
                          n742 = Concatenate Strings(w2149, "_cmdOffset_-1", ".dat") -> (w2152:string)
                          n743 = Build Path(base path=w2151, name or relative path=w2152) -> (appended path=w2153:path)
                          n744 = Array To Spreadsheet String(array=w2147, 3:"%f") -> (spreadsheet string=w2154:string)  [unwired: 1 in]
                          n745 = Write to Text File(file (use dialog)=w2153, text=w2154) -> ()  [unwired: 2 in, 3 out]
                        }
                        frame #1 {
                          n746 = Concatenate Strings(w2158, "_cmdAdd_-1", ".dat") -> (w2161:string)
                          n747 = Build Path(base path=w2160, name or relative path=w2161) -> (appended path=w2162:path)
                          n748 = Array To Spreadsheet String(array=w2156, 3:"%f") -> (spreadsheet string=w2163:string)  [unwired: 1 in]
                          n749 = Write to Text File(file (use dialog)=w2162, text=w2163) -> ()  [unwired: 2 in, 3 out]
                        }
                        frame #2 {
                          n750 = Concatenate Strings(w2167, "_cmdFinal_-1", ".dat") -> (w2170:string)
                          n751 = Build Path(base path=w2169, name or relative path=w2170) -> (appended path=w2171:path)
                          n752 = Array To Spreadsheet String(array=w2165, 3:"%f") -> (spreadsheet string=w2172:string)  [unwired: 1 in]
                          n753 = Write to Text File(file (use dialog)=w2171, text=w2172) -> ()  [unwired: 2 in, 3 out]
                        }
                        frame #3 {
                          n754 = Concatenate Strings(w2176, "_cmdFinalMirror_-1", ".dat") -> (w2179:string)
                          n755 = Build Path(base path=w2178, name or relative path=w2179) -> (appended path=w2180:path)
                          n756 = Array To Spreadsheet String(array=w2174, 3:"%f") -> (spreadsheet string=w2181:string)  [unwired: 1 in]
                          n757 = Write to Text File(file (use dialog)=w2180, text=w2181) -> ()  [unwired: 2 in, 3 out]
                        }
                      }
                    }
                  }
                  n758 = local write "Final Positions"(w2131) -> ()
                  n759 = local write "DM Actuator Values"(w2132) -> ()
                  n760 = flat-sequence {
                    tunnel: [w2139] -> w2118
                    tunnel: w2128 -> [w2139]
                    frame #0 {
                      n761 = Wait (ms)(milliseconds to wait=u32 50) -> ()  [unwired: 1 out]
                    }
                  }
                }
                frame #4 {
                  n762 = local read "HASO ready"() -> (w2192:bool)
                  n763 = case shown="True" w2192 {
                    tunnel: w2201 -> [_ w2227]
                    tunnel: w2199 -> [_ w2226]
                    tunnel: w2198 -> [_ w2225]
                    tunnel: [w2202 w2224] -> w2191
                    tunnel: w2200 -> [_ w2223]
                    tunnel: w2193 -> [_ w2211]
                    tunnel: w2190 -> [w2202 w2210]
                    tunnel: w2196 -> [w2205 _]
                    tunnel: w2195 -> [w2204 w2222]
                    tunnel: [w2205 w2221] -> w2189
                    tunnel: [w2204 w2220] -> _
                    tunnel: w2197 -> [w2206 w2219]
                    tunnel: w2194 -> [w2203 w2218]
                    tunnel: [w2206 w2217] -> _
                    tunnel: [w2203 w2216] -> _
                    frame False {
                    }
                    frame True {
                      n764 = property on="nb_images (set)" class="DigNum (strict)"() -> ("Value"=w2228:u32)  [unwired: 2 in, 2 out]
                      n765 = case shown="2, Default" w2228 {
                        tunnel: [w2318 w2320] -> w2209
                        tunnel: w2223 -> [w2317 _]
                        tunnel: w2227 -> [w2318 _]
                        tunnel: [w2317 w2319] -> w2208
                        tunnel: w2226 -> [_ w2320]
                        tunnel: w2225 -> [_ w2319]
                        frame 2, Default {
                        }
                        frame 1 {
                        }
                      }
                      n766 = stacked-sequence {
                        tunnel: w2209 -> [_ w2246]
                        tunnel: w2208 -> [_ w2245]
                        tunnel: [_ w2244] -> w2212
                        tunnel: [_ w2242] -> w2213
                        tunnel: [_ w2241] -> _
                        tunnel: w2211 -> [_ w2238]
                        tunnel: w2210 -> [_ w2237]
                        frame #0 {
                          # "Delay until MD gets stable"
                          n767 = local read "exposure_duration_s (set)"() -> (w2229:dbl)
                          n768 = local read "nb_images (set)"() -> (w2230:u32)
                          n769 = Multiply(x=w2229, y=w2230) -> (x*y=w2231:dbl)
                          n770 = Add(x=w2231, y=3.0) -> (x+y=w2232:dbl)
                          n771 = Multiply(x=w2232, y=1000.0) -> (x*y=w2236:dbl)
                          n772 = To Unsigned Long Integer(number=w2236) -> (unsigned 32bit integer=w2235:u32)
                          n773 = Wait (ms)(milliseconds to wait=w2235) -> ()  [unwired: 1 out]
                        }
                        frame #1 {
                          n774 = while {
                            tunnel: w2238 -> [w2251]
                            tunnel: [w2250] -> w2240
                            tunnel: w2237 -> [w2248]
                            tunnel: [w2247] -> w2239
                            stop <- w2249 stop-if-true
                            n775 = call <userlib>:"LVClass_Camera asynchroneImageReady.vi"("Camera in"=w2251, "error in (no error)"=w2248) -> ("Camera out"=w2250:refnum<class "Camera.lvclass">, "ready"=w2249:bool, "error out"=w2247:errorcluster)  [unwired: 11 in]
                          }
                          n776 = call <userlib>:"LVClass_Camera get image.vi"("Camera in"=w2240, "Image"=w2246, "Image RAW"=w2245, "remove_background"=FALSE, "error in (no error)"=w2239) -> ("Camera out"=w2241:refnum<class "Camera.lvclass">, "Image (dup)"=w2244:refnum<class "Image.lvclass">, "error out"=w2242:errorcluster)  [unwired: 7 in, 1 out]
                        }
                      }
                      n777 = case shown="No Error" w2213 {
                        selector: w2213 -> [w2314 w2315]
                        tunnel: w2212 -> [w2308 w2316]
                        tunnel: [w2311 w2316] -> w2215
                        tunnel: [w2310 w2315] -> w2214
                        frame No Error {
                          # "get image"
                          n778 = call <userlib>:"LVClass_Image get image data.vi"("Image in"=w2308, "error in (no error)"=w2314) -> ("Image out"=w2313:refnum<class "Image.lvclass">, "Image data out"=w2309:u32[][], "error out"=w2312:errorcluster)  [unwired: 11 in]
                          n779 = call <userlib>:"LVClass_Image get image information.vi"("Image in"=w2313, "error in (no error)"=w2312) -> ("Image out"=w2311:refnum<class "Image.lvclass">, "error out"=w2310:errorcluster)  [unwired: 11 in, 1 out]
                          n780 = local write "HASO intensity"(w2309) -> ()
                        }
                        frame Error {
                        }
                      }
                      n781 = case shown="No Error" w2214 {
                        selector: w2214 -> [w2275 w2307]
                        tunnel: [w2281 w2307] -> w2224
                        tunnel: w2215 -> [w2274 _]
                        tunnel: [w2279 w2303] -> w2216
                        tunnel: [w2278 w2306] -> w2217
                        tunnel: refnum<class "HasoSlopes.lvclass"> refnum ("HasoSlopes in") -> [w2271 w2305]
                        tunnel: w2222 -> [w2270 w2304]
                        tunnel: [w2258 w2305] -> w2221
                        tunnel: [w2269 w2304] -> w2220
                        tunnel: w2219 -> [w2267 w2306]
                        tunnel: w2218 -> [w2265 w2303]
                        frame No Error {
                          # "phaseout"
                          n782 = local read "File Base Name"() -> (w2256:string)
                          n783 = local read "Save File"() -> (w2257:bool)
                          n784 = local read "Output path"() -> (w2255:path)
                          n785 = call "image2slopes.vi"("error in (no error)"=w2275, "Image in"=w2274, "HasoEngine in"=w2270, "HasoSlopes in"=w2271) -> ("error out"=w2268:errorcluster, "HasoEngine out"=w2269:refnum<class "HasoEngine.lvclass">, "HasoSlopes out"=w2252:refnum<class "HasoSlopes.lvclass">)  [unwired: 4 in, 1 out]
                          n786 = local read "Filter"() -> (w2264:u8[])
                          n787 = call "slopes2phase.vi"("TypePhase"=WavefrontReconstructionMode."Modal_Zernike", "Number of coefficients"=u8 32, "error in (no error)"=w2268, "Filter"=w2264, "HasoSlopes in"=w2252, "Phase in"=w2267) -> ("error out"=w2260:errorcluster, "HasoSlopes out"=w2261:refnum<class "HasoSlopes.lvclass">, "Phase out"=w2266:refnum<class "Phase.lvclass">)  [unwired: 3 in]
                          n788 = local read "idxType"() -> (w2254:enum16{"Wyant", "ANSI"})
                          n789 = call "slopes2zern.vi"("HasoSlopes in"=w2261, "error in (no error)"=w2260, "idxType"=w2254) -> ("HasoSlopes out"=w2258:refnum<class "HasoSlopes.lvclass">, "Zernike Coefficients"=w2253:dbl[], "error out"=w2259:errorcluster)  [unwired: 3 in, 2 out]
                          n790 = call <userlib>:"LVClass_Pupil ctor from HasoSlopes.vi"("Pupil in"=w2265, "HasoSlopes.lvclass"=w2252, "error in (no error)"=w2259) -> ("Pupil out"=w2276:refnum<class "Pupil.lvclass">, "error out"=w2277:errorcluster)  [unwired: 11 in]
                          n791 = case shown="True" w2257 {
                            tunnel: w2256 -> [_ w2286]
                            tunnel: w2255 -> [_ w2285]
                            tunnel: w2253 -> [_ w2284]
                            tunnel: w2252 -> [_ w2283]
                            frame False {
                            }
                            frame True {
                              n792 = stacked-sequence {
                                tunnel: w2286 -> [w2290 w2296]
                                tunnel: w2285 -> [w2289 w2295]
                                tunnel: w2284 -> [_ w2294]
                                tunnel: w2283 -> [w2287 _]
                                frame #0 {
                                n793 = Concatenate Strings(w2290, "_slopesMeas_-1", ".has") -> (w2293:string)
                                n794 = Build Path(base path=w2289, name or relative path=w2293) -> (appended path=w2288:path)
                                n795 = call <userlib>:"LVClass_HasoSlopes Save.vi"("HasoSlopes in"=w2287, "path"=w2288) -> ()  [unwired: 12 in, 2 out]
                                }
                                frame #1 {
                                n796 = Concatenate Strings(w2296, "_zernCoefMeas_-1", ".txt") -> (w2299:string)
                                n797 = Build Path(base path=w2295, name or relative path=w2299) -> (appended path=w2300:path)
                                n798 = Array To Spreadsheet String(array=w2294, 3:"%f") -> (spreadsheet string=w2301:string)  [unwired: 1 in]
                                n799 = Write to Text File(file (use dialog)=w2300, text=w2301) -> ()  [unwired: 2 in, 3 out]
                                }
                              }
                            }
                          }
                          n800 = call <userlib>:"LVClasse_Phase GetStatisticDatas.vi"("Phase in"=w2266, "error in (no error)"=w2277) -> ("Phase out"=w2282:refnum<class "Phase.lvclass">, "StatisticsData"=w2262:T2, "error out"=w2280:errorcluster)  [unwired: 11 in]
                          n801 = local write "Phase statistics"(w2262) -> ()
                          n802 = call <userlib>:"LVClasse_Phase Get Data.vi"("Phase in"=w2282, "Pupil"=w2276, "error in (no error)"=w2280) -> ("Phase out"=w2278:refnum<class "Phase.lvclass">, "data"=w2263:sgl[][], "Pupil (dup)"=w2279:refnum<class "Pupil.lvclass">, "error out"=w2281:errorcluster)  [unwired: 9 in]
                          n803 = local write "Zernike Measured"(w2253) -> ()
                          n804 = local write "Phase values"(w2263) -> ()
                        }
                        frame Error {
                        }
                      }
                    }
                  }
                }
                frame #5 {
                  n805 = local read "HASO ready"() -> (w2326:bool)
                  n806 = case shown="True" w2326 {
                    tunnel: w2333 -> [_ _]
                    tunnel: w2331 -> [_ _]
                    tunnel: w2330 -> [_ _]
                    tunnel: [w2335 w2347] -> w2322
                    tunnel: w2332 -> [_ _]
                    tunnel: w2327 -> [_ _]
                    tunnel: [w2334 w2342] -> w2321
                    tunnel: w2329 -> [w2337 w2346]
                    tunnel: w2328 -> [w2336 w2345]
                    tunnel: [w2337 w2344] -> _
                    tunnel: [w2336 w2343] -> _
                    tunnel: w2325 -> [w2334 w2340]
                    tunnel: w2324 -> [_ w2339]
                    tunnel: w2323 -> [w2335 w2338]
                    frame False {
                    }
                    frame True {
                      n807 = case shown="No Error" w2338 {
                        selector: w2338 -> [w2349 w2401]
                        tunnel: [w2375 w2401] -> w2347
                        tunnel: [w2373 w2399] -> w2343
                        tunnel: [w2372 w2400] -> w2344
                        tunnel: w2346 -> [w2367 w2400]
                        tunnel: w2345 -> [w2365 w2399]
                        tunnel: [w2351 w2397] -> w2342
                        tunnel: [w2348 w2398] -> w2341
                        tunnel: w2340 -> [w2350 w2397]
                        tunnel: w2339 -> [w2348 w2398]
                        frame No Error {
                          # "phaseout"
                          n808 = local read "File Base Name"() -> (w2357:string)
                          n809 = local read "Save File"() -> (w2358:bool)
                          n810 = local read "Output path"() -> (w2356:path)
                          n811 = local read "Filter"() -> (w2364:u8[])
                          n812 = call <userlib>:"LVClass_HasoSlopes Apply Substractor.vi"("HasoSlopes in"=w2350, "HasoSlopes to substract"=w2348, "error in (no error)"=w2349) -> ("HasoSlopes out"=w2353:refnum<class "HasoSlopes.lvclass">, "error out"=w2352:errorcluster)  [unwired: 11 in]
                          n813 = call "slopes2phase.vi"("TypePhase"=WavefrontReconstructionMode."Modal_Zernike", "Number of coefficients"=u8 32, "error in (no error)"=w2352, "Filter"=w2364, "HasoSlopes in"=w2353, "Phase in"=w2367) -> ("error out"=w2360:errorcluster, "HasoSlopes out"=w2361:refnum<class "HasoSlopes.lvclass">, "Phase out"=w2366:refnum<class "Phase.lvclass">)  [unwired: 3 in]
                          n814 = local read "idxType"() -> (w2355:enum16{"Wyant", "ANSI"})
                          n815 = call "slopes2zern.vi"("HasoSlopes in"=w2361, "error in (no error)"=w2360, "idxType"=w2355) -> ("HasoSlopes out"=w2351:refnum<class "HasoSlopes.lvclass">, "Zernike Coefficients"=w2354:dbl[], "error out"=w2359:errorcluster)  [unwired: 3 in, 2 out]
                          n816 = call <userlib>:"LVClass_Pupil ctor from HasoSlopes.vi"("Pupil in"=w2365, "HasoSlopes.lvclass"=w2353, "error in (no error)"=w2359) -> ("Pupil out"=w2370:refnum<class "Pupil.lvclass">, "error out"=w2371:errorcluster)  [unwired: 11 in]
                          n817 = case shown="True" w2358 {
                            tunnel: w2357 -> [_ w2380]
                            tunnel: w2356 -> [_ w2379]
                            tunnel: w2354 -> [_ w2378]
                            tunnel: w2353 -> [_ w2377]
                            frame False {
                            }
                            frame True {
                              n818 = stacked-sequence {
                                tunnel: w2380 -> [w2384 w2390]
                                tunnel: w2379 -> [w2383 w2389]
                                tunnel: w2378 -> [_ w2388]
                                tunnel: w2377 -> [w2381 _]
                                frame #0 {
                                n819 = Concatenate Strings(w2384, "_slopesNet", ".has") -> (w2387:string)
                                n820 = Build Path(base path=w2383, name or relative path=w2387) -> (appended path=w2382:path)
                                n821 = call <userlib>:"LVClass_HasoSlopes Save.vi"("HasoSlopes in"=w2381, "path"=w2382) -> ()  [unwired: 12 in, 2 out]
                                }
                                frame #1 {
                                n822 = Concatenate Strings(w2390, "_zernCoefNet", ".txt") -> (w2393:string)
                                n823 = Build Path(base path=w2389, name or relative path=w2393) -> (appended path=w2394:path)
                                n824 = Array To Spreadsheet String(array=w2388, 3:"%f") -> (spreadsheet string=w2395:string)  [unwired: 1 in]
                                n825 = Write to Text File(file (use dialog)=w2394, text=w2395) -> ()  [unwired: 2 in, 3 out]
                                }
                              }
                            }
                          }
                          n826 = call <userlib>:"LVClasse_Phase GetStatisticDatas.vi"("Phase in"=w2366, "error in (no error)"=w2371) -> ("Phase out"=w2376:refnum<class "Phase.lvclass">, "StatisticsData"=w2362:T2, "error out"=w2374:errorcluster)  [unwired: 11 in]
                          n827 = local write "Phase statistics"(w2362) -> ()
                          n828 = call <userlib>:"LVClasse_Phase Get Data.vi"("Phase in"=w2376, "Pupil"=w2370, "error in (no error)"=w2374) -> ("Phase out"=w2372:refnum<class "Phase.lvclass">, "data"=w2363:sgl[][], "Pupil (dup)"=w2373:refnum<class "Pupil.lvclass">, "error out"=w2375:errorcluster)  [unwired: 9 in]
                          n829 = local write "Zernike Measured"(w2354) -> ()
                          n830 = local write "Phase values"(w2363) -> ()
                        }
                        frame Error {
                        }
                      }
                      n831 = call <userlib>:"LVClass_HasoSlopes dtor.vi"("HasoSlopes in"=w2341) -> ()  [unwired: 13 in, 2 out]
                    }
                  }
                }
                frame #6 {
                  # "Apply offset to DM"
                  n832 = case shown="True" w2403 {
                    tunnel: w2405 -> [_ w2413]
                    tunnel: [w2406 w2408] -> w2404
                    tunnel: w2402 -> [w2406 w2409]
                    frame False {
                    }
                    frame True {
                      # "Delay for DM response"
                      n833 = local read "Initial offset"() -> (w2412:bool)
                      n834 = case shown="True" w2412 {
                        tunnel: [w2418 w2423] -> w2410
                        frame False {
                          n835 = Initialize Array(0.0, 52) -> (w2418:dbl[])
                        }
                        frame True {
                          n836 = local read "Offset command file"() -> (w2422:path)
                          n837 = call-poly <vilib>:"Read From Spreadsheet File.vi"("format (%.3f)"="%.8f", "file path (dialog if empty)"=w2422) -> ("first row"=w2423:dbl[])  [unwired: 5 in, 4 out]
                        }
                      }
                      n838 = local write "Initial Positions"(w2410) -> ()
                      n839 = call <userlib>:"LVClass_WavefrontCorrector Move to Absolute Position.vi"("WavefrontCorrector in"=w2413, "Absolute Positions"=w2410, "error in (no error)"=w2409) -> ("WavefrontCorrector out"=w2414:refnum<class "WavefrontCorrector.lvclass">, "error out"=w2415:errorcluster)  [unwired: 11 in]
                      n840 = call <userlib>:"LVClass_WavefrontCorrector Get Current Position.vi"("WavefrontCorrector in"=w2414, "error in (no error)"=w2415) -> ("Wavefront Corrector Position"=w2411:T14, "error out"=w2407:errorcluster)  [unwired: 11 in, 1 out]
                      n841 = local write "Initial Positions"(w2411) -> ()
                      n842 = flat-sequence {
                        tunnel: [w2416] -> w2408
                        tunnel: w2407 -> [w2416]
                        frame #0 {
                          n843 = Wait (ms)(milliseconds to wait=u32 50) -> ()  [unwired: 1 out]
                        }
                      }
                    }
                  }
                }
                frame #7 {
                  n844 = case shown="True" w2424 {
                    tunnel: w2435 -> [_ w2447]
                    tunnel: w2434 -> [_ w2446]
                    tunnel: w2433 -> [_ w2445]
                    tunnel: w2432 -> [_ w2444]
                    tunnel: w2431 -> [_ w2443]
                    tunnel: w2430 -> [_ w2442]
                    tunnel: w2429 -> [_ w2441]
                    tunnel: w2428 -> [_ w2440]
                    tunnel: w2427 -> [w2436 w2438]
                    tunnel: [w2436 w2437] -> w2425
                    frame False {
                    }
                    frame True {
                      n845 = local read "HASO ready"() -> (w2439:bool)
                      n846 = case shown="True" w2439 {
                        tunnel: w2447 -> [_ w2472]
                        tunnel: w2445 -> [_ w2471]
                        tunnel: w2444 -> [_ w2470]
                        tunnel: [w2448 w2469] -> w2437
                        tunnel: w2446 -> [_ w2468]
                        tunnel: w2440 -> [_ w2455]
                        tunnel: w2438 -> [w2448 w2454]
                        tunnel: w2442 -> [w2450 w2467]
                        tunnel: [w2450 w2466] -> _
                        tunnel: w2443 -> [w2451 w2465]
                        tunnel: w2441 -> [w2449 w2464]
                        tunnel: [w2451 w2463] -> _
                        tunnel: [w2449 w2462] -> _
                        frame False {
                        }
                        frame True {
                          n847 = property on="nb_images (set)" class="DigNum (strict)"() -> ("Value"=w2473:u32)  [unwired: 2 in, 2 out]
                          n848 = case shown="2, Default" w2473 {
                            tunnel: [w2562 w2564] -> w2457
                            tunnel: w2468 -> [w2561 _]
                            tunnel: w2472 -> [w2562 _]
                            tunnel: [w2561 w2563] -> w2456
                            tunnel: w2471 -> [_ w2564]
                            tunnel: w2470 -> [_ w2563]
                            frame 2, Default {
                            }
                            frame 1 {
                            }
                          }
                          n849 = stacked-sequence {
                            tunnel: w2457 -> [_ w2491]
                            tunnel: w2456 -> [_ w2490]
                            tunnel: [_ w2489] -> w2453
                            tunnel: [_ w2487] -> w2452
                            tunnel: [_ w2486] -> _
                            tunnel: w2455 -> [_ w2483]
                            tunnel: w2454 -> [_ w2482]
                            frame #0 {
                              # "Delay until MD gets stable"
                              n850 = local read "exposure_duration_s (set)"() -> (w2474:dbl)
                              n851 = local read "nb_images (set)"() -> (w2475:u32)
                              n852 = Multiply(x=w2474, y=w2475) -> (x*y=w2476:dbl)
                              n853 = Add(x=w2476, y=3.0) -> (x+y=w2477:dbl)
                              n854 = Multiply(x=w2477, y=1000.0) -> (x*y=w2481:dbl)
                              n855 = To Unsigned Long Integer(number=w2481) -> (unsigned 32bit integer=w2480:u32)
                              n856 = Wait (ms)(milliseconds to wait=w2480) -> ()  [unwired: 1 out]
                            }
                            frame #1 {
                              n857 = while {
                                tunnel: w2483 -> [w2496]
                                tunnel: [w2495] -> w2485
                                tunnel: w2482 -> [w2493]
                                tunnel: [w2492] -> w2484
                                stop <- w2494 stop-if-true
                                n858 = call <userlib>:"LVClass_Camera asynchroneImageReady.vi"("Camera in"=w2496, "error in (no error)"=w2493) -> ("Camera out"=w2495:refnum<class "Camera.lvclass">, "ready"=w2494:bool, "error out"=w2492:errorcluster)  [unwired: 11 in]
                              }
                              n859 = call <userlib>:"LVClass_Camera get image.vi"("Camera in"=w2485, "Image"=w2491, "Image RAW"=w2490, "remove_background"=FALSE, "error in (no error)"=w2484) -> ("Camera out"=w2486:refnum<class "Camera.lvclass">, "Image (dup)"=w2489:refnum<class "Image.lvclass">, "error out"=w2487:errorcluster)  [unwired: 7 in, 1 out]
                            }
                          }
                          n860 = case shown="No Error" w2452 {
                            selector: w2452 -> [w2558 w2559]
                            tunnel: w2453 -> [w2555 w2560]
                            tunnel: [w2554 w2560] -> w2461
                            tunnel: [w2553 w2559] -> w2460
                            frame No Error {
                              # "get image"
                              n861 = call <userlib>:"LVClass_Image get image data.vi"("Image in"=w2555, "error in (no error)"=w2558) -> ("Image out"=w2557:refnum<class "Image.lvclass">, "Image data out"=w2552:u32[][], "error out"=w2556:errorcluster)  [unwired: 11 in]
                              n862 = call <userlib>:"LVClass_Image get image information.vi"("Image in"=w2557, "error in (no error)"=w2556) -> ("Image out"=w2554:refnum<class "Image.lvclass">, "error out"=w2553:errorcluster)  [unwired: 11 in, 1 out]
                              n863 = local write "HASO intensity"(w2552) -> ()
                            }
                            frame Error {
                            }
                          }
                          n864 = case shown="No Error" w2460 {
                            selector: w2460 -> [w2519 w2551]
                            tunnel: [w2525 w2551] -> w2469
                            tunnel: w2461 -> [w2518 _]
                            tunnel: [w2523 w2548] -> w2462
                            tunnel: [w2522 w2550] -> w2463
                            tunnel: refnum<class "HasoSlopes.lvclass"> refnum ("HasoSlopes in") -> [w2515 w2547]
                            tunnel: w2467 -> [w2514 w2549]
                            tunnel: [w2513 w2549] -> w2466
                            tunnel: w2465 -> [w2512 w2550]
                            tunnel: w2464 -> [w2510 w2548]
                            tunnel: [w2497 w2547] -> w2458
                            frame No Error {
                              # "phaseout"
                              n865 = local read "File Base Name"() -> (w2502:string)
                              n866 = local read "Save File"() -> (w2503:bool)
                              n867 = local read "Output path"() -> (w2501:path)
                              n868 = call "image2slopes.vi"("error in (no error)"=w2519, "Image in"=w2518, "HasoEngine in"=w2514, "HasoSlopes in"=w2515) -> ("error out"=w2498:errorcluster, "HasoEngine out"=w2513:refnum<class "HasoEngine.lvclass">, "HasoSlopes out"=w2497:refnum<class "HasoSlopes.lvclass">)  [unwired: 4 in, 1 out]
                              n869 = local read "Filter"() -> (w2509:u8[])
                              n870 = call "slopes2phase.vi"("TypePhase"=WavefrontReconstructionMode."Modal_Zernike", "Number of coefficients"=u8 32, "error in (no error)"=w2498, "Filter"=w2509, "HasoSlopes in"=w2497, "Phase in"=w2512) -> ("error out"=w2505:errorcluster, "HasoSlopes out"=w2506:refnum<class "HasoSlopes.lvclass">, "Phase out"=w2511:refnum<class "Phase.lvclass">)  [unwired: 3 in]
                              n871 = local read "idxType"() -> (w2500:enum16{"Wyant", "ANSI"})
                              n872 = call "slopes2zern.vi"("HasoSlopes in"=w2506, "error in (no error)"=w2505, "idxType"=w2500) -> ("Zernike Coefficients"=w2499:dbl[], "error out"=w2504:errorcluster)  [unwired: 3 in, 3 out]
                              n873 = call <userlib>:"LVClass_Pupil ctor from HasoSlopes.vi"("Pupil in"=w2510, "HasoSlopes.lvclass"=w2497, "error in (no error)"=w2504) -> ("Pupil out"=w2520:refnum<class "Pupil.lvclass">, "error out"=w2521:errorcluster)  [unwired: 11 in]
                              n874 = case shown="True" w2503 {
                                tunnel: w2502 -> [_ w2530]
                                tunnel: w2501 -> [_ w2529]
                                tunnel: w2499 -> [_ w2528]
                                tunnel: w2497 -> [_ w2527]
                                frame False {
                                }
                                frame True {
                                n875 = stacked-sequence {
                                tunnel: w2530 -> [w2534 w2540]
                                tunnel: w2529 -> [w2533 w2539]
                                tunnel: w2528 -> [_ w2538]
                                tunnel: w2527 -> [w2531 _]
                                frame #0 {
                                n876 = Concatenate Strings(w2534, "_slopesOffset", ".has") -> (w2537:string)
                                n877 = Build Path(base path=w2533, name or relative path=w2537) -> (appended path=w2532:path)
                                n878 = call <userlib>:"LVClass_HasoSlopes Save.vi"("HasoSlopes in"=w2531, "path"=w2532) -> ()  [unwired: 12 in, 2 out]
                                }
                                frame #1 {
                                n879 = Concatenate Strings(w2540, "_zernOffset", ".txt") -> (w2543:string)
                                n880 = Build Path(base path=w2539, name or relative path=w2543) -> (appended path=w2544:path)
                                n881 = Array To Spreadsheet String(array=w2538, 3:"%f") -> (spreadsheet string=w2545:string)  [unwired: 1 in]
                                n882 = Write to Text File(file (use dialog)=w2544, text=w2545) -> ()  [unwired: 2 in, 3 out]
                                }
                                }
                                }
                              }
                              n883 = call <userlib>:"LVClasse_Phase GetStatisticDatas.vi"("Phase in"=w2511, "error in (no error)"=w2521) -> ("Phase out"=w2526:refnum<class "Phase.lvclass">, "StatisticsData"=w2507:T2, "error out"=w2524:errorcluster)  [unwired: 11 in]
                              n884 = local write "Phase statistics"(w2507) -> ()
                              n885 = call <userlib>:"LVClasse_Phase Get Data.vi"("Phase in"=w2526, "Pupil"=w2520, "error in (no error)"=w2524) -> ("Phase out"=w2522:refnum<class "Phase.lvclass">, "data"=w2508:sgl[][], "Pupil (dup)"=w2523:refnum<class "Pupil.lvclass">, "error out"=w2525:errorcluster)  [unwired: 9 in]
                              n886 = local write "Zernike Measured"(w2499) -> ()
                              n887 = local write "Phase values"(w2508) -> ()
                            }
                            frame Error {
                            }
                          }
                          n888 = call <userlib>:"LVClass_HasoSlopes dtor.vi"("HasoSlopes in"=w2458) -> ()  [unwired: 13 in, 2 out]
                        }
                      }
                    }
                  }
                  n889 = Unbundle By Name(w2425) -> ("status"=w2426:bool)
                }
              }
            }
          }
        }
      }
      event "Exit": Value Change {
        # "STOP AND EXIT"
        n890 = event-data() -> ()  [unwired: 1 in, 4 out]
        n891 = case shown="False" w2570 {
          tunnel: w2578 -> [w2581 w2584]
          tunnel: [errorcluster {"status"=FALSE, "code"=0, "source"=""} ("error out") w2583] -> w2577
          tunnel: [w2581 w2582] -> w2576
          frame False {
          }
          frame True {
            n892 = call <userlib>:"LVClass_Camera stop acquisition.vi"("Camera in"=w2584) -> ("Camera out"=w2582:refnum<class "Camera.lvclass">, "error out"=w2583:errorcluster)  [unwired: 13 in]
          }
        }
      }
      event Panel Close? {
        n893 = event-data() -> ()  [unwired: 1 in, 1 out]
        n894 = flat-sequence {
          tunnel: w2600 -> [w2606]
          tunnel: w2593 -> [w2603]
          tunnel: [w2605] -> w2586
          tunnel: [w2604] -> w2585
          tunnel: [w2608] -> w2598
          tunnel: [w2609] -> w2599
          tunnel: w2586 -> [w2609]
          tunnel: w2585 -> [w2608]
          frame #0 {
            n895 = call <userlib>:"LVClass_Camera stop acquisition.vi"("Camera in"=w2606, "error in (no error)"=w2603) -> ("Camera out"=w2605:refnum<class "Camera.lvclass">, "error out"=w2604:errorcluster)  [unwired: 12 in]
          }
          frame #1 {
            n896 = local write "HASO ready"(FALSE) -> ()
          }
        }
        n897 = event-data("Discard?"=TRUE) -> ()  [unwired: 1 in, 1 out]
      }
    }
    n898 = Wait (ms)(milliseconds to wait=u32 250) -> ()  [unwired: 1 out]
  }
  n899 = case shown="True" w25 {
    tunnel: w46 -> [_ w2634]
    tunnel: w45 -> [_ w2633]
    tunnel: w44 -> [_ w2632]
    tunnel: w43 -> [_ w2631]
    tunnel: w42 -> [_ w2630]
    tunnel: w41 -> [_ w2629]
    tunnel: w40 -> [_ w2628]
    tunnel: w10 -> [_ w2621]
    tunnel: w6 -> [_ w2620]
    tunnel: w5 -> [_ w2619]
    tunnel: w4 -> [_ w2618]
    tunnel: w2 -> [_ w2615]
    tunnel: w3 -> [_ w2610]
    frame False {
    }
    frame True {
      n900 = flat-sequence {
        tunnel: w2633 -> [w2671]
        tunnel: w2634 -> [w2669]
        tunnel: [w2671] -> w2648
        tunnel: w2628 -> [w2670]
        tunnel: [w2670] -> w2647
        tunnel: [w2669] -> w2646
        tunnel: w2632 -> [w2668]
        tunnel: w2631 -> [w2667]
        tunnel: w2630 -> [w2666]
        tunnel: w2629 -> [w2665]
        tunnel: [w2664] -> w2645
        tunnel: [w2663] -> w2644
        tunnel: [w2662] -> w2643
        tunnel: [w2661] -> w2642
        tunnel: [w2654] -> w2626
        tunnel: [w2655] -> w2624
        tunnel: [w2656] -> w2622
        tunnel: w2621 -> [w2660]
        tunnel: w2620 -> [w2659]
        tunnel: w2619 -> [w2658]
        tunnel: w2618 -> [w2657]
        tunnel: [w2653] -> w2616
        tunnel: w2615 -> [w2652]
        tunnel: [w2651] -> w2614
        tunnel: w2610 -> [w2650]
        tunnel: [w2650] -> w2611
        tunnel: w2648 -> [w2686]
        tunnel: w2647 -> [w2685]
        tunnel: w2646 -> [w2683]
        tunnel: [w2685] -> w2641
        tunnel: [w2684] -> w2640
        tunnel: [w2683] -> w2639
        tunnel: w2645 -> [w2682]
        tunnel: [w2682] -> w2638
        tunnel: w2644 -> [w2681]
        tunnel: [w2681] -> w2637
        tunnel: w2643 -> [w2680]
        tunnel: [w2680] -> w2636
        tunnel: w2642 -> [w2679]
        tunnel: [w2679] -> w2635
        tunnel: [w2678] -> w2627
        tunnel: w2626 -> [w2678]
        tunnel: [w2677] -> w2625
        tunnel: w2624 -> [w2677]
        tunnel: [w2676] -> w2623
        tunnel: w2622 -> [w2676]
        tunnel: [w2675] -> w2617
        tunnel: w2616 -> [w2675]
        tunnel: w2614 -> [w2674]
        tunnel: [w2674] -> w2613
        tunnel: [w2673] -> w2612
        tunnel: w2611 -> [w2672]
        tunnel: w2641 -> [w2702]
        tunnel: w2640 -> [w2700]
        tunnel: w2639 -> [w2699]
        tunnel: w2638 -> [w2698]
        tunnel: w2637 -> [w2697]
        tunnel: w2636 -> [w2696]
        tunnel: w2635 -> [w2695]
        tunnel: w2627 -> [w2693]
        tunnel: w2625 -> [w2692]
        tunnel: w2623 -> [w2691]
        tunnel: w2617 -> [w2690]
        tunnel: w2613 -> [w2689]
        tunnel: w2612 -> [w2688]
        frame #0 {
          n901 = call <userlib>:"LVClass_Image dtor.vi"("Image in"=w2667) -> ("error out"=w2663:errorcluster)  [unwired: 13 in, 1 out]
          n902 = local write "HASO ready"(FALSE) -> ()
          n903 = call <userlib>:"LVClass_HasoSlopes dtor.vi"("HasoSlopes in"=w2660) -> ("error out"=w2655:errorcluster)  [unwired: 13 in, 1 out]
          n904 = call <userlib>:"LVClass_Pupil dtor.vi"("Pupil in"=w2657) -> ("error out"=w2653:errorcluster)  [unwired: 13 in, 1 out]
          n905 = call <userlib>:"LVClass_Image dtor.vi"("Image in"=w2665) -> ("error out"=w2661:errorcluster)  [unwired: 13 in, 1 out]
          n906 = call <userlib>:"LVClass_WavefrontCorrector dtor.vi"("WavefrontCorrector in"=w2652) -> ("error out"=w2651:errorcluster)  [unwired: 13 in, 1 out]
          n907 = call <userlib>:"LVClass_Image dtor.vi"("Image in"=w2668) -> ("error out"=w2664:errorcluster)  [unwired: 13 in, 1 out]
          n908 = call <userlib>:"LVClass_Image dtor.vi"("Image in"=w2666) -> ("error out"=w2662:errorcluster)  [unwired: 13 in, 1 out]
          n909 = call <userlib>:"LVClass_HasoEngine dtor.vi"("HasoEngine in"=w2658) -> ("error out"=w2654:errorcluster)  [unwired: 13 in, 1 out]
          n910 = call <userlib>:"LVClasse_Phase dtor.vi"("Phase in"=w2659) -> ("error out"=w2656:errorcluster)  [unwired: 13 in, 1 out]
        }
        frame #1 {
          n911 = call <userlib>:"LVClass_Camera dtor.vi"("Camera in"=w2686) -> ("error out"=w2684:errorcluster)  [unwired: 13 in, 1 out]
          n912 = call <userlib>:"LVClass_WavefrontCorrectorSet dtor.vi"("WavefrontCorrectorSet in"=w2672) -> ("error out"=w2673:errorcluster)  [unwired: 13 in, 1 out]
        }
        frame #2 {
          n913 = call <userlib>:"LVClass_CameraSet dtor.vi"("CameraSet.lvclass"=w2702) -> ("error out"=w2701:errorcluster)  [unwired: 13 in, 1 out]
          n914 = local write "Current status"("Shut down") -> ()
          n915 = Merge Errors(w2701, w2700, w2699, w2698, w2697, w2696, w2695, w2691, w2692, w2693, w2690, w2689, w2688) -> (w2694:errorcluster)
          n916 = property on="Current error" class="Clust (strict)"("Value"=w2694) -> ()  [unwired: 2 in, 2 out]
        }
      }
    }
  }
